vi "Database.vi"() -> ()   [LabVIEW 2016]
panel:
  in  "Tree (Right)":string[](tree)=["PPMS 2\\PPMS 2 Temperature"]
  in  "Tree (Left)":string[](tree)=["MNK_18T\\1820_IPS_Level_He", "MNK_18T\\1820_IPS_Magnet_Field"]
  in  "max points per trace (all)":i32=-1
  in  "Tab Control":enum32{"Time Traces", "X-Y Plot (shitty)"}(tab)
  out "Database Trace":T1(graph) caption="Retrieved from Citadel 5"
  in  "Y Scale.Mapping Mode\n0 = linear; 1 = log":u8
  in  "Filter?":bool
  out "XY Graph":cluster{"data":dbl[], "data":dbl[]}(graph)
  in  "Tab Control 2":T2(tab)
  in  "DST":bool caption="Blank Button"
  in  "IP or PC Name":string="HousesOfTheHoly"
  in  "Span":dbl=3600.0 step=3600.0 format="%<%D d %H hr %M min %S s>t"
  in  "Which Database?":enum16{"HousesOfTheHoly", "Rambleon"}(ring)
  in  "Mode":T3(ring)=enum."Start, End, End - T"
  in  "Display the following network shared variables (left axis)":u16[](array[ring])=[194] items=["Attocube 3DR\\axis 1: Amplitude", "Attocube 3DR\\axis 1: Capacitance", "Attocube 3DR\\axis 1: control mode", "Attocube 3DR\\axis 1: current position", "Attocube 3DR\\axis 1: DCLevel", "Attocube 3DR\\axis 1: Frequency", "Attocube 3DR\\axis 1: moving", "Attocube 3DR\\axis 1: Output", "Attocube 3DR\\axis 1: rot. count", "Attocube 3DR\\axis 1: sensor disconnected", "Attocube 3DR\\axis 1: sensor error", "Attocube 3DR\\axis 1: Single Circle Mode", "Attocube 3DR\\axis 1: sp position", "Attocube 3DR\\axis 1: sp rot count", "Attocube 3DR\\axis 1: speed", "Attocube 3DR\\axis 1: StepWidth", "Attocube 3DR\\axis 1: stop detected", "Attocube 3DR\\axis 1: stop enable", "Attocube 3DR\\axis 1: Target GND", "Attocube 3DR\\axis 2: Amplitude", "Attocube 3DR\\axis 2: Capacitance", "Attocube 3DR\\axis 2: control mode", "Attocube 3DR\\axis 2: current position", "Attocube 3DR\\axis 2: DCLevel", "Attocube 3DR\\axis 2: Frequency", "Attocube 3DR\\axis 2: moving", "Attocube 3DR\\axis 2: Output", "Attocube 3DR\\axis 2: rot. count", "Attocube 3DR\\axis 2: sensor disconnected", "Attocube 3DR\\axis 2: sensor error", "Attocube 3DR\\axis 2: Single Circle Mode", "Attocube 3DR\\axis 2: sp position", "Attocube 3DR\\axis 2: sp rot count", "Attocube 3DR\\axis 2: speed", "Attocube 3DR\\axis 2: StepWidth", "Attocube 3DR\\axis 2: stop detected", "Attocube 3DR\\axis 2: stop enable", "Attocube 3DR\\axis 2: Target GND", "Attocube 3DR\\static amplitude", "Cypher\\Cypher RH1", "Cypher\\Cypher RH2", "Cypher\\Cypher Temperature", "Cypher\\Cypher_Funnel_Property", "Cypher\\Cypher_Path_Property", "Cypher\\Cypher_Rectangle_Property", "DR200\\DR200_Magnet_Field", "DR200\\DR200_Magnet_Field_Target", "DR200\\DR200_Magnet_PS_Current", "DR200\\DR200_Magnet_PS_Field", "DR200\\DR200_Magnet_PS_Voltage", "DR200\\DR200_Magnet_Rate_Target", "DR200\\DR200_Magnet_Status_Activity", "DR200\\DR200_Magnet_Status_Mode", "DR200\\DR200_Magnet_Status_Switch_Heater", "DR200\\DR200_Magnet_Status_System", "JLevy\\Levy 1", "Leiden CF900\\CF Impedance CMN", "Leiden CF900\\CF_FP_STATE", "Leiden CF900\\CF_KH_ch1", "Leiden CF900\\CF_KH_ch2", "Leiden CF900\\CF_KH_ch3", "Leiden CF900\\CF_KH_ch4", "Leiden CF900\\CF_KH_ch5", "Leiden CF900\\CF_KH_ch6", "Leiden CF900\\CF_KH_ch7", "Leiden CF900\\CF_KH_ch8", "Leiden CF900\\CF_TC_calibration", "Leiden CF900\\CF_TC_description", "Leiden CF900\\CF_TC_Z_calibration", "Leiden CF900\\CF_TC_Z_description", "Leiden CF900\\CF_TC_Z_R0", "Leiden CF900\\CF_TC_Z_R1", "Leiden CF900\\CF_TC_Z_R2", "Leiden CF900\\CF_TC_Z_R3", "Leiden CF900\\CF_TC_Z_R4", "Leiden CF900\\CF_TC_Z_R5", "Leiden CF900\\CF_TC_Z_R6", "Leiden CF900\\CF_TC_Z_R7", "Leiden CF900\\CF_TC_Z_R8", "Leiden CF900\\CF_TC_Z_R9", "Leiden CF900\\CF_TC_Z_T0", "Leiden CF900\\CF_TC_Z_T1", "Leiden CF900\\CF_TC_Z_T2", "Leiden CF900\\CF_TC_Z_T3", "Leiden CF900\\CF_TC_Z_T4", "Leiden CF900\\CF_TC_Z_T5", "Leiden CF900\\CF_TC_Z_T6", "Leiden CF900\\CF_TC_Z_T7", "Leiden CF900\\CF_TC_Z_T8", "Leiden CF900\\CF_TC_Z_T9", "Leiden CF900\\CF900_Cstill", "Leiden CF900\\Leiden CF FP\\CF FP Flow", "Leiden CF900\\Leiden CF FP\\CF FP He", "Leiden CF900\\Leiden CF FP\\CF FP MG0", "Leiden CF900\\Leiden CF FP\\CF FP MG1", "Leiden CF900\\Leiden CF FP\\CF FP MG2", "Leiden CF900\\Leiden CF FP\\CF FP MG3", "Leiden CF900\\Leiden CF FP\\CF FP MG4", "Leiden CF900\\Leiden CF FP\\CF FP MG5", "Leiden CF900\\Leiden CF FP\\CF FP oil", "Leiden CF900\\Leiden CF FP\\CF FP P_high", "Leiden CF900\\Leiden CF FP\\CF FP P_low", "Leiden CF900\\Leiden CF FP\\CF FP P1", "Leiden CF900\\Leiden CF FP\\CF FP P2", "Leiden CF900\\Leiden CF FP\\CF FP P3", "Leiden CF900\\Leiden CF FP\\CF FP P4", "Leiden CF900\\Leiden CF FP\\CF FP P5", "Leiden CF900\\Leiden CF FP\\CF FP P6", "Leiden CF900\\Leiden CF FP\\CF FP P7", "Leiden CF900\\Leiden CF FP\\CF FP PT current", "Leiden CF900\\Leiden CF FP\\CF FP PT on", "Leiden CF900\\Leiden CF FP\\CF FP State0", "Leiden CF900\\Leiden CF FP\\CF FP State1", "Leiden CF900\\Leiden CF FP\\CF FP State2", "Leiden CF900\\Leiden CF FP\\CF FP W_in", "Leiden CF900\\Leiden CF FP\\CF FP W_out", "Leiden CF900\\Leiden CF Impedance Bridge\\CF IB TA", "Leiden CF900\\Leiden CF Impedance Bridge\\CF IB TB", "Leiden CF900\\Leiden CF Impedance Bridge\\CF IB TC", "Leiden CF900\\Leiden CF Impedance Bridge\\CF IB TD", "Leiden CF900\\Leiden CF Impedance Bridge\\CF IB TE", "Leiden CF900\\Leiden CF Magnetic Field\\CF Field X", "Leiden CF900\\Leiden CF Magnetic Field\\CF Field Y", "Leiden CF900\\Leiden CF Magnetic Field\\CF Field Z", "Leiden CF900\\Leiden CF TC\\CF TC I0", "Leiden CF900\\Leiden CF TC\\CF TC I1", "Leiden CF900\\Leiden CF TC\\CF TC I2", "Leiden CF900\\Leiden CF TC\\CF TC I3", "Leiden CF900\\Leiden CF TC\\CF TC R0", "Leiden CF900\\Leiden CF TC\\CF TC R1", "Leiden CF900\\Leiden CF TC\\CF TC R2", "Leiden CF900\\Leiden CF TC\\CF TC R3", "Leiden CF900\\Leiden CF TC\\CF TC R4", "Leiden CF900\\Leiden CF TC\\CF TC R5", "Leiden CF900\\Leiden CF TC\\CF TC R6", "Leiden CF900\\Leiden CF TC\\CF TC R7", "Leiden CF900\\Leiden CF TC\\CF TC T0", "Leiden CF900\\Leiden CF TC\\CF TC T1", "Leiden CF900\\Leiden CF TC\\CF TC T2", "Leiden CF900\\Leiden CF TC\\CF TC T3", "Leiden CF900\\Leiden CF TC\\CF TC T4", "Leiden CF900\\Leiden CF TC\\CF TC T5", "Leiden CF900\\Leiden CF TC\\CF TC T6", "Leiden CF900\\Leiden CF TC\\CF TC T7", "Leiden CF900\\RuO2_T", "Leiden CF900\\RuO2_Z", "Leiden CF900\\Vbg", "Leiden CF900\\VRM VrmSweepMode", "Leiden CF900\\VRM VrmSweepRate", "Leiden CF900\\VRM VrmSweepTime", "Leiden CF900\\VRM VrmX setpT", "Leiden CF900\\VRM VrmY setpT", "Leiden CF900\\VRM VrmZ setpT", "Leiden CF900\\VRM X at rest", "Leiden CF900\\VRM X magA", "Leiden CF900\\VRM X magT", "Leiden CF900\\VRM X meas A", "Leiden CF900\\VRM X meas V", "Leiden CF900\\VRM X outA", "Leiden CF900\\VRM X outT", "Leiden CF900\\VRM X setpT", "Leiden CF900\\VRM X Status", "Leiden CF900\\VRM X sweep", "Leiden CF900\\VRM X sweep A", "Leiden CF900\\VRM Y at rest", "Leiden CF900\\VRM Y magA", "Leiden CF900\\VRM Y magT", "Leiden CF900\\VRM Y meas A", "Leiden CF900\\VRM Y meas V", "Leiden CF900\\VRM Y outA", "Leiden CF900\\VRM Y outT", "Leiden CF900\\VRM Y setpT", "Leiden CF900\\VRM Y Status", "Leiden CF900\\VRM Y sweep", "Leiden CF900\\VRM Y sweep A", "Leiden CF900\\VRM Z at rest", "Leiden CF900\\VRM Z magA", "Leiden CF900\\VRM Z magT", "Leiden CF900\\VRM Z meas A", "Leiden CF900\\VRM Z meas V", "Leiden CF900\\VRM Z outA", "Leiden CF900\\VRM Z outT", "Leiden CF900\\VRM Z setpT", "Leiden CF900\\VRM Z Status", "Leiden CF900\\VRM Z sweep", "Leiden CF900\\VRM Z sweep A", "MFP3D\\MFP3D Hum", "MFP3D\\MFP3D Temperature", "MFP3D\\MFP3D TSP01 Hum", "MFP3D\\MFP3D TSP01 Temperature", "MFP3D\\MFP3D User", "MNK_18T\\1820_IPS_Current", "MNK_18T\\1820_IPS_Level_He", "MNK_18T\\1820_IPS_Level_N2", "MNK_18T\\1820_IPS_M1_Current", "MNK_18T\\1820_IPS_M1_Voltage", "MNK_18T\\1820_IPS_M2_Current", "MNK_18T\\1820_IPS_M2_Voltage", "MNK_18T\\1820_IPS_M3_Current", "MNK_18T\\1820_IPS_M3_Voltage", "MNK_18T\\1820_IPS_Magnet_Field", "MNK_18T\\1820_IPS_Magnet_Temperature", "MNK_18T\\1820_IPS_Magnet_Temperature_R", "MNK_18T\\1820_IPS_PS_Field", "MNK_18T\\1820_IPS_Reply", "MNK_18T\\1820_IPS_Status", "MNK_18T\\1820_IPS_Switch", "MNK_18T\\1820_IPS_Target_Field", "MNK_18T\\1820_IPS_Target_Field_Rate", "MNK_18T\\1820_IPS_Voltage", "MNK_18T\\1820_ITC_Lambda_Status", "MNK_18T\\1820_ITC_Lambda_Temperature", "MNK_18T\\1820_ITC_Lambda_Temperature_R", "MNK_18T\\1820_ITC_Needle_Valve", "MNK_18T\\1820_ITC_Pressure", "MNK_18T\\1820_ITC_Reply", "MNK_18T\\KH_ch1", "MNK_18T\\KH_ch2", "MNK_18T\\KH_ch3", "MNK_18T\\KH_ch4", "MNK_18T\\KH_ch5", "MNK_18T\\KH_ch6", "MNK_18T\\KH_ch7", "MNK_18T\\KH_ch8", "MNK_18T\\Lockin_Results", "MNK_18T\\MNK_CMN-187_T", "MNK_18T\\MNK_CMN-187_Z", "MNK_18T\\MNK_Cstill_T", "MNK_18T\\MNK_Cstill_Z", "MNK_18T\\MNK_FP_Flow", "MNK_18T\\MNK_FP_MG0", "MNK_18T\\MNK_FP_MG1", "MNK_18T\\MNK_FP_MG2", "MNK_18T\\MNK_FP_MG3", "MNK_18T\\MNK_FP_MG4", "MNK_18T\\MNK_FP_MG5", "MNK_18T\\MNK_FP_P1", "MNK_18T\\MNK_FP_P2", "MNK_18T\\MNK_FP_P3", "MNK_18T\\MNK_FP_P4", "MNK_18T\\MNK_FP_P5", "MNK_18T\\MNK_FP_P6", "MNK_18T\\MNK_FP_P7", "MNK_18T\\MNK_FP_STATE", "MNK_18T\\MNK_FP_State0", "MNK_18T\\MNK_FP_State1", "MNK_18T\\MNK_FP_State2", "MNK_18T\\MNK_TC_calibration", "MNK_18T\\MNK_TC_description", "MNK_18T\\MNK_TC_I0", "MNK_18T\\MNK_TC_I1", "MNK_18T\\MNK_TC_I2", "MNK_18T\\MNK_TC_I3", "MNK_18T\\MNK_TC_R0", "MNK_18T\\MNK_TC_R1", "MNK_18T\\MNK_TC_R2", "MNK_18T\\MNK_TC_R3", "MNK_18T\\MNK_TC_R4", "MNK_18T\\MNK_TC_R5", "MNK_18T\\MNK_TC_R6", "MNK_18T\\MNK_TC_R7", "MNK_18T\\MNK_TC_T0", "MNK_18T\\MNK_TC_T1", "MNK_18T\\MNK_TC_T2", "MNK_18T\\MNK_TC_T3", "MNK_18T\\MNK_TC_T4", "MNK_18T\\MNK_TC_T5", "MNK_18T\\MNK_TC_T6", "MNK_18T\\MNK_TC_T7", "MNK_18T\\MNK_TC_Z_calibration", "MNK_18T\\MNK_TC_Z_description", "MNK_18T\\OSC_config", "MNK_18T\\Vbg", "Montana THZ 1\\THZ 1 Dew Point", "Montana THZ 1\\THZ 1 Humidity", "Montana THZ 1\\THZ 1 Temperature", "OneNote API HTTP\\Access Token 0000000048124379", "OneNote API HTTP\\Asana Access Token 15669051163913", "PPMS 1\\PPMS 1 Magnetic Field", "PPMS 1\\PPMS 1 Temperature", "PPMS 2\\PPMS 2 Flow Rate", "PPMS 2\\PPMS 2 Helium Level", "PPMS 2\\PPMS 2 Magnetic Field", "PPMS 2\\PPMS 2 Position", "PPMS 2\\PPMS 2 Sys Pressure", "PPMS 2\\PPMS 2 Temperature", "PPMS 2\\PPMS 2 Vbg", "PPMS2\\PPMS2 Annulus Pres (Torr)", "PPMS2\\PPMS2 Annulus Vacuum (V)", "PPMS2\\PPMS2 Block Htr Cur (mA)", "PPMS2\\PPMS2 Block Htr Pwr (W)", "PPMS2\\PPMS2 BlockHeater(Ohm)", "PPMS2\\PPMS2 Bridge 1 Excitation (uA)", "PPMS2\\PPMS2 Bridge 1 Resistance (ohms)", "PPMS2\\PPMS2 Bridge 2 Excitation (uA)", "PPMS2\\PPMS2 Bridge 2 Resistance (ohms)", "PPMS2\\PPMS2 Bridge 3 Excitation (uA)", "PPMS2\\PPMS2 Bridge 3 Resistance (ohms)", "PPMS2\\PPMS2 Bridge 4 Excitation (uA)", "PPMS2\\PPMS2 Bridge 4 Resistance (ohms)", "PPMS2\\PPMS2 CIG Cernox (K)", "PPMS2\\PPMS2 CIG Excit (uA)", "PPMS2\\PPMS2 Comment", "PPMS2\\PPMS2 DAC  I  (cnts)", "PPMS2\\PPMS2 Digital Inputs (code)", "PPMS2\\PPMS2 Drive 1 Iout (mA)", "PPMS2\\PPMS2 Drive 1 Ipower (watts)", "PPMS2\\PPMS2 Drive 2 Iout (mA)", "PPMS2\\PPMS2 Drive 2 Ipower (watts)", "PPMS2\\PPMS2 EXT Flow (L min)", "PPMS2\\PPMS2 Flapper state", "PPMS2\\PPMS2 Flow Rate (l min)", "PPMS2\\PPMS2 He Level ()", "PPMS2\\PPMS2 Hi res (A) read", "PPMS2\\PPMS2 High Vacuum mode", "PPMS2\\PPMS2 Hires enable", "PPMS2\\PPMS2 Impedance (mode)", "PPMS2\\PPMS2 iso flag", "PPMS2\\PPMS2 KRPMs", "PPMS2\\PPMS2 Last 2 eng st", "PPMS2\\PPMS2 Log", "PPMS2\\PPMS2 Mag (V) read", "PPMS2\\PPMS2 Mag (V) set", "PPMS2\\PPMS2 Mag adj sc(I)set", "PPMS2\\PPMS2 Magnet (Oe)", "PPMS2\\PPMS2 Magnetic Field (Oe)", "PPMS2\\PPMS2 Map 20 ()", "PPMS2\\PPMS2 Map 21 ()", "PPMS2\\PPMS2 Map 22 ()", "PPMS2\\PPMS2 Map 23 ()", "PPMS2\\PPMS2 Map 24 ()", "PPMS2\\PPMS2 Map 25 ()", "PPMS2\\PPMS2 Map 26 ()", "PPMS2\\PPMS2 Map 27 ()", "PPMS2\\PPMS2 Map 28 ()", "PPMS2\\PPMS2 Map 29 ()", "PPMS2\\PPMS2 Map 67 ()", "PPMS2\\PPMS2 Map 68 ()", "PPMS2\\PPMS2 Map 69 ()", "PPMS2\\PPMS2 Map 89 ()", "PPMS2\\PPMS2 Map 90 ()", "PPMS2\\PPMS2 Map 91 ()", "PPMS2\\PPMS2 Map 92 ()", "PPMS2\\PPMS2 Map 93 ()", "PPMS2\\PPMS2 Neck Excit (uA)", "PPMS2\\PPMS2 Neck Htr Cur (mA)", "PPMS2\\PPMS2 Neck Htr Pwr (W)", "PPMS2\\PPMS2 Neck Therm (K)", "PPMS2\\PPMS2 NeckHeater(Ohm)", "PPMS2\\PPMS2 Plat Excit (uA)", "PPMS2\\PPMS2 Plat Therm (K)", "PPMS2\\PPMS2 Pressure ()", "PPMS2\\PPMS2 PSU Field (Oe)", "PPMS2\\PPMS2 Pump power (W)", "PPMS2\\PPMS2 Pump temp (C)", "PPMS2\\PPMS2 Redirected 55 ()", "PPMS2\\PPMS2 Redirected 56 ()", "PPMS2\\PPMS2 Redirected 57 ()", "PPMS2\\PPMS2 Redirected 58 ()", "PPMS2\\PPMS2 Redirected 59 ()", "PPMS2\\PPMS2 Redirected 61 ()", "PPMS2\\PPMS2 Regen htr flag", "PPMS2\\PPMS2 Sample Position (deg)", "PPMS2\\PPMS2 Seq Stat ()", "PPMS2\\PPMS2 Setpoint (K)", "PPMS2\\PPMS2 Signal 1 Vin (V)", "PPMS2\\PPMS2 Signal 2 Vin (V)", "PPMS2\\PPMS2 Spare Excit (uA)", "PPMS2\\PPMS2 Spare Therm (K)", "PPMS2\\PPMS2 Status (code)", "PPMS2\\PPMS2 Sw heater state", "PPMS2\\PPMS2 Sys Temp ()", "PPMS2\\PPMS2 System Pres (Torr)", "PPMS2\\PPMS2 System Status (code)", "PPMS2\\PPMS2 Tableless Map53 ()", "PPMS2\\PPMS2 Tableless Map54 ()", "PPMS2\\PPMS2 Temperature (K)", "PPMS2\\PPMS2 Therm v", "PPMS2\\PPMS2 Time Stamp (sec)", "PPMS2\\PPMS2 Valve Position (deg)", "PPMSDR\\PPMSDR Annulus Pres (Torr)", "PPMSDR\\PPMSDR Annulus Vacuum (V)", "PPMSDR\\PPMSDR Block Htr Cur (mA)", "PPMSDR\\PPMSDR Block Htr Pwr (W)", "PPMSDR\\PPMSDR BlockHeater(Ohm)", "PPMSDR\\PPMSDR Bridge 1 Excitation (uA)", "PPMSDR\\PPMSDR Bridge 1 Resistance (ohms)", "PPMSDR\\PPMSDR Bridge 2 Excitation (uA)", "PPMSDR\\PPMSDR Bridge 2 Resistance (ohms)", "PPMSDR\\PPMSDR Bridge 3 Excitation (uA)", "PPMSDR\\PPMSDR Bridge 3 Resistance (ohms)", "PPMSDR\\PPMSDR Bridge 4 Excitation (uA)", "PPMSDR\\PPMSDR Bridge 4 Resistance (ohms)", "PPMSDR\\PPMSDR CIG Cernox (K)", "PPMSDR\\PPMSDR CIG Excit (uA)", "PPMSDR\\PPMSDR Comment", "PPMSDR\\PPMSDR DAC  I  (cnts)", "PPMSDR\\PPMSDR Digital Inputs (code)", "PPMSDR\\PPMSDR Drive 1 Iout (mA)", "PPMSDR\\PPMSDR Drive 1 Ipower (watts)", "PPMSDR\\PPMSDR Drive 2 Iout (mA)", "PPMSDR\\PPMSDR Drive 2 Ipower (watts)", "PPMSDR\\PPMSDR EXT Flow (L min)", "PPMSDR\\PPMSDR Flapper state", "PPMSDR\\PPMSDR Flow Rate (l min)", "PPMSDR\\PPMSDR He Level ()", "PPMSDR\\PPMSDR Hi res (A) read", "PPMSDR\\PPMSDR High Vacuum mode", "PPMSDR\\PPMSDR Hires enable", "PPMSDR\\PPMSDR Impedance (mode)", "PPMSDR\\PPMSDR iso flag", "PPMSDR\\PPMSDR KRPMs", "PPMSDR\\PPMSDR Last 2 eng st", "PPMSDR\\PPMSDR Log", "PPMSDR\\PPMSDR low res (A) read", "PPMSDR\\PPMSDR Mag (V) read", "PPMSDR\\PPMSDR Mag (V) set", "PPMSDR\\PPMSDR Mag adj sc(I)set", "PPMSDR\\PPMSDR Magnet (Oe)", "PPMSDR\\PPMSDR Magnetic Field (Oe)", "PPMSDR\\PPMSDR MAP 1", "PPMSDR\\PPMSDR MAP 10", "PPMSDR\\PPMSDR MAP 11", "PPMSDR\\PPMSDR MAP 12", "PPMSDR\\PPMSDR MAP 13", "PPMSDR\\PPMSDR MAP 14", "PPMSDR\\PPMSDR MAP 15", "PPMSDR\\PPMSDR MAP 16", "PPMSDR\\PPMSDR MAP 17", "PPMSDR\\PPMSDR MAP 18", "PPMSDR\\PPMSDR MAP 19", "PPMSDR\\PPMSDR MAP 2", "PPMSDR\\PPMSDR MAP 20", "PPMSDR\\PPMSDR Map 20 ()", "PPMSDR\\PPMSDR MAP 21", "PPMSDR\\PPMSDR Map 21 ()", "PPMSDR\\PPMSDR MAP 22", "PPMSDR\\PPMSDR Map 22 ()", "PPMSDR\\PPMSDR MAP 23", "PPMSDR\\PPMSDR Map 23 ()", "PPMSDR\\PPMSDR MAP 24", "PPMSDR\\PPMSDR Map 24 ()", "PPMSDR\\PPMSDR MAP 25", "PPMSDR\\PPMSDR Map 25 ()", "PPMSDR\\PPMSDR MAP 26", "PPMSDR\\PPMSDR Map 26 ()", "PPMSDR\\PPMSDR MAP 27", "PPMSDR\\PPMSDR Map 27 ()", "PPMSDR\\PPMSDR MAP 28", "PPMSDR\\PPMSDR Map 28 ()", "PPMSDR\\PPMSDR MAP 29", "PPMSDR\\PPMSDR Map 29 ()", "PPMSDR\\PPMSDR MAP 3", "PPMSDR\\PPMSDR MAP 30", "PPMSDR\\PPMSDR MAP 4", "PPMSDR\\PPMSDR MAP 5", "PPMSDR\\PPMSDR MAP 6", "PPMSDR\\PPMSDR Map 67 ()", "PPMSDR\\PPMSDR Map 68 ()", "PPMSDR\\PPMSDR Map 69 ()", "PPMSDR\\PPMSDR MAP 7", "PPMSDR\\PPMSDR MAP 8", "PPMSDR\\PPMSDR Map 89 ()", "PPMSDR\\PPMSDR MAP 9", "PPMSDR\\PPMSDR Map 90 ()", "PPMSDR\\PPMSDR Map 91 ()", "PPMSDR\\PPMSDR Map 92 ()", "PPMSDR\\PPMSDR Map 93 ()", "PPMSDR\\PPMSDR Neck Excit (uA)", "PPMSDR\\PPMSDR Neck Htr Cur (mA)", "PPMSDR\\PPMSDR Neck Htr Pwr (W)", "PPMSDR\\PPMSDR Neck Therm (K)", "PPMSDR\\PPMSDR NeckHeater(Ohm)", "PPMSDR\\PPMSDR Plat Excit (uA)", "PPMSDR\\PPMSDR Plat Therm (K)", "PPMSDR\\PPMSDR Pressure ()", "PPMSDR\\PPMSDR Pump power (W)", "PPMSDR\\PPMSDR Pump temp (C)", "PPMSDR\\PPMSDR Redirected 55 ()", "PPMSDR\\PPMSDR Redirected 56 ()", "PPMSDR\\PPMSDR Redirected 57 ()", "PPMSDR\\PPMSDR Redirected 58 ()", "PPMSDR\\PPMSDR Redirected 59 ()", "PPMSDR\\PPMSDR Redirected 61 ()", "PPMSDR\\PPMSDR Regen htr flag", "PPMSDR\\PPMSDR Sample Position (deg)", "PPMSDR\\PPMSDR Seq Stat ()", "PPMSDR\\PPMSDR Setpoint (K)", "PPMSDR\\PPMSDR Signal 1 Vin (V)", "PPMSDR\\PPMSDR Signal 2 Vin (V)", "PPMSDR\\PPMSDR Spare Excit (uA)", "PPMSDR\\PPMSDR Spare Therm (K)", "PPMSDR\\PPMSDR Status (code)", "PPMSDR\\PPMSDR Sw heater state", "PPMSDR\\PPMSDR Sys Temp ()", "PPMSDR\\PPMSDR System Pres (Torr)", "PPMSDR\\PPMSDR System Status (code)", "PPMSDR\\PPMSDR Tableless Map53 ()", "PPMSDR\\PPMSDR Tableless Map54 ()", "PPMSDR\\PPMSDR Temperature (K)", "PPMSDR\\PPMSDR Therm v", "PPMSDR\\PPMSDR Time Stamp (sec)", "PPMSDR\\PPMSDR Valve Position (deg)", "Sample Characterization\\2G Conductance", "Sample Characterization\\4G", "Sample Characterization\\4R", "Sample Characterization\\CURRENT", "Sample Characterization\\Experiment ID", "Sample Characterization\\Notes", "Sample Characterization\\OSCILLATION VOLTAGE", "Sample Characterization\\Sample Name", "Sample Characterization\\V1", "Sample Characterization\\V2", "SPM\\Laser Power", "SPM\\SPM scanner X", "SPM\\SPM scanner Y", "TEMPerHUM\\MFP : Humidity", "TEMPerHUM\\MFP : ID", "TEMPerHUM\\MFP : Location", "TEMPerHUM\\MFP : Picture URL", "TEMPerHUM\\MFP : Temperature", "TEMPerHUM\\MFP-3D : Humidity", "TEMPerHUM\\MFP-3D : ID", "TEMPerHUM\\MFP-3D : Location", "TEMPerHUM\\MFP-3D : Picture URL", "TEMPerHUM\\MFP-3D : Temperature", "TEMPerHUM\\TEST3 : Humidity", "TEMPerHUM\\TEST3 : ID", "TEMPerHUM\\TEST3 : Location", "TEMPerHUM\\TEST3 : Picture URL", "TEMPerHUM\\TEST3 : Temperature"]
  in  "Display the following network shared variables (right axis)":u16[](array[ring])=[192] items=["Attocube 3DR\\axis 1: Amplitude", "Attocube 3DR\\axis 1: Capacitance", "Attocube 3DR\\axis 1: control mode", "Attocube 3DR\\axis 1: current position", "Attocube 3DR\\axis 1: DCLevel", "Attocube 3DR\\axis 1: Frequency", "Attocube 3DR\\axis 1: moving", "Attocube 3DR\\axis 1: Output", "Attocube 3DR\\axis 1: rot. count", "Attocube 3DR\\axis 1: sensor disconnected", "Attocube 3DR\\axis 1: sensor error", "Attocube 3DR\\axis 1: Single Circle Mode", "Attocube 3DR\\axis 1: sp position", "Attocube 3DR\\axis 1: sp rot count", "Attocube 3DR\\axis 1: speed", "Attocube 3DR\\axis 1: StepWidth", "Attocube 3DR\\axis 1: stop detected", "Attocube 3DR\\axis 1: stop enable", "Attocube 3DR\\axis 1: Target GND", "Attocube 3DR\\axis 2: Amplitude", "Attocube 3DR\\axis 2: Capacitance", "Attocube 3DR\\axis 2: control mode", "Attocube 3DR\\axis 2: current position", "Attocube 3DR\\axis 2: DCLevel", "Attocube 3DR\\axis 2: Frequency", "Attocube 3DR\\axis 2: moving", "Attocube 3DR\\axis 2: Output", "Attocube 3DR\\axis 2: rot. count", "Attocube 3DR\\axis 2: sensor disconnected", "Attocube 3DR\\axis 2: sensor error", "Attocube 3DR\\axis 2: Single Circle Mode", "Attocube 3DR\\axis 2: sp position", "Attocube 3DR\\axis 2: sp rot count", "Attocube 3DR\\axis 2: speed", "Attocube 3DR\\axis 2: StepWidth", "Attocube 3DR\\axis 2: stop detected", "Attocube 3DR\\axis 2: stop enable", "Attocube 3DR\\axis 2: Target GND", "Attocube 3DR\\static amplitude", "Cypher\\Cypher RH1", "Cypher\\Cypher RH2", "Cypher\\Cypher Temperature", "Cypher\\Cypher_Funnel_Property", "Cypher\\Cypher_Path_Property", "Cypher\\Cypher_Rectangle_Property", "DR200\\DR200_Magnet_Field", "DR200\\DR200_Magnet_Field_Target", "DR200\\DR200_Magnet_PS_Current", "DR200\\DR200_Magnet_PS_Field", "DR200\\DR200_Magnet_PS_Voltage", "DR200\\DR200_Magnet_Rate_Target", "DR200\\DR200_Magnet_Status_Activity", "DR200\\DR200_Magnet_Status_Mode", "DR200\\DR200_Magnet_Status_Switch_Heater", "DR200\\DR200_Magnet_Status_System", "JLevy\\Levy 1", "Leiden CF900\\CF Impedance CMN", "Leiden CF900\\CF_FP_STATE", "Leiden CF900\\CF_KH_ch1", "Leiden CF900\\CF_KH_ch2", "Leiden CF900\\CF_KH_ch3", "Leiden CF900\\CF_KH_ch4", "Leiden CF900\\CF_KH_ch5", "Leiden CF900\\CF_KH_ch6", "Leiden CF900\\CF_KH_ch7", "Leiden CF900\\CF_KH_ch8", "Leiden CF900\\CF_TC_calibration", "Leiden CF900\\CF_TC_description", "Leiden CF900\\CF_TC_Z_calibration", "Leiden CF900\\CF_TC_Z_description", "Leiden CF900\\CF_TC_Z_R0", "Leiden CF900\\CF_TC_Z_R1", "Leiden CF900\\CF_TC_Z_R2", "Leiden CF900\\CF_TC_Z_R3", "Leiden CF900\\CF_TC_Z_R4", "Leiden CF900\\CF_TC_Z_R5", "Leiden CF900\\CF_TC_Z_R6", "Leiden CF900\\CF_TC_Z_R7", "Leiden CF900\\CF_TC_Z_R8", "Leiden CF900\\CF_TC_Z_R9", "Leiden CF900\\CF_TC_Z_T0", "Leiden CF900\\CF_TC_Z_T1", "Leiden CF900\\CF_TC_Z_T2", "Leiden CF900\\CF_TC_Z_T3", "Leiden CF900\\CF_TC_Z_T4", "Leiden CF900\\CF_TC_Z_T5", "Leiden CF900\\CF_TC_Z_T6", "Leiden CF900\\CF_TC_Z_T7", "Leiden CF900\\CF_TC_Z_T8", "Leiden CF900\\CF_TC_Z_T9", "Leiden CF900\\CF900_Cstill", "Leiden CF900\\Leiden CF FP\\CF FP Flow", "Leiden CF900\\Leiden CF FP\\CF FP He", "Leiden CF900\\Leiden CF FP\\CF FP MG0", "Leiden CF900\\Leiden CF FP\\CF FP MG1", "Leiden CF900\\Leiden CF FP\\CF FP MG2", "Leiden CF900\\Leiden CF FP\\CF FP MG3", "Leiden CF900\\Leiden CF FP\\CF FP MG4", "Leiden CF900\\Leiden CF FP\\CF FP MG5", "Leiden CF900\\Leiden CF FP\\CF FP oil", "Leiden CF900\\Leiden CF FP\\CF FP P_high", "Leiden CF900\\Leiden CF FP\\CF FP P_low", "Leiden CF900\\Leiden CF FP\\CF FP P1", "Leiden CF900\\Leiden CF FP\\CF FP P2", "Leiden CF900\\Leiden CF FP\\CF FP P3", "Leiden CF900\\Leiden CF FP\\CF FP P4", "Leiden CF900\\Leiden CF FP\\CF FP P5", "Leiden CF900\\Leiden CF FP\\CF FP P6", "Leiden CF900\\Leiden CF FP\\CF FP P7", "Leiden CF900\\Leiden CF FP\\CF FP PT current", "Leiden CF900\\Leiden CF FP\\CF FP PT on", "Leiden CF900\\Leiden CF FP\\CF FP State0", "Leiden CF900\\Leiden CF FP\\CF FP State1", "Leiden CF900\\Leiden CF FP\\CF FP State2", "Leiden CF900\\Leiden CF FP\\CF FP W_in", "Leiden CF900\\Leiden CF FP\\CF FP W_out", "Leiden CF900\\Leiden CF Impedance Bridge\\CF IB TA", "Leiden CF900\\Leiden CF Impedance Bridge\\CF IB TB", "Leiden CF900\\Leiden CF Impedance Bridge\\CF IB TC", "Leiden CF900\\Leiden CF Impedance Bridge\\CF IB TD", "Leiden CF900\\Leiden CF Impedance Bridge\\CF IB TE", "Leiden CF900\\Leiden CF Magnetic Field\\CF Field X", "Leiden CF900\\Leiden CF Magnetic Field\\CF Field Y", "Leiden CF900\\Leiden CF Magnetic Field\\CF Field Z", "Leiden CF900\\Leiden CF TC\\CF TC I0", "Leiden CF900\\Leiden CF TC\\CF TC I1", "Leiden CF900\\Leiden CF TC\\CF TC I2", "Leiden CF900\\Leiden CF TC\\CF TC I3", "Leiden CF900\\Leiden CF TC\\CF TC R0", "Leiden CF900\\Leiden CF TC\\CF TC R1", "Leiden CF900\\Leiden CF TC\\CF TC R2", "Leiden CF900\\Leiden CF TC\\CF TC R3", "Leiden CF900\\Leiden CF TC\\CF TC R4", "Leiden CF900\\Leiden CF TC\\CF TC R5", "Leiden CF900\\Leiden CF TC\\CF TC R6", "Leiden CF900\\Leiden CF TC\\CF TC R7", "Leiden CF900\\Leiden CF TC\\CF TC T0", "Leiden CF900\\Leiden CF TC\\CF TC T1", "Leiden CF900\\Leiden CF TC\\CF TC T2", "Leiden CF900\\Leiden CF TC\\CF TC T3", "Leiden CF900\\Leiden CF TC\\CF TC T4", "Leiden CF900\\Leiden CF TC\\CF TC T5", "Leiden CF900\\Leiden CF TC\\CF TC T6", "Leiden CF900\\Leiden CF TC\\CF TC T7", "Leiden CF900\\RuO2_T", "Leiden CF900\\RuO2_Z", "Leiden CF900\\Vbg", "Leiden CF900\\VRM VrmSweepMode", "Leiden CF900\\VRM VrmSweepRate", "Leiden CF900\\VRM VrmSweepTime", "Leiden CF900\\VRM VrmX setpT", "Leiden CF900\\VRM VrmY setpT", "Leiden CF900\\VRM VrmZ setpT", "Leiden CF900\\VRM X at rest", "Leiden CF900\\VRM X magA", "Leiden CF900\\VRM X magT", "Leiden CF900\\VRM X meas A", "Leiden CF900\\VRM X meas V", "Leiden CF900\\VRM X outA", "Leiden CF900\\VRM X outT", "Leiden CF900\\VRM X setpT", "Leiden CF900\\VRM X Status", "Leiden CF900\\VRM X sweep", "Leiden CF900\\VRM X sweep A", "Leiden CF900\\VRM Y at rest", "Leiden CF900\\VRM Y magA", "Leiden CF900\\VRM Y magT", "Leiden CF900\\VRM Y meas A", "Leiden CF900\\VRM Y meas V", "Leiden CF900\\VRM Y outA", "Leiden CF900\\VRM Y outT", "Leiden CF900\\VRM Y setpT", "Leiden CF900\\VRM Y Status", "Leiden CF900\\VRM Y sweep", "Leiden CF900\\VRM Y sweep A", "Leiden CF900\\VRM Z at rest", "Leiden CF900\\VRM Z magA", "Leiden CF900\\VRM Z magT", "Leiden CF900\\VRM Z meas A", "Leiden CF900\\VRM Z meas V", "Leiden CF900\\VRM Z outA", "Leiden CF900\\VRM Z outT", "Leiden CF900\\VRM Z setpT", "Leiden CF900\\VRM Z Status", "Leiden CF900\\VRM Z sweep", "Leiden CF900\\VRM Z sweep A", "MFP3D\\MFP3D Hum", "MFP3D\\MFP3D Temperature", "MFP3D\\MFP3D TSP01 Hum", "MFP3D\\MFP3D TSP01 Temperature", "MFP3D\\MFP3D User", "MNK_18T\\1820_IPS_Current", "MNK_18T\\1820_IPS_Level_He", "MNK_18T\\1820_IPS_Level_N2", "MNK_18T\\1820_IPS_M1_Current", "MNK_18T\\1820_IPS_M1_Voltage", "MNK_18T\\1820_IPS_M2_Current", "MNK_18T\\1820_IPS_M2_Voltage", "MNK_18T\\1820_IPS_M3_Current", "MNK_18T\\1820_IPS_M3_Voltage", "MNK_18T\\1820_IPS_Magnet_Field", "MNK_18T\\1820_IPS_Magnet_Temperature", "MNK_18T\\1820_IPS_Magnet_Temperature_R", "MNK_18T\\1820_IPS_PS_Field", "MNK_18T\\1820_IPS_Reply", "MNK_18T\\1820_IPS_Status", "MNK_18T\\1820_IPS_Switch", "MNK_18T\\1820_IPS_Target_Field", "MNK_18T\\1820_IPS_Target_Field_Rate", "MNK_18T\\1820_IPS_Voltage", "MNK_18T\\1820_ITC_Lambda_Status", "MNK_18T\\1820_ITC_Lambda_Temperature", "MNK_18T\\1820_ITC_Lambda_Temperature_R", "MNK_18T\\1820_ITC_Needle_Valve", "MNK_18T\\1820_ITC_Pressure", "MNK_18T\\1820_ITC_Reply", "MNK_18T\\KH_ch1", "MNK_18T\\KH_ch2", "MNK_18T\\KH_ch3", "MNK_18T\\KH_ch4", "MNK_18T\\KH_ch5", "MNK_18T\\KH_ch6", "MNK_18T\\KH_ch7", "MNK_18T\\KH_ch8", "MNK_18T\\Lockin_Results", "MNK_18T\\MNK_CMN-187_T", "MNK_18T\\MNK_CMN-187_Z", "MNK_18T\\MNK_Cstill_T", "MNK_18T\\MNK_Cstill_Z", "MNK_18T\\MNK_FP_Flow", "MNK_18T\\MNK_FP_MG0", "MNK_18T\\MNK_FP_MG1", "MNK_18T\\MNK_FP_MG2", "MNK_18T\\MNK_FP_MG3", "MNK_18T\\MNK_FP_MG4", "MNK_18T\\MNK_FP_MG5", "MNK_18T\\MNK_FP_P1", "MNK_18T\\MNK_FP_P2", "MNK_18T\\MNK_FP_P3", "MNK_18T\\MNK_FP_P4", "MNK_18T\\MNK_FP_P5", "MNK_18T\\MNK_FP_P6", "MNK_18T\\MNK_FP_P7", "MNK_18T\\MNK_FP_STATE", "MNK_18T\\MNK_FP_State0", "MNK_18T\\MNK_FP_State1", "MNK_18T\\MNK_FP_State2", "MNK_18T\\MNK_TC_calibration", "MNK_18T\\MNK_TC_description", "MNK_18T\\MNK_TC_I0", "MNK_18T\\MNK_TC_I1", "MNK_18T\\MNK_TC_I2", "MNK_18T\\MNK_TC_I3", "MNK_18T\\MNK_TC_R0", "MNK_18T\\MNK_TC_R1", "MNK_18T\\MNK_TC_R2", "MNK_18T\\MNK_TC_R3", "MNK_18T\\MNK_TC_R4", "MNK_18T\\MNK_TC_R5", "MNK_18T\\MNK_TC_R6", "MNK_18T\\MNK_TC_R7", "MNK_18T\\MNK_TC_T0", "MNK_18T\\MNK_TC_T1", "MNK_18T\\MNK_TC_T2", "MNK_18T\\MNK_TC_T3", "MNK_18T\\MNK_TC_T4", "MNK_18T\\MNK_TC_T5", "MNK_18T\\MNK_TC_T6", "MNK_18T\\MNK_TC_T7", "MNK_18T\\MNK_TC_Z_calibration", "MNK_18T\\MNK_TC_Z_description", "MNK_18T\\OSC_config", "MNK_18T\\Vbg", "Montana THZ 1\\THZ 1 Dew Point", "Montana THZ 1\\THZ 1 Humidity", "Montana THZ 1\\THZ 1 Temperature", "OneNote API HTTP\\Access Token 0000000048124379", "OneNote API HTTP\\Asana Access Token 15669051163913", "PPMS 1\\PPMS 1 Magnetic Field", "PPMS 1\\PPMS 1 Temperature", "PPMS 2\\PPMS 2 Flow Rate", "PPMS 2\\PPMS 2 Helium Level", "PPMS 2\\PPMS 2 Magnetic Field", "PPMS 2\\PPMS 2 Position", "PPMS 2\\PPMS 2 Sys Pressure", "PPMS 2\\PPMS 2 Temperature", "PPMS 2\\PPMS 2 Vbg", "PPMS2\\PPMS2 Annulus Pres (Torr)", "PPMS2\\PPMS2 Annulus Vacuum (V)", "PPMS2\\PPMS2 Block Htr Cur (mA)", "PPMS2\\PPMS2 Block Htr Pwr (W)", "PPMS2\\PPMS2 BlockHeater(Ohm)", "PPMS2\\PPMS2 Bridge 1 Excitation (uA)", "PPMS2\\PPMS2 Bridge 1 Resistance (ohms)", "PPMS2\\PPMS2 Bridge 2 Excitation (uA)", "PPMS2\\PPMS2 Bridge 2 Resistance (ohms)", "PPMS2\\PPMS2 Bridge 3 Excitation (uA)", "PPMS2\\PPMS2 Bridge 3 Resistance (ohms)", "PPMS2\\PPMS2 Bridge 4 Excitation (uA)", "PPMS2\\PPMS2 Bridge 4 Resistance (ohms)", "PPMS2\\PPMS2 CIG Cernox (K)", "PPMS2\\PPMS2 CIG Excit (uA)", "PPMS2\\PPMS2 Comment", "PPMS2\\PPMS2 DAC  I  (cnts)", "PPMS2\\PPMS2 Digital Inputs (code)", "PPMS2\\PPMS2 Drive 1 Iout (mA)", "PPMS2\\PPMS2 Drive 1 Ipower (watts)", "PPMS2\\PPMS2 Drive 2 Iout (mA)", "PPMS2\\PPMS2 Drive 2 Ipower (watts)", "PPMS2\\PPMS2 EXT Flow (L min)", "PPMS2\\PPMS2 Flapper state", "PPMS2\\PPMS2 Flow Rate (l min)", "PPMS2\\PPMS2 He Level ()", "PPMS2\\PPMS2 Hi res (A) read", "PPMS2\\PPMS2 High Vacuum mode", "PPMS2\\PPMS2 Hires enable", "PPMS2\\PPMS2 Impedance (mode)", "PPMS2\\PPMS2 iso flag", "PPMS2\\PPMS2 KRPMs", "PPMS2\\PPMS2 Last 2 eng st", "PPMS2\\PPMS2 Log", "PPMS2\\PPMS2 Mag (V) read", "PPMS2\\PPMS2 Mag (V) set", "PPMS2\\PPMS2 Mag adj sc(I)set", "PPMS2\\PPMS2 Magnet (Oe)", "PPMS2\\PPMS2 Magnetic Field (Oe)", "PPMS2\\PPMS2 Map 20 ()", "PPMS2\\PPMS2 Map 21 ()", "PPMS2\\PPMS2 Map 22 ()", "PPMS2\\PPMS2 Map 23 ()", "PPMS2\\PPMS2 Map 24 ()", "PPMS2\\PPMS2 Map 25 ()", "PPMS2\\PPMS2 Map 26 ()", "PPMS2\\PPMS2 Map 27 ()", "PPMS2\\PPMS2 Map 28 ()", "PPMS2\\PPMS2 Map 29 ()", "PPMS2\\PPMS2 Map 67 ()", "PPMS2\\PPMS2 Map 68 ()", "PPMS2\\PPMS2 Map 69 ()", "PPMS2\\PPMS2 Map 89 ()", "PPMS2\\PPMS2 Map 90 ()", "PPMS2\\PPMS2 Map 91 ()", "PPMS2\\PPMS2 Map 92 ()", "PPMS2\\PPMS2 Map 93 ()", "PPMS2\\PPMS2 Neck Excit (uA)", "PPMS2\\PPMS2 Neck Htr Cur (mA)", "PPMS2\\PPMS2 Neck Htr Pwr (W)", "PPMS2\\PPMS2 Neck Therm (K)", "PPMS2\\PPMS2 NeckHeater(Ohm)", "PPMS2\\PPMS2 Plat Excit (uA)", "PPMS2\\PPMS2 Plat Therm (K)", "PPMS2\\PPMS2 Pressure ()", "PPMS2\\PPMS2 PSU Field (Oe)", "PPMS2\\PPMS2 Pump power (W)", "PPMS2\\PPMS2 Pump temp (C)", "PPMS2\\PPMS2 Redirected 55 ()", "PPMS2\\PPMS2 Redirected 56 ()", "PPMS2\\PPMS2 Redirected 57 ()", "PPMS2\\PPMS2 Redirected 58 ()", "PPMS2\\PPMS2 Redirected 59 ()", "PPMS2\\PPMS2 Redirected 61 ()", "PPMS2\\PPMS2 Regen htr flag", "PPMS2\\PPMS2 Sample Position (deg)", "PPMS2\\PPMS2 Seq Stat ()", "PPMS2\\PPMS2 Setpoint (K)", "PPMS2\\PPMS2 Signal 1 Vin (V)", "PPMS2\\PPMS2 Signal 2 Vin (V)", "PPMS2\\PPMS2 Spare Excit (uA)", "PPMS2\\PPMS2 Spare Therm (K)", "PPMS2\\PPMS2 Status (code)", "PPMS2\\PPMS2 Sw heater state", "PPMS2\\PPMS2 Sys Temp ()", "PPMS2\\PPMS2 System Pres (Torr)", "PPMS2\\PPMS2 System Status (code)", "PPMS2\\PPMS2 Tableless Map53 ()", "PPMS2\\PPMS2 Tableless Map54 ()", "PPMS2\\PPMS2 Temperature (K)", "PPMS2\\PPMS2 Therm v", "PPMS2\\PPMS2 Time Stamp (sec)", "PPMS2\\PPMS2 Valve Position (deg)", "PPMSDR\\PPMSDR Annulus Pres (Torr)", "PPMSDR\\PPMSDR Annulus Vacuum (V)", "PPMSDR\\PPMSDR Block Htr Cur (mA)", "PPMSDR\\PPMSDR Block Htr Pwr (W)", "PPMSDR\\PPMSDR BlockHeater(Ohm)", "PPMSDR\\PPMSDR Bridge 1 Excitation (uA)", "PPMSDR\\PPMSDR Bridge 1 Resistance (ohms)", "PPMSDR\\PPMSDR Bridge 2 Excitation (uA)", "PPMSDR\\PPMSDR Bridge 2 Resistance (ohms)", "PPMSDR\\PPMSDR Bridge 3 Excitation (uA)", "PPMSDR\\PPMSDR Bridge 3 Resistance (ohms)", "PPMSDR\\PPMSDR Bridge 4 Excitation (uA)", "PPMSDR\\PPMSDR Bridge 4 Resistance (ohms)", "PPMSDR\\PPMSDR CIG Cernox (K)", "PPMSDR\\PPMSDR CIG Excit (uA)", "PPMSDR\\PPMSDR Comment", "PPMSDR\\PPMSDR DAC  I  (cnts)", "PPMSDR\\PPMSDR Digital Inputs (code)", "PPMSDR\\PPMSDR Drive 1 Iout (mA)", "PPMSDR\\PPMSDR Drive 1 Ipower (watts)", "PPMSDR\\PPMSDR Drive 2 Iout (mA)", "PPMSDR\\PPMSDR Drive 2 Ipower (watts)", "PPMSDR\\PPMSDR EXT Flow (L min)", "PPMSDR\\PPMSDR Flapper state", "PPMSDR\\PPMSDR Flow Rate (l min)", "PPMSDR\\PPMSDR He Level ()", "PPMSDR\\PPMSDR Hi res (A) read", "PPMSDR\\PPMSDR High Vacuum mode", "PPMSDR\\PPMSDR Hires enable", "PPMSDR\\PPMSDR Impedance (mode)", "PPMSDR\\PPMSDR iso flag", "PPMSDR\\PPMSDR KRPMs", "PPMSDR\\PPMSDR Last 2 eng st", "PPMSDR\\PPMSDR Log", "PPMSDR\\PPMSDR low res (A) read", "PPMSDR\\PPMSDR Mag (V) read", "PPMSDR\\PPMSDR Mag (V) set", "PPMSDR\\PPMSDR Mag adj sc(I)set", "PPMSDR\\PPMSDR Magnet (Oe)", "PPMSDR\\PPMSDR Magnetic Field (Oe)", "PPMSDR\\PPMSDR MAP 1", "PPMSDR\\PPMSDR MAP 10", "PPMSDR\\PPMSDR MAP 11", "PPMSDR\\PPMSDR MAP 12", "PPMSDR\\PPMSDR MAP 13", "PPMSDR\\PPMSDR MAP 14", "PPMSDR\\PPMSDR MAP 15", "PPMSDR\\PPMSDR MAP 16", "PPMSDR\\PPMSDR MAP 17", "PPMSDR\\PPMSDR MAP 18", "PPMSDR\\PPMSDR MAP 19", "PPMSDR\\PPMSDR MAP 2", "PPMSDR\\PPMSDR MAP 20", "PPMSDR\\PPMSDR Map 20 ()", "PPMSDR\\PPMSDR MAP 21", "PPMSDR\\PPMSDR Map 21 ()", "PPMSDR\\PPMSDR MAP 22", "PPMSDR\\PPMSDR Map 22 ()", "PPMSDR\\PPMSDR MAP 23", "PPMSDR\\PPMSDR Map 23 ()", "PPMSDR\\PPMSDR MAP 24", "PPMSDR\\PPMSDR Map 24 ()", "PPMSDR\\PPMSDR MAP 25", "PPMSDR\\PPMSDR Map 25 ()", "PPMSDR\\PPMSDR MAP 26", "PPMSDR\\PPMSDR Map 26 ()", "PPMSDR\\PPMSDR MAP 27", "PPMSDR\\PPMSDR Map 27 ()", "PPMSDR\\PPMSDR MAP 28", "PPMSDR\\PPMSDR Map 28 ()", "PPMSDR\\PPMSDR MAP 29", "PPMSDR\\PPMSDR Map 29 ()", "PPMSDR\\PPMSDR MAP 3", "PPMSDR\\PPMSDR MAP 30", "PPMSDR\\PPMSDR MAP 4", "PPMSDR\\PPMSDR MAP 5", "PPMSDR\\PPMSDR MAP 6", "PPMSDR\\PPMSDR Map 67 ()", "PPMSDR\\PPMSDR Map 68 ()", "PPMSDR\\PPMSDR Map 69 ()", "PPMSDR\\PPMSDR MAP 7", "PPMSDR\\PPMSDR MAP 8", "PPMSDR\\PPMSDR Map 89 ()", "PPMSDR\\PPMSDR MAP 9", "PPMSDR\\PPMSDR Map 90 ()", "PPMSDR\\PPMSDR Map 91 ()", "PPMSDR\\PPMSDR Map 92 ()", "PPMSDR\\PPMSDR Map 93 ()", "PPMSDR\\PPMSDR Neck Excit (uA)", "PPMSDR\\PPMSDR Neck Htr Cur (mA)", "PPMSDR\\PPMSDR Neck Htr Pwr (W)", "PPMSDR\\PPMSDR Neck Therm (K)", "PPMSDR\\PPMSDR NeckHeater(Ohm)", "PPMSDR\\PPMSDR Plat Excit (uA)", "PPMSDR\\PPMSDR Plat Therm (K)", "PPMSDR\\PPMSDR Pressure ()", "PPMSDR\\PPMSDR Pump power (W)", "PPMSDR\\PPMSDR Pump temp (C)", "PPMSDR\\PPMSDR Redirected 55 ()", "PPMSDR\\PPMSDR Redirected 56 ()", "PPMSDR\\PPMSDR Redirected 57 ()", "PPMSDR\\PPMSDR Redirected 58 ()", "PPMSDR\\PPMSDR Redirected 59 ()", "PPMSDR\\PPMSDR Redirected 61 ()", "PPMSDR\\PPMSDR Regen htr flag", "PPMSDR\\PPMSDR Sample Position (deg)", "PPMSDR\\PPMSDR Seq Stat ()", "PPMSDR\\PPMSDR Setpoint (K)", "PPMSDR\\PPMSDR Signal 1 Vin (V)", "PPMSDR\\PPMSDR Signal 2 Vin (V)", "PPMSDR\\PPMSDR Spare Excit (uA)", "PPMSDR\\PPMSDR Spare Therm (K)", "PPMSDR\\PPMSDR Status (code)", "PPMSDR\\PPMSDR Sw heater state", "PPMSDR\\PPMSDR Sys Temp ()", "PPMSDR\\PPMSDR System Pres (Torr)", "PPMSDR\\PPMSDR System Status (code)", "PPMSDR\\PPMSDR Tableless Map53 ()", "PPMSDR\\PPMSDR Tableless Map54 ()", "PPMSDR\\PPMSDR Temperature (K)", "PPMSDR\\PPMSDR Therm v", "PPMSDR\\PPMSDR Time Stamp (sec)", "PPMSDR\\PPMSDR Valve Position (deg)", "Sample Characterization\\2G Conductance", "Sample Characterization\\4G", "Sample Characterization\\4R", "Sample Characterization\\CURRENT", "Sample Characterization\\Experiment ID", "Sample Characterization\\Notes", "Sample Characterization\\OSCILLATION VOLTAGE", "Sample Characterization\\Sample Name", "Sample Characterization\\V1", "Sample Characterization\\V2", "SPM\\Laser Power", "SPM\\SPM scanner X", "SPM\\SPM scanner Y", "TEMPerHUM\\MFP : Humidity", "TEMPerHUM\\MFP : ID", "TEMPerHUM\\MFP : Location", "TEMPerHUM\\MFP : Picture URL", "TEMPerHUM\\MFP : Temperature", "TEMPerHUM\\MFP-3D : Humidity", "TEMPerHUM\\MFP-3D : ID", "TEMPerHUM\\MFP-3D : Location", "TEMPerHUM\\MFP-3D : Picture URL", "TEMPerHUM\\MFP-3D : Temperature", "TEMPerHUM\\TEST3 : Humidity", "TEMPerHUM\\TEST3 : ID", "TEMPerHUM\\TEST3 : Location", "TEMPerHUM\\TEST3 : Picture URL", "TEMPerHUM\\TEST3 : Temperature"]
  in  "Export Button":bool
  in  "path":path=path "C:/Users/Voodoo/Desktop/export"
  out "Shift Hours":dbl=-5.0 format="%#_13g"
  in  "Igor":bool=TRUE caption="Blank Button"
  in  "Favorite A (Right)":u16[](array[ring])=[136] items=["Attocube 3DR\\axis 1: Amplitude", "Attocube 3DR\\axis 1: Capacitance", "Attocube 3DR\\axis 1: control mode", "Attocube 3DR\\axis 1: current position", "Attocube 3DR\\axis 1: DCLevel", "Attocube 3DR\\axis 1: Frequency", "Attocube 3DR\\axis 1: moving", "Attocube 3DR\\axis 1: Output", "Attocube 3DR\\axis 1: rot. count", "Attocube 3DR\\axis 1: sensor disconnected", "Attocube 3DR\\axis 1: sensor error", "Attocube 3DR\\axis 1: Single Circle Mode", "Attocube 3DR\\axis 1: sp position", "Attocube 3DR\\axis 1: sp rot count", "Attocube 3DR\\axis 1: speed", "Attocube 3DR\\axis 1: StepWidth", "Attocube 3DR\\axis 1: stop detected", "Attocube 3DR\\axis 1: stop enable", "Attocube 3DR\\axis 1: Target GND", "Attocube 3DR\\axis 2: Amplitude", "Attocube 3DR\\axis 2: Capacitance", "Attocube 3DR\\axis 2: control mode", "Attocube 3DR\\axis 2: current position", "Attocube 3DR\\axis 2: DCLevel", "Attocube 3DR\\axis 2: Frequency", "Attocube 3DR\\axis 2: moving", "Attocube 3DR\\axis 2: Output", "Attocube 3DR\\axis 2: rot. count", "Attocube 3DR\\axis 2: sensor disconnected", "Attocube 3DR\\axis 2: sensor error", "Attocube 3DR\\axis 2: Single Circle Mode", "Attocube 3DR\\axis 2: sp position", "Attocube 3DR\\axis 2: sp rot count", "Attocube 3DR\\axis 2: speed", "Attocube 3DR\\axis 2: StepWidth", "Attocube 3DR\\axis 2: stop detected", "Attocube 3DR\\axis 2: stop enable", "Attocube 3DR\\axis 2: Target GND", "Attocube 3DR\\static amplitude", "Cypher\\Cypher RH1", "Cypher\\Cypher RH2", "Cypher\\Cypher Temperature", "Cypher\\Cypher_Funnel_Property", "Cypher\\Cypher_Path_Property", "Cypher\\Cypher_Rectangle_Property", "DR200\\DR200_Magnet_Field", "DR200\\DR200_Magnet_Field_Target", "DR200\\DR200_Magnet_PS_Current", "DR200\\DR200_Magnet_PS_Field", "DR200\\DR200_Magnet_PS_Voltage", "DR200\\DR200_Magnet_Rate_Target", "DR200\\DR200_Magnet_Status_Activity", "DR200\\DR200_Magnet_Status_Mode", "DR200\\DR200_Magnet_Status_Switch_Heater", "DR200\\DR200_Magnet_Status_System", "JLevy\\Levy 1", "Leiden CF900\\CF Impedance CMN", "Leiden CF900\\CF_FP_STATE", "Leiden CF900\\CF_KH_ch1", "Leiden CF900\\CF_KH_ch2", "Leiden CF900\\CF_KH_ch3", "Leiden CF900\\CF_KH_ch4", "Leiden CF900\\CF_KH_ch5", "Leiden CF900\\CF_KH_ch6", "Leiden CF900\\CF_KH_ch7", "Leiden CF900\\CF_KH_ch8", "Leiden CF900\\CF_TC_calibration", "Leiden CF900\\CF_TC_description", "Leiden CF900\\CF_TC_Z_calibration", "Leiden CF900\\CF_TC_Z_description", "Leiden CF900\\CF_TC_Z_R0", "Leiden CF900\\CF_TC_Z_R1", "Leiden CF900\\CF_TC_Z_R2", "Leiden CF900\\CF_TC_Z_R3", "Leiden CF900\\CF_TC_Z_R4", "Leiden CF900\\CF_TC_Z_R5", "Leiden CF900\\CF_TC_Z_R6", "Leiden CF900\\CF_TC_Z_R7", "Leiden CF900\\CF_TC_Z_R8", "Leiden CF900\\CF_TC_Z_R9", "Leiden CF900\\CF_TC_Z_T0", "Leiden CF900\\CF_TC_Z_T1", "Leiden CF900\\CF_TC_Z_T2", "Leiden CF900\\CF_TC_Z_T3", "Leiden CF900\\CF_TC_Z_T4", "Leiden CF900\\CF_TC_Z_T5", "Leiden CF900\\CF_TC_Z_T6", "Leiden CF900\\CF_TC_Z_T7", "Leiden CF900\\CF_TC_Z_T8", "Leiden CF900\\CF_TC_Z_T9", "Leiden CF900\\CF900_Cstill", "Leiden CF900\\Leiden CF FP\\CF FP Flow", "Leiden CF900\\Leiden CF FP\\CF FP He", "Leiden CF900\\Leiden CF FP\\CF FP MG0", "Leiden CF900\\Leiden CF FP\\CF FP MG1", "Leiden CF900\\Leiden CF FP\\CF FP MG2", "Leiden CF900\\Leiden CF FP\\CF FP MG3", "Leiden CF900\\Leiden CF FP\\CF FP MG4", "Leiden CF900\\Leiden CF FP\\CF FP MG5", "Leiden CF900\\Leiden CF FP\\CF FP oil", "Leiden CF900\\Leiden CF FP\\CF FP P_high", "Leiden CF900\\Leiden CF FP\\CF FP P_low", "Leiden CF900\\Leiden CF FP\\CF FP P1", "Leiden CF900\\Leiden CF FP\\CF FP P2", "Leiden CF900\\Leiden CF FP\\CF FP P3", "Leiden CF900\\Leiden CF FP\\CF FP P4", "Leiden CF900\\Leiden CF FP\\CF FP P5", "Leiden CF900\\Leiden CF FP\\CF FP P6", "Leiden CF900\\Leiden CF FP\\CF FP P7", "Leiden CF900\\Leiden CF FP\\CF FP PT current", "Leiden CF900\\Leiden CF FP\\CF FP PT on", "Leiden CF900\\Leiden CF FP\\CF FP State0", "Leiden CF900\\Leiden CF FP\\CF FP State1", "Leiden CF900\\Leiden CF FP\\CF FP State2", "Leiden CF900\\Leiden CF FP\\CF FP W_in", "Leiden CF900\\Leiden CF FP\\CF FP W_out", "Leiden CF900\\Leiden CF Impedance Bridge\\CF IB TA", "Leiden CF900\\Leiden CF Impedance Bridge\\CF IB TB", "Leiden CF900\\Leiden CF Impedance Bridge\\CF IB TC", "Leiden CF900\\Leiden CF Impedance Bridge\\CF IB TD", "Leiden CF900\\Leiden CF Impedance Bridge\\CF IB TE", "Leiden CF900\\Leiden CF Magnetic Field\\CF Field X", "Leiden CF900\\Leiden CF Magnetic Field\\CF Field Y", "Leiden CF900\\Leiden CF Magnetic Field\\CF Field Z", "Leiden CF900\\Leiden CF TC\\CF TC I0", "Leiden CF900\\Leiden CF TC\\CF TC I1", "Leiden CF900\\Leiden CF TC\\CF TC I2", "Leiden CF900\\Leiden CF TC\\CF TC I3", "Leiden CF900\\Leiden CF TC\\CF TC R0", "Leiden CF900\\Leiden CF TC\\CF TC R1", "Leiden CF900\\Leiden CF TC\\CF TC R2", "Leiden CF900\\Leiden CF TC\\CF TC R3", "Leiden CF900\\Leiden CF TC\\CF TC R4", "Leiden CF900\\Leiden CF TC\\CF TC R5", "Leiden CF900\\Leiden CF TC\\CF TC R6", "Leiden CF900\\Leiden CF TC\\CF TC R7", "Leiden CF900\\Leiden CF TC\\CF TC T0", "Leiden CF900\\Leiden CF TC\\CF TC T1", "Leiden CF900\\Leiden CF TC\\CF TC T2", "Leiden CF900\\Leiden CF TC\\CF TC T3", "Leiden CF900\\Leiden CF TC\\CF TC T4", "Leiden CF900\\Leiden CF TC\\CF TC T5", "Leiden CF900\\Leiden CF TC\\CF TC T6", "Leiden CF900\\Leiden CF TC\\CF TC T7", "Leiden CF900\\RuO2_T", "Leiden CF900\\RuO2_Z", "Leiden CF900\\Vbg", "Leiden CF900\\VRM VrmSweepMode", "Leiden CF900\\VRM VrmSweepRate", "Leiden CF900\\VRM VrmSweepTime", "Leiden CF900\\VRM VrmX setpT", "Leiden CF900\\VRM VrmY setpT", "Leiden CF900\\VRM VrmZ setpT", "Leiden CF900\\VRM X at rest", "Leiden CF900\\VRM X magA", "Leiden CF900\\VRM X magT", "Leiden CF900\\VRM X meas A", "Leiden CF900\\VRM X meas V", "Leiden CF900\\VRM X outA", "Leiden CF900\\VRM X outT", "Leiden CF900\\VRM X setpT", "Leiden CF900\\VRM X Status", "Leiden CF900\\VRM X sweep", "Leiden CF900\\VRM X sweep A", "Leiden CF900\\VRM Y at rest", "Leiden CF900\\VRM Y magA", "Leiden CF900\\VRM Y magT", "Leiden CF900\\VRM Y meas A", "Leiden CF900\\VRM Y meas V", "Leiden CF900\\VRM Y outA", "Leiden CF900\\VRM Y outT", "Leiden CF900\\VRM Y setpT", "Leiden CF900\\VRM Y Status", "Leiden CF900\\VRM Y sweep", "Leiden CF900\\VRM Y sweep A", "Leiden CF900\\VRM Z at rest", "Leiden CF900\\VRM Z magA", "Leiden CF900\\VRM Z magT", "Leiden CF900\\VRM Z meas A", "Leiden CF900\\VRM Z meas V", "Leiden CF900\\VRM Z outA", "Leiden CF900\\VRM Z outT", "Leiden CF900\\VRM Z setpT", "Leiden CF900\\VRM Z Status", "Leiden CF900\\VRM Z sweep", "Leiden CF900\\VRM Z sweep A", "MFP3D\\MFP3D Hum", "MFP3D\\MFP3D Temperature", "MFP3D\\MFP3D TSP01 Hum", "MFP3D\\MFP3D TSP01 Temperature", "MFP3D\\MFP3D User", "MNK_18T\\1820_IPS_Current", "MNK_18T\\1820_IPS_Level_He", "MNK_18T\\1820_IPS_Level_N2", "MNK_18T\\1820_IPS_M1_Current", "MNK_18T\\1820_IPS_M1_Voltage", "MNK_18T\\1820_IPS_M2_Current", "MNK_18T\\1820_IPS_M2_Voltage", "MNK_18T\\1820_IPS_M3_Current", "MNK_18T\\1820_IPS_M3_Voltage", "MNK_18T\\1820_IPS_Magnet_Field", "MNK_18T\\1820_IPS_Magnet_Temperature", "MNK_18T\\1820_IPS_Magnet_Temperature_R", "MNK_18T\\1820_IPS_PS_Field", "MNK_18T\\1820_IPS_Reply", "MNK_18T\\1820_IPS_Status", "MNK_18T\\1820_IPS_Switch", "MNK_18T\\1820_IPS_Target_Field", "MNK_18T\\1820_IPS_Target_Field_Rate", "MNK_18T\\1820_IPS_Voltage", "MNK_18T\\1820_ITC_Lambda_Status", "MNK_18T\\1820_ITC_Lambda_Temperature", "MNK_18T\\1820_ITC_Lambda_Temperature_R", "MNK_18T\\1820_ITC_Needle_Valve", "MNK_18T\\1820_ITC_Pressure", "MNK_18T\\1820_ITC_Reply", "MNK_18T\\KH_ch1", "MNK_18T\\KH_ch2", "MNK_18T\\KH_ch3", "MNK_18T\\KH_ch4", "MNK_18T\\KH_ch5", "MNK_18T\\KH_ch6", "MNK_18T\\KH_ch7", "MNK_18T\\KH_ch8", "MNK_18T\\Lockin_Results", "MNK_18T\\MNK_CMN-187_T", "MNK_18T\\MNK_CMN-187_Z", "MNK_18T\\MNK_Cstill_T", "MNK_18T\\MNK_Cstill_Z", "MNK_18T\\MNK_FP_Flow", "MNK_18T\\MNK_FP_MG0", "MNK_18T\\MNK_FP_MG1", "MNK_18T\\MNK_FP_MG2", "MNK_18T\\MNK_FP_MG3", "MNK_18T\\MNK_FP_MG4", "MNK_18T\\MNK_FP_MG5", "MNK_18T\\MNK_FP_P1", "MNK_18T\\MNK_FP_P2", "MNK_18T\\MNK_FP_P3", "MNK_18T\\MNK_FP_P4", "MNK_18T\\MNK_FP_P5", "MNK_18T\\MNK_FP_P6", "MNK_18T\\MNK_FP_P7", "MNK_18T\\MNK_FP_STATE", "MNK_18T\\MNK_FP_State0", "MNK_18T\\MNK_FP_State1", "MNK_18T\\MNK_FP_State2", "MNK_18T\\MNK_TC_calibration", "MNK_18T\\MNK_TC_description", "MNK_18T\\MNK_TC_I0", "MNK_18T\\MNK_TC_I1", "MNK_18T\\MNK_TC_I2", "MNK_18T\\MNK_TC_I3", "MNK_18T\\MNK_TC_R0", "MNK_18T\\MNK_TC_R1", "MNK_18T\\MNK_TC_R2", "MNK_18T\\MNK_TC_R3", "MNK_18T\\MNK_TC_R4", "MNK_18T\\MNK_TC_R5", "MNK_18T\\MNK_TC_R6", "MNK_18T\\MNK_TC_R7", "MNK_18T\\MNK_TC_T0", "MNK_18T\\MNK_TC_T1", "MNK_18T\\MNK_TC_T2", "MNK_18T\\MNK_TC_T3", "MNK_18T\\MNK_TC_T4", "MNK_18T\\MNK_TC_T5", "MNK_18T\\MNK_TC_T6", "MNK_18T\\MNK_TC_T7", "MNK_18T\\MNK_TC_Z_calibration", "MNK_18T\\MNK_TC_Z_description", "MNK_18T\\OSC_config", "MNK_18T\\Vbg", "Montana THZ 1\\THZ 1 Dew Point", "Montana THZ 1\\THZ 1 Humidity", "Montana THZ 1\\THZ 1 Temperature", "OneNote API HTTP\\Access Token 0000000048124379", "OneNote API HTTP\\Asana Access Token 15669051163913", "PPMS 1\\PPMS 1 Magnetic Field", "PPMS 1\\PPMS 1 Temperature", "PPMS 2\\PPMS 2 Flow Rate", "PPMS 2\\PPMS 2 Helium Level", "PPMS 2\\PPMS 2 Magnetic Field", "PPMS 2\\PPMS 2 Position", "PPMS 2\\PPMS 2 Sys Pressure", "PPMS 2\\PPMS 2 Temperature", "PPMS 2\\PPMS 2 Vbg", "PPMS2\\PPMS2 Annulus Pres (Torr)", "PPMS2\\PPMS2 Annulus Vacuum (V)", "PPMS2\\PPMS2 Block Htr Cur (mA)", "PPMS2\\PPMS2 Block Htr Pwr (W)", "PPMS2\\PPMS2 BlockHeater(Ohm)", "PPMS2\\PPMS2 Bridge 1 Excitation (uA)", "PPMS2\\PPMS2 Bridge 1 Resistance (ohms)", "PPMS2\\PPMS2 Bridge 2 Excitation (uA)", "PPMS2\\PPMS2 Bridge 2 Resistance (ohms)", "PPMS2\\PPMS2 Bridge 3 Excitation (uA)", "PPMS2\\PPMS2 Bridge 3 Resistance (ohms)", "PPMS2\\PPMS2 Bridge 4 Excitation (uA)", "PPMS2\\PPMS2 Bridge 4 Resistance (ohms)", "PPMS2\\PPMS2 CIG Cernox (K)", "PPMS2\\PPMS2 CIG Excit (uA)", "PPMS2\\PPMS2 Comment", "PPMS2\\PPMS2 DAC  I  (cnts)", "PPMS2\\PPMS2 Digital Inputs (code)", "PPMS2\\PPMS2 Drive 1 Iout (mA)", "PPMS2\\PPMS2 Drive 1 Ipower (watts)", "PPMS2\\PPMS2 Drive 2 Iout (mA)", "PPMS2\\PPMS2 Drive 2 Ipower (watts)", "PPMS2\\PPMS2 EXT Flow (L min)", "PPMS2\\PPMS2 Flapper state", "PPMS2\\PPMS2 Flow Rate (l min)", "PPMS2\\PPMS2 He Level ()", "PPMS2\\PPMS2 Hi res (A) read", "PPMS2\\PPMS2 High Vacuum mode", "PPMS2\\PPMS2 Hires enable", "PPMS2\\PPMS2 Impedance (mode)", "PPMS2\\PPMS2 iso flag", "PPMS2\\PPMS2 KRPMs", "PPMS2\\PPMS2 Last 2 eng st", "PPMS2\\PPMS2 Log", "PPMS2\\PPMS2 Mag (V) read", "PPMS2\\PPMS2 Mag (V) set", "PPMS2\\PPMS2 Mag adj sc(I)set", "PPMS2\\PPMS2 Magnet (Oe)", "PPMS2\\PPMS2 Magnetic Field (Oe)", "PPMS2\\PPMS2 Map 20 ()", "PPMS2\\PPMS2 Map 21 ()", "PPMS2\\PPMS2 Map 22 ()", "PPMS2\\PPMS2 Map 23 ()", "PPMS2\\PPMS2 Map 24 ()", "PPMS2\\PPMS2 Map 25 ()", "PPMS2\\PPMS2 Map 26 ()", "PPMS2\\PPMS2 Map 27 ()", "PPMS2\\PPMS2 Map 28 ()", "PPMS2\\PPMS2 Map 29 ()", "PPMS2\\PPMS2 Map 67 ()", "PPMS2\\PPMS2 Map 68 ()", "PPMS2\\PPMS2 Map 69 ()", "PPMS2\\PPMS2 Map 89 ()", "PPMS2\\PPMS2 Map 90 ()", "PPMS2\\PPMS2 Map 91 ()", "PPMS2\\PPMS2 Map 92 ()", "PPMS2\\PPMS2 Map 93 ()", "PPMS2\\PPMS2 Neck Excit (uA)", "PPMS2\\PPMS2 Neck Htr Cur (mA)", "PPMS2\\PPMS2 Neck Htr Pwr (W)", "PPMS2\\PPMS2 Neck Therm (K)", "PPMS2\\PPMS2 NeckHeater(Ohm)", "PPMS2\\PPMS2 Plat Excit (uA)", "PPMS2\\PPMS2 Plat Therm (K)", "PPMS2\\PPMS2 Pressure ()", "PPMS2\\PPMS2 PSU Field (Oe)", "PPMS2\\PPMS2 Pump power (W)", "PPMS2\\PPMS2 Pump temp (C)", "PPMS2\\PPMS2 Redirected 55 ()", "PPMS2\\PPMS2 Redirected 56 ()", "PPMS2\\PPMS2 Redirected 57 ()", "PPMS2\\PPMS2 Redirected 58 ()", "PPMS2\\PPMS2 Redirected 59 ()", "PPMS2\\PPMS2 Redirected 61 ()", "PPMS2\\PPMS2 Regen htr flag", "PPMS2\\PPMS2 Sample Position (deg)", "PPMS2\\PPMS2 Seq Stat ()", "PPMS2\\PPMS2 Setpoint (K)", "PPMS2\\PPMS2 Signal 1 Vin (V)", "PPMS2\\PPMS2 Signal 2 Vin (V)", "PPMS2\\PPMS2 Spare Excit (uA)", "PPMS2\\PPMS2 Spare Therm (K)", "PPMS2\\PPMS2 Status (code)", "PPMS2\\PPMS2 Sw heater state", "PPMS2\\PPMS2 Sys Temp ()", "PPMS2\\PPMS2 System Pres (Torr)", "PPMS2\\PPMS2 System Status (code)", "PPMS2\\PPMS2 Tableless Map53 ()", "PPMS2\\PPMS2 Tableless Map54 ()", "PPMS2\\PPMS2 Temperature (K)", "PPMS2\\PPMS2 Therm v", "PPMS2\\PPMS2 Time Stamp (sec)", "PPMS2\\PPMS2 Valve Position (deg)", "PPMSDR\\PPMSDR Annulus Pres (Torr)", "PPMSDR\\PPMSDR Annulus Vacuum (V)", "PPMSDR\\PPMSDR Block Htr Cur (mA)", "PPMSDR\\PPMSDR Block Htr Pwr (W)", "PPMSDR\\PPMSDR BlockHeater(Ohm)", "PPMSDR\\PPMSDR Bridge 1 Excitation (uA)", "PPMSDR\\PPMSDR Bridge 1 Resistance (ohms)", "PPMSDR\\PPMSDR Bridge 2 Excitation (uA)", "PPMSDR\\PPMSDR Bridge 2 Resistance (ohms)", "PPMSDR\\PPMSDR Bridge 3 Excitation (uA)", "PPMSDR\\PPMSDR Bridge 3 Resistance (ohms)", "PPMSDR\\PPMSDR Bridge 4 Excitation (uA)", "PPMSDR\\PPMSDR Bridge 4 Resistance (ohms)", "PPMSDR\\PPMSDR CIG Cernox (K)", "PPMSDR\\PPMSDR CIG Excit (uA)", "PPMSDR\\PPMSDR Comment", "PPMSDR\\PPMSDR DAC  I  (cnts)", "PPMSDR\\PPMSDR Digital Inputs (code)", "PPMSDR\\PPMSDR Drive 1 Iout (mA)", "PPMSDR\\PPMSDR Drive 1 Ipower (watts)", "PPMSDR\\PPMSDR Drive 2 Iout (mA)", "PPMSDR\\PPMSDR Drive 2 Ipower (watts)", "PPMSDR\\PPMSDR EXT Flow (L min)", "PPMSDR\\PPMSDR Flapper state", "PPMSDR\\PPMSDR Flow Rate (l min)", "PPMSDR\\PPMSDR He Level ()", "PPMSDR\\PPMSDR Hi res (A) read", "PPMSDR\\PPMSDR High Vacuum mode", "PPMSDR\\PPMSDR Hires enable", "PPMSDR\\PPMSDR Impedance (mode)", "PPMSDR\\PPMSDR iso flag", "PPMSDR\\PPMSDR KRPMs", "PPMSDR\\PPMSDR Last 2 eng st", "PPMSDR\\PPMSDR Log", "PPMSDR\\PPMSDR low res (A) read", "PPMSDR\\PPMSDR Mag (V) read", "PPMSDR\\PPMSDR Mag (V) set", "PPMSDR\\PPMSDR Mag adj sc(I)set", "PPMSDR\\PPMSDR Magnet (Oe)", "PPMSDR\\PPMSDR Magnetic Field (Oe)", "PPMSDR\\PPMSDR MAP 1", "PPMSDR\\PPMSDR MAP 10", "PPMSDR\\PPMSDR MAP 11", "PPMSDR\\PPMSDR MAP 12", "PPMSDR\\PPMSDR MAP 13", "PPMSDR\\PPMSDR MAP 14", "PPMSDR\\PPMSDR MAP 15", "PPMSDR\\PPMSDR MAP 16", "PPMSDR\\PPMSDR MAP 17", "PPMSDR\\PPMSDR MAP 18", "PPMSDR\\PPMSDR MAP 19", "PPMSDR\\PPMSDR MAP 2", "PPMSDR\\PPMSDR MAP 20", "PPMSDR\\PPMSDR Map 20 ()", "PPMSDR\\PPMSDR MAP 21", "PPMSDR\\PPMSDR Map 21 ()", "PPMSDR\\PPMSDR MAP 22", "PPMSDR\\PPMSDR Map 22 ()", "PPMSDR\\PPMSDR MAP 23", "PPMSDR\\PPMSDR Map 23 ()", "PPMSDR\\PPMSDR MAP 24", "PPMSDR\\PPMSDR Map 24 ()", "PPMSDR\\PPMSDR MAP 25", "PPMSDR\\PPMSDR Map 25 ()", "PPMSDR\\PPMSDR MAP 26", "PPMSDR\\PPMSDR Map 26 ()", "PPMSDR\\PPMSDR MAP 27", "PPMSDR\\PPMSDR Map 27 ()", "PPMSDR\\PPMSDR MAP 28", "PPMSDR\\PPMSDR Map 28 ()", "PPMSDR\\PPMSDR MAP 29", "PPMSDR\\PPMSDR Map 29 ()", "PPMSDR\\PPMSDR MAP 3", "PPMSDR\\PPMSDR MAP 30", "PPMSDR\\PPMSDR MAP 4", "PPMSDR\\PPMSDR MAP 5", "PPMSDR\\PPMSDR MAP 6", "PPMSDR\\PPMSDR Map 67 ()", "PPMSDR\\PPMSDR Map 68 ()", "PPMSDR\\PPMSDR Map 69 ()", "PPMSDR\\PPMSDR MAP 7", "PPMSDR\\PPMSDR MAP 8", "PPMSDR\\PPMSDR Map 89 ()", "PPMSDR\\PPMSDR MAP 9", "PPMSDR\\PPMSDR Map 90 ()", "PPMSDR\\PPMSDR Map 91 ()", "PPMSDR\\PPMSDR Map 92 ()", "PPMSDR\\PPMSDR Map 93 ()", "PPMSDR\\PPMSDR Neck Excit (uA)", "PPMSDR\\PPMSDR Neck Htr Cur (mA)", "PPMSDR\\PPMSDR Neck Htr Pwr (W)", "PPMSDR\\PPMSDR Neck Therm (K)", "PPMSDR\\PPMSDR NeckHeater(Ohm)", "PPMSDR\\PPMSDR Plat Excit (uA)", "PPMSDR\\PPMSDR Plat Therm (K)", "PPMSDR\\PPMSDR Pressure ()", "PPMSDR\\PPMSDR Pump power (W)", "PPMSDR\\PPMSDR Pump temp (C)", "PPMSDR\\PPMSDR Redirected 55 ()", "PPMSDR\\PPMSDR Redirected 56 ()", "PPMSDR\\PPMSDR Redirected 57 ()", "PPMSDR\\PPMSDR Redirected 58 ()", "PPMSDR\\PPMSDR Redirected 59 ()", "PPMSDR\\PPMSDR Redirected 61 ()", "PPMSDR\\PPMSDR Regen htr flag", "PPMSDR\\PPMSDR Sample Position (deg)", "PPMSDR\\PPMSDR Seq Stat ()", "PPMSDR\\PPMSDR Setpoint (K)", "PPMSDR\\PPMSDR Signal 1 Vin (V)", "PPMSDR\\PPMSDR Signal 2 Vin (V)", "PPMSDR\\PPMSDR Spare Excit (uA)", "PPMSDR\\PPMSDR Spare Therm (K)", "PPMSDR\\PPMSDR Status (code)", "PPMSDR\\PPMSDR Sw heater state", "PPMSDR\\PPMSDR Sys Temp ()", "PPMSDR\\PPMSDR System Pres (Torr)", "PPMSDR\\PPMSDR System Status (code)", "PPMSDR\\PPMSDR Tableless Map53 ()", "PPMSDR\\PPMSDR Tableless Map54 ()", "PPMSDR\\PPMSDR Temperature (K)", "PPMSDR\\PPMSDR Therm v", "PPMSDR\\PPMSDR Time Stamp (sec)", "PPMSDR\\PPMSDR Valve Position (deg)", "Sample Characterization\\2G Conductance", "Sample Characterization\\4G", "Sample Characterization\\4R", "Sample Characterization\\CURRENT", "Sample Characterization\\Experiment ID", "Sample Characterization\\Notes", "Sample Characterization\\OSCILLATION VOLTAGE", "Sample Characterization\\Sample Name", "Sample Characterization\\V1", "Sample Characterization\\V2", "SPM\\Laser Power", "SPM\\SPM scanner X", "SPM\\SPM scanner Y", "TEMPerHUM\\MFP : Humidity", "TEMPerHUM\\MFP : ID", "TEMPerHUM\\MFP : Location", "TEMPerHUM\\MFP : Picture URL", "TEMPerHUM\\MFP : Temperature", "TEMPerHUM\\MFP-3D : Humidity", "TEMPerHUM\\MFP-3D : ID", "TEMPerHUM\\MFP-3D : Location", "TEMPerHUM\\MFP-3D : Picture URL", "TEMPerHUM\\MFP-3D : Temperature", "TEMPerHUM\\TEST3 : Humidity", "TEMPerHUM\\TEST3 : ID", "TEMPerHUM\\TEST3 : Location", "TEMPerHUM\\TEST3 : Picture URL", "TEMPerHUM\\TEST3 : Temperature"]
  in  "Favorite A (Left)":u16[](array[ring])=[100] items=["Attocube 3DR\\axis 1: Amplitude", "Attocube 3DR\\axis 1: Capacitance", "Attocube 3DR\\axis 1: control mode", "Attocube 3DR\\axis 1: current position", "Attocube 3DR\\axis 1: DCLevel", "Attocube 3DR\\axis 1: Frequency", "Attocube 3DR\\axis 1: moving", "Attocube 3DR\\axis 1: Output", "Attocube 3DR\\axis 1: rot. count", "Attocube 3DR\\axis 1: sensor disconnected", "Attocube 3DR\\axis 1: sensor error", "Attocube 3DR\\axis 1: Single Circle Mode", "Attocube 3DR\\axis 1: sp position", "Attocube 3DR\\axis 1: sp rot count", "Attocube 3DR\\axis 1: speed", "Attocube 3DR\\axis 1: StepWidth", "Attocube 3DR\\axis 1: stop detected", "Attocube 3DR\\axis 1: stop enable", "Attocube 3DR\\axis 1: Target GND", "Attocube 3DR\\axis 2: Amplitude", "Attocube 3DR\\axis 2: Capacitance", "Attocube 3DR\\axis 2: control mode", "Attocube 3DR\\axis 2: current position", "Attocube 3DR\\axis 2: DCLevel", "Attocube 3DR\\axis 2: Frequency", "Attocube 3DR\\axis 2: moving", "Attocube 3DR\\axis 2: Output", "Attocube 3DR\\axis 2: rot. count", "Attocube 3DR\\axis 2: sensor disconnected", "Attocube 3DR\\axis 2: sensor error", "Attocube 3DR\\axis 2: Single Circle Mode", "Attocube 3DR\\axis 2: sp position", "Attocube 3DR\\axis 2: sp rot count", "Attocube 3DR\\axis 2: speed", "Attocube 3DR\\axis 2: StepWidth", "Attocube 3DR\\axis 2: stop detected", "Attocube 3DR\\axis 2: stop enable", "Attocube 3DR\\axis 2: Target GND", "Attocube 3DR\\static amplitude", "Cypher\\Cypher RH1", "Cypher\\Cypher RH2", "Cypher\\Cypher Temperature", "Cypher\\Cypher_Funnel_Property", "Cypher\\Cypher_Path_Property", "Cypher\\Cypher_Rectangle_Property", "DR200\\DR200_Magnet_Field", "DR200\\DR200_Magnet_Field_Target", "DR200\\DR200_Magnet_PS_Current", "DR200\\DR200_Magnet_PS_Field", "DR200\\DR200_Magnet_PS_Voltage", "DR200\\DR200_Magnet_Rate_Target", "DR200\\DR200_Magnet_Status_Activity", "DR200\\DR200_Magnet_Status_Mode", "DR200\\DR200_Magnet_Status_Switch_Heater", "DR200\\DR200_Magnet_Status_System", "JLevy\\Levy 1", "Leiden CF900\\CF Impedance CMN", "Leiden CF900\\CF_FP_STATE", "Leiden CF900\\CF_KH_ch1", "Leiden CF900\\CF_KH_ch2", "Leiden CF900\\CF_KH_ch3", "Leiden CF900\\CF_KH_ch4", "Leiden CF900\\CF_KH_ch5", "Leiden CF900\\CF_KH_ch6", "Leiden CF900\\CF_KH_ch7", "Leiden CF900\\CF_KH_ch8", "Leiden CF900\\CF_TC_calibration", "Leiden CF900\\CF_TC_description", "Leiden CF900\\CF_TC_Z_calibration", "Leiden CF900\\CF_TC_Z_description", "Leiden CF900\\CF_TC_Z_R0", "Leiden CF900\\CF_TC_Z_R1", "Leiden CF900\\CF_TC_Z_R2", "Leiden CF900\\CF_TC_Z_R3", "Leiden CF900\\CF_TC_Z_R4", "Leiden CF900\\CF_TC_Z_R5", "Leiden CF900\\CF_TC_Z_R6", "Leiden CF900\\CF_TC_Z_R7", "Leiden CF900\\CF_TC_Z_R8", "Leiden CF900\\CF_TC_Z_R9", "Leiden CF900\\CF_TC_Z_T0", "Leiden CF900\\CF_TC_Z_T1", "Leiden CF900\\CF_TC_Z_T2", "Leiden CF900\\CF_TC_Z_T3", "Leiden CF900\\CF_TC_Z_T4", "Leiden CF900\\CF_TC_Z_T5", "Leiden CF900\\CF_TC_Z_T6", "Leiden CF900\\CF_TC_Z_T7", "Leiden CF900\\CF_TC_Z_T8", "Leiden CF900\\CF_TC_Z_T9", "Leiden CF900\\CF900_Cstill", "Leiden CF900\\Leiden CF FP\\CF FP Flow", "Leiden CF900\\Leiden CF FP\\CF FP He", "Leiden CF900\\Leiden CF FP\\CF FP MG0", "Leiden CF900\\Leiden CF FP\\CF FP MG1", "Leiden CF900\\Leiden CF FP\\CF FP MG2", "Leiden CF900\\Leiden CF FP\\CF FP MG3", "Leiden CF900\\Leiden CF FP\\CF FP MG4", "Leiden CF900\\Leiden CF FP\\CF FP MG5", "Leiden CF900\\Leiden CF FP\\CF FP oil", "Leiden CF900\\Leiden CF FP\\CF FP P_high", "Leiden CF900\\Leiden CF FP\\CF FP P_low", "Leiden CF900\\Leiden CF FP\\CF FP P1", "Leiden CF900\\Leiden CF FP\\CF FP P2", "Leiden CF900\\Leiden CF FP\\CF FP P3", "Leiden CF900\\Leiden CF FP\\CF FP P4", "Leiden CF900\\Leiden CF FP\\CF FP P5", "Leiden CF900\\Leiden CF FP\\CF FP P6", "Leiden CF900\\Leiden CF FP\\CF FP P7", "Leiden CF900\\Leiden CF FP\\CF FP PT current", "Leiden CF900\\Leiden CF FP\\CF FP PT on", "Leiden CF900\\Leiden CF FP\\CF FP State0", "Leiden CF900\\Leiden CF FP\\CF FP State1", "Leiden CF900\\Leiden CF FP\\CF FP State2", "Leiden CF900\\Leiden CF FP\\CF FP W_in", "Leiden CF900\\Leiden CF FP\\CF FP W_out", "Leiden CF900\\Leiden CF Impedance Bridge\\CF IB TA", "Leiden CF900\\Leiden CF Impedance Bridge\\CF IB TB", "Leiden CF900\\Leiden CF Impedance Bridge\\CF IB TC", "Leiden CF900\\Leiden CF Impedance Bridge\\CF IB TD", "Leiden CF900\\Leiden CF Impedance Bridge\\CF IB TE", "Leiden CF900\\Leiden CF Magnetic Field\\CF Field X", "Leiden CF900\\Leiden CF Magnetic Field\\CF Field Y", "Leiden CF900\\Leiden CF Magnetic Field\\CF Field Z", "Leiden CF900\\Leiden CF TC\\CF TC I0", "Leiden CF900\\Leiden CF TC\\CF TC I1", "Leiden CF900\\Leiden CF TC\\CF TC I2", "Leiden CF900\\Leiden CF TC\\CF TC I3", "Leiden CF900\\Leiden CF TC\\CF TC R0", "Leiden CF900\\Leiden CF TC\\CF TC R1", "Leiden CF900\\Leiden CF TC\\CF TC R2", "Leiden CF900\\Leiden CF TC\\CF TC R3", "Leiden CF900\\Leiden CF TC\\CF TC R4", "Leiden CF900\\Leiden CF TC\\CF TC R5", "Leiden CF900\\Leiden CF TC\\CF TC R6", "Leiden CF900\\Leiden CF TC\\CF TC R7", "Leiden CF900\\Leiden CF TC\\CF TC T0", "Leiden CF900\\Leiden CF TC\\CF TC T1", "Leiden CF900\\Leiden CF TC\\CF TC T2", "Leiden CF900\\Leiden CF TC\\CF TC T3", "Leiden CF900\\Leiden CF TC\\CF TC T4", "Leiden CF900\\Leiden CF TC\\CF TC T5", "Leiden CF900\\Leiden CF TC\\CF TC T6", "Leiden CF900\\Leiden CF TC\\CF TC T7", "Leiden CF900\\RuO2_T", "Leiden CF900\\RuO2_Z", "Leiden CF900\\Vbg", "Leiden CF900\\VRM VrmSweepMode", "Leiden CF900\\VRM VrmSweepRate", "Leiden CF900\\VRM VrmSweepTime", "Leiden CF900\\VRM VrmX setpT", "Leiden CF900\\VRM VrmY setpT", "Leiden CF900\\VRM VrmZ setpT", "Leiden CF900\\VRM X at rest", "Leiden CF900\\VRM X magA", "Leiden CF900\\VRM X magT", "Leiden CF900\\VRM X meas A", "Leiden CF900\\VRM X meas V", "Leiden CF900\\VRM X outA", "Leiden CF900\\VRM X outT", "Leiden CF900\\VRM X setpT", "Leiden CF900\\VRM X Status", "Leiden CF900\\VRM X sweep", "Leiden CF900\\VRM X sweep A", "Leiden CF900\\VRM Y at rest", "Leiden CF900\\VRM Y magA", "Leiden CF900\\VRM Y magT", "Leiden CF900\\VRM Y meas A", "Leiden CF900\\VRM Y meas V", "Leiden CF900\\VRM Y outA", "Leiden CF900\\VRM Y outT", "Leiden CF900\\VRM Y setpT", "Leiden CF900\\VRM Y Status", "Leiden CF900\\VRM Y sweep", "Leiden CF900\\VRM Y sweep A", "Leiden CF900\\VRM Z at rest", "Leiden CF900\\VRM Z magA", "Leiden CF900\\VRM Z magT", "Leiden CF900\\VRM Z meas A", "Leiden CF900\\VRM Z meas V", "Leiden CF900\\VRM Z outA", "Leiden CF900\\VRM Z outT", "Leiden CF900\\VRM Z setpT", "Leiden CF900\\VRM Z Status", "Leiden CF900\\VRM Z sweep", "Leiden CF900\\VRM Z sweep A", "MFP3D\\MFP3D Hum", "MFP3D\\MFP3D Temperature", "MFP3D\\MFP3D TSP01 Hum", "MFP3D\\MFP3D TSP01 Temperature", "MFP3D\\MFP3D User", "MNK_18T\\1820_IPS_Current", "MNK_18T\\1820_IPS_Level_He", "MNK_18T\\1820_IPS_Level_N2", "MNK_18T\\1820_IPS_M1_Current", "MNK_18T\\1820_IPS_M1_Voltage", "MNK_18T\\1820_IPS_M2_Current", "MNK_18T\\1820_IPS_M2_Voltage", "MNK_18T\\1820_IPS_M3_Current", "MNK_18T\\1820_IPS_M3_Voltage", "MNK_18T\\1820_IPS_Magnet_Field", "MNK_18T\\1820_IPS_Magnet_Temperature", "MNK_18T\\1820_IPS_Magnet_Temperature_R", "MNK_18T\\1820_IPS_PS_Field", "MNK_18T\\1820_IPS_Reply", "MNK_18T\\1820_IPS_Status", "MNK_18T\\1820_IPS_Switch", "MNK_18T\\1820_IPS_Target_Field", "MNK_18T\\1820_IPS_Target_Field_Rate", "MNK_18T\\1820_IPS_Voltage", "MNK_18T\\1820_ITC_Lambda_Status", "MNK_18T\\1820_ITC_Lambda_Temperature", "MNK_18T\\1820_ITC_Lambda_Temperature_R", "MNK_18T\\1820_ITC_Needle_Valve", "MNK_18T\\1820_ITC_Pressure", "MNK_18T\\1820_ITC_Reply", "MNK_18T\\KH_ch1", "MNK_18T\\KH_ch2", "MNK_18T\\KH_ch3", "MNK_18T\\KH_ch4", "MNK_18T\\KH_ch5", "MNK_18T\\KH_ch6", "MNK_18T\\KH_ch7", "MNK_18T\\KH_ch8", "MNK_18T\\Lockin_Results", "MNK_18T\\MNK_CMN-187_T", "MNK_18T\\MNK_CMN-187_Z", "MNK_18T\\MNK_Cstill_T", "MNK_18T\\MNK_Cstill_Z", "MNK_18T\\MNK_FP_Flow", "MNK_18T\\MNK_FP_MG0", "MNK_18T\\MNK_FP_MG1", "MNK_18T\\MNK_FP_MG2", "MNK_18T\\MNK_FP_MG3", "MNK_18T\\MNK_FP_MG4", "MNK_18T\\MNK_FP_MG5", "MNK_18T\\MNK_FP_P1", "MNK_18T\\MNK_FP_P2", "MNK_18T\\MNK_FP_P3", "MNK_18T\\MNK_FP_P4", "MNK_18T\\MNK_FP_P5", "MNK_18T\\MNK_FP_P6", "MNK_18T\\MNK_FP_P7", "MNK_18T\\MNK_FP_STATE", "MNK_18T\\MNK_FP_State0", "MNK_18T\\MNK_FP_State1", "MNK_18T\\MNK_FP_State2", "MNK_18T\\MNK_TC_calibration", "MNK_18T\\MNK_TC_description", "MNK_18T\\MNK_TC_I0", "MNK_18T\\MNK_TC_I1", "MNK_18T\\MNK_TC_I2", "MNK_18T\\MNK_TC_I3", "MNK_18T\\MNK_TC_R0", "MNK_18T\\MNK_TC_R1", "MNK_18T\\MNK_TC_R2", "MNK_18T\\MNK_TC_R3", "MNK_18T\\MNK_TC_R4", "MNK_18T\\MNK_TC_R5", "MNK_18T\\MNK_TC_R6", "MNK_18T\\MNK_TC_R7", "MNK_18T\\MNK_TC_T0", "MNK_18T\\MNK_TC_T1", "MNK_18T\\MNK_TC_T2", "MNK_18T\\MNK_TC_T3", "MNK_18T\\MNK_TC_T4", "MNK_18T\\MNK_TC_T5", "MNK_18T\\MNK_TC_T6", "MNK_18T\\MNK_TC_T7", "MNK_18T\\MNK_TC_Z_calibration", "MNK_18T\\MNK_TC_Z_description", "MNK_18T\\OSC_config", "MNK_18T\\Vbg", "Montana THZ 1\\THZ 1 Dew Point", "Montana THZ 1\\THZ 1 Humidity", "Montana THZ 1\\THZ 1 Temperature", "OneNote API HTTP\\Access Token 0000000048124379", "OneNote API HTTP\\Asana Access Token 15669051163913", "PPMS 1\\PPMS 1 Magnetic Field", "PPMS 1\\PPMS 1 Temperature", "PPMS 2\\PPMS 2 Flow Rate", "PPMS 2\\PPMS 2 Helium Level", "PPMS 2\\PPMS 2 Magnetic Field", "PPMS 2\\PPMS 2 Position", "PPMS 2\\PPMS 2 Sys Pressure", "PPMS 2\\PPMS 2 Temperature", "PPMS 2\\PPMS 2 Vbg", "PPMS2\\PPMS2 Annulus Pres (Torr)", "PPMS2\\PPMS2 Annulus Vacuum (V)", "PPMS2\\PPMS2 Block Htr Cur (mA)", "PPMS2\\PPMS2 Block Htr Pwr (W)", "PPMS2\\PPMS2 BlockHeater(Ohm)", "PPMS2\\PPMS2 Bridge 1 Excitation (uA)", "PPMS2\\PPMS2 Bridge 1 Resistance (ohms)", "PPMS2\\PPMS2 Bridge 2 Excitation (uA)", "PPMS2\\PPMS2 Bridge 2 Resistance (ohms)", "PPMS2\\PPMS2 Bridge 3 Excitation (uA)", "PPMS2\\PPMS2 Bridge 3 Resistance (ohms)", "PPMS2\\PPMS2 Bridge 4 Excitation (uA)", "PPMS2\\PPMS2 Bridge 4 Resistance (ohms)", "PPMS2\\PPMS2 CIG Cernox (K)", "PPMS2\\PPMS2 CIG Excit (uA)", "PPMS2\\PPMS2 Comment", "PPMS2\\PPMS2 DAC  I  (cnts)", "PPMS2\\PPMS2 Digital Inputs (code)", "PPMS2\\PPMS2 Drive 1 Iout (mA)", "PPMS2\\PPMS2 Drive 1 Ipower (watts)", "PPMS2\\PPMS2 Drive 2 Iout (mA)", "PPMS2\\PPMS2 Drive 2 Ipower (watts)", "PPMS2\\PPMS2 EXT Flow (L min)", "PPMS2\\PPMS2 Flapper state", "PPMS2\\PPMS2 Flow Rate (l min)", "PPMS2\\PPMS2 He Level ()", "PPMS2\\PPMS2 Hi res (A) read", "PPMS2\\PPMS2 High Vacuum mode", "PPMS2\\PPMS2 Hires enable", "PPMS2\\PPMS2 Impedance (mode)", "PPMS2\\PPMS2 iso flag", "PPMS2\\PPMS2 KRPMs", "PPMS2\\PPMS2 Last 2 eng st", "PPMS2\\PPMS2 Log", "PPMS2\\PPMS2 Mag (V) read", "PPMS2\\PPMS2 Mag (V) set", "PPMS2\\PPMS2 Mag adj sc(I)set", "PPMS2\\PPMS2 Magnet (Oe)", "PPMS2\\PPMS2 Magnetic Field (Oe)", "PPMS2\\PPMS2 Map 20 ()", "PPMS2\\PPMS2 Map 21 ()", "PPMS2\\PPMS2 Map 22 ()", "PPMS2\\PPMS2 Map 23 ()", "PPMS2\\PPMS2 Map 24 ()", "PPMS2\\PPMS2 Map 25 ()", "PPMS2\\PPMS2 Map 26 ()", "PPMS2\\PPMS2 Map 27 ()", "PPMS2\\PPMS2 Map 28 ()", "PPMS2\\PPMS2 Map 29 ()", "PPMS2\\PPMS2 Map 67 ()", "PPMS2\\PPMS2 Map 68 ()", "PPMS2\\PPMS2 Map 69 ()", "PPMS2\\PPMS2 Map 89 ()", "PPMS2\\PPMS2 Map 90 ()", "PPMS2\\PPMS2 Map 91 ()", "PPMS2\\PPMS2 Map 92 ()", "PPMS2\\PPMS2 Map 93 ()", "PPMS2\\PPMS2 Neck Excit (uA)", "PPMS2\\PPMS2 Neck Htr Cur (mA)", "PPMS2\\PPMS2 Neck Htr Pwr (W)", "PPMS2\\PPMS2 Neck Therm (K)", "PPMS2\\PPMS2 NeckHeater(Ohm)", "PPMS2\\PPMS2 Plat Excit (uA)", "PPMS2\\PPMS2 Plat Therm (K)", "PPMS2\\PPMS2 Pressure ()", "PPMS2\\PPMS2 PSU Field (Oe)", "PPMS2\\PPMS2 Pump power (W)", "PPMS2\\PPMS2 Pump temp (C)", "PPMS2\\PPMS2 Redirected 55 ()", "PPMS2\\PPMS2 Redirected 56 ()", "PPMS2\\PPMS2 Redirected 57 ()", "PPMS2\\PPMS2 Redirected 58 ()", "PPMS2\\PPMS2 Redirected 59 ()", "PPMS2\\PPMS2 Redirected 61 ()", "PPMS2\\PPMS2 Regen htr flag", "PPMS2\\PPMS2 Sample Position (deg)", "PPMS2\\PPMS2 Seq Stat ()", "PPMS2\\PPMS2 Setpoint (K)", "PPMS2\\PPMS2 Signal 1 Vin (V)", "PPMS2\\PPMS2 Signal 2 Vin (V)", "PPMS2\\PPMS2 Spare Excit (uA)", "PPMS2\\PPMS2 Spare Therm (K)", "PPMS2\\PPMS2 Status (code)", "PPMS2\\PPMS2 Sw heater state", "PPMS2\\PPMS2 Sys Temp ()", "PPMS2\\PPMS2 System Pres (Torr)", "PPMS2\\PPMS2 System Status (code)", "PPMS2\\PPMS2 Tableless Map53 ()", "PPMS2\\PPMS2 Tableless Map54 ()", "PPMS2\\PPMS2 Temperature (K)", "PPMS2\\PPMS2 Therm v", "PPMS2\\PPMS2 Time Stamp (sec)", "PPMS2\\PPMS2 Valve Position (deg)", "PPMSDR\\PPMSDR Annulus Pres (Torr)", "PPMSDR\\PPMSDR Annulus Vacuum (V)", "PPMSDR\\PPMSDR Block Htr Cur (mA)", "PPMSDR\\PPMSDR Block Htr Pwr (W)", "PPMSDR\\PPMSDR BlockHeater(Ohm)", "PPMSDR\\PPMSDR Bridge 1 Excitation (uA)", "PPMSDR\\PPMSDR Bridge 1 Resistance (ohms)", "PPMSDR\\PPMSDR Bridge 2 Excitation (uA)", "PPMSDR\\PPMSDR Bridge 2 Resistance (ohms)", "PPMSDR\\PPMSDR Bridge 3 Excitation (uA)", "PPMSDR\\PPMSDR Bridge 3 Resistance (ohms)", "PPMSDR\\PPMSDR Bridge 4 Excitation (uA)", "PPMSDR\\PPMSDR Bridge 4 Resistance (ohms)", "PPMSDR\\PPMSDR CIG Cernox (K)", "PPMSDR\\PPMSDR CIG Excit (uA)", "PPMSDR\\PPMSDR Comment", "PPMSDR\\PPMSDR DAC  I  (cnts)", "PPMSDR\\PPMSDR Digital Inputs (code)", "PPMSDR\\PPMSDR Drive 1 Iout (mA)", "PPMSDR\\PPMSDR Drive 1 Ipower (watts)", "PPMSDR\\PPMSDR Drive 2 Iout (mA)", "PPMSDR\\PPMSDR Drive 2 Ipower (watts)", "PPMSDR\\PPMSDR EXT Flow (L min)", "PPMSDR\\PPMSDR Flapper state", "PPMSDR\\PPMSDR Flow Rate (l min)", "PPMSDR\\PPMSDR He Level ()", "PPMSDR\\PPMSDR Hi res (A) read", "PPMSDR\\PPMSDR High Vacuum mode", "PPMSDR\\PPMSDR Hires enable", "PPMSDR\\PPMSDR Impedance (mode)", "PPMSDR\\PPMSDR iso flag", "PPMSDR\\PPMSDR KRPMs", "PPMSDR\\PPMSDR Last 2 eng st", "PPMSDR\\PPMSDR Log", "PPMSDR\\PPMSDR low res (A) read", "PPMSDR\\PPMSDR Mag (V) read", "PPMSDR\\PPMSDR Mag (V) set", "PPMSDR\\PPMSDR Mag adj sc(I)set", "PPMSDR\\PPMSDR Magnet (Oe)", "PPMSDR\\PPMSDR Magnetic Field (Oe)", "PPMSDR\\PPMSDR MAP 1", "PPMSDR\\PPMSDR MAP 10", "PPMSDR\\PPMSDR MAP 11", "PPMSDR\\PPMSDR MAP 12", "PPMSDR\\PPMSDR MAP 13", "PPMSDR\\PPMSDR MAP 14", "PPMSDR\\PPMSDR MAP 15", "PPMSDR\\PPMSDR MAP 16", "PPMSDR\\PPMSDR MAP 17", "PPMSDR\\PPMSDR MAP 18", "PPMSDR\\PPMSDR MAP 19", "PPMSDR\\PPMSDR MAP 2", "PPMSDR\\PPMSDR MAP 20", "PPMSDR\\PPMSDR Map 20 ()", "PPMSDR\\PPMSDR MAP 21", "PPMSDR\\PPMSDR Map 21 ()", "PPMSDR\\PPMSDR MAP 22", "PPMSDR\\PPMSDR Map 22 ()", "PPMSDR\\PPMSDR MAP 23", "PPMSDR\\PPMSDR Map 23 ()", "PPMSDR\\PPMSDR MAP 24", "PPMSDR\\PPMSDR Map 24 ()", "PPMSDR\\PPMSDR MAP 25", "PPMSDR\\PPMSDR Map 25 ()", "PPMSDR\\PPMSDR MAP 26", "PPMSDR\\PPMSDR Map 26 ()", "PPMSDR\\PPMSDR MAP 27", "PPMSDR\\PPMSDR Map 27 ()", "PPMSDR\\PPMSDR MAP 28", "PPMSDR\\PPMSDR Map 28 ()", "PPMSDR\\PPMSDR MAP 29", "PPMSDR\\PPMSDR Map 29 ()", "PPMSDR\\PPMSDR MAP 3", "PPMSDR\\PPMSDR MAP 30", "PPMSDR\\PPMSDR MAP 4", "PPMSDR\\PPMSDR MAP 5", "PPMSDR\\PPMSDR MAP 6", "PPMSDR\\PPMSDR Map 67 ()", "PPMSDR\\PPMSDR Map 68 ()", "PPMSDR\\PPMSDR Map 69 ()", "PPMSDR\\PPMSDR MAP 7", "PPMSDR\\PPMSDR MAP 8", "PPMSDR\\PPMSDR Map 89 ()", "PPMSDR\\PPMSDR MAP 9", "PPMSDR\\PPMSDR Map 90 ()", "PPMSDR\\PPMSDR Map 91 ()", "PPMSDR\\PPMSDR Map 92 ()", "PPMSDR\\PPMSDR Map 93 ()", "PPMSDR\\PPMSDR Neck Excit (uA)", "PPMSDR\\PPMSDR Neck Htr Cur (mA)", "PPMSDR\\PPMSDR Neck Htr Pwr (W)", "PPMSDR\\PPMSDR Neck Therm (K)", "PPMSDR\\PPMSDR NeckHeater(Ohm)", "PPMSDR\\PPMSDR Plat Excit (uA)", "PPMSDR\\PPMSDR Plat Therm (K)", "PPMSDR\\PPMSDR Pressure ()", "PPMSDR\\PPMSDR Pump power (W)", "PPMSDR\\PPMSDR Pump temp (C)", "PPMSDR\\PPMSDR Redirected 55 ()", "PPMSDR\\PPMSDR Redirected 56 ()", "PPMSDR\\PPMSDR Redirected 57 ()", "PPMSDR\\PPMSDR Redirected 58 ()", "PPMSDR\\PPMSDR Redirected 59 ()", "PPMSDR\\PPMSDR Redirected 61 ()", "PPMSDR\\PPMSDR Regen htr flag", "PPMSDR\\PPMSDR Sample Position (deg)", "PPMSDR\\PPMSDR Seq Stat ()", "PPMSDR\\PPMSDR Setpoint (K)", "PPMSDR\\PPMSDR Signal 1 Vin (V)", "PPMSDR\\PPMSDR Signal 2 Vin (V)", "PPMSDR\\PPMSDR Spare Excit (uA)", "PPMSDR\\PPMSDR Spare Therm (K)", "PPMSDR\\PPMSDR Status (code)", "PPMSDR\\PPMSDR Sw heater state", "PPMSDR\\PPMSDR Sys Temp ()", "PPMSDR\\PPMSDR System Pres (Torr)", "PPMSDR\\PPMSDR System Status (code)", "PPMSDR\\PPMSDR Tableless Map53 ()", "PPMSDR\\PPMSDR Tableless Map54 ()", "PPMSDR\\PPMSDR Temperature (K)", "PPMSDR\\PPMSDR Therm v", "PPMSDR\\PPMSDR Time Stamp (sec)", "PPMSDR\\PPMSDR Valve Position (deg)", "Sample Characterization\\2G Conductance", "Sample Characterization\\4G", "Sample Characterization\\4R", "Sample Characterization\\CURRENT", "Sample Characterization\\Experiment ID", "Sample Characterization\\Notes", "Sample Characterization\\OSCILLATION VOLTAGE", "Sample Characterization\\Sample Name", "Sample Characterization\\V1", "Sample Characterization\\V2", "SPM\\Laser Power", "SPM\\SPM scanner X", "SPM\\SPM scanner Y", "TEMPerHUM\\MFP : Humidity", "TEMPerHUM\\MFP : ID", "TEMPerHUM\\MFP : Location", "TEMPerHUM\\MFP : Picture URL", "TEMPerHUM\\MFP : Temperature", "TEMPerHUM\\MFP-3D : Humidity", "TEMPerHUM\\MFP-3D : ID", "TEMPerHUM\\MFP-3D : Location", "TEMPerHUM\\MFP-3D : Picture URL", "TEMPerHUM\\MFP-3D : Temperature", "TEMPerHUM\\TEST3 : Humidity", "TEMPerHUM\\TEST3 : ID", "TEMPerHUM\\TEST3 : Location", "TEMPerHUM\\TEST3 : Picture URL", "TEMPerHUM\\TEST3 : Temperature"]
  in  "Favorite B (Right)":u16[](array[ring])=[172] items=["Attocube 3DR\\axis 1: Amplitude", "Attocube 3DR\\axis 1: Capacitance", "Attocube 3DR\\axis 1: control mode", "Attocube 3DR\\axis 1: current position", "Attocube 3DR\\axis 1: DCLevel", "Attocube 3DR\\axis 1: Frequency", "Attocube 3DR\\axis 1: moving", "Attocube 3DR\\axis 1: Output", "Attocube 3DR\\axis 1: rot. count", "Attocube 3DR\\axis 1: sensor disconnected", "Attocube 3DR\\axis 1: sensor error", "Attocube 3DR\\axis 1: Single Circle Mode", "Attocube 3DR\\axis 1: sp position", "Attocube 3DR\\axis 1: sp rot count", "Attocube 3DR\\axis 1: speed", "Attocube 3DR\\axis 1: StepWidth", "Attocube 3DR\\axis 1: stop detected", "Attocube 3DR\\axis 1: stop enable", "Attocube 3DR\\axis 1: Target GND", "Attocube 3DR\\axis 2: Amplitude", "Attocube 3DR\\axis 2: Capacitance", "Attocube 3DR\\axis 2: control mode", "Attocube 3DR\\axis 2: current position", "Attocube 3DR\\axis 2: DCLevel", "Attocube 3DR\\axis 2: Frequency", "Attocube 3DR\\axis 2: moving", "Attocube 3DR\\axis 2: Output", "Attocube 3DR\\axis 2: rot. count", "Attocube 3DR\\axis 2: sensor disconnected", "Attocube 3DR\\axis 2: sensor error", "Attocube 3DR\\axis 2: Single Circle Mode", "Attocube 3DR\\axis 2: sp position", "Attocube 3DR\\axis 2: sp rot count", "Attocube 3DR\\axis 2: speed", "Attocube 3DR\\axis 2: StepWidth", "Attocube 3DR\\axis 2: stop detected", "Attocube 3DR\\axis 2: stop enable", "Attocube 3DR\\axis 2: Target GND", "Attocube 3DR\\static amplitude", "Cypher\\Cypher RH1", "Cypher\\Cypher RH2", "Cypher\\Cypher Temperature", "Cypher\\Cypher_Funnel_Property", "Cypher\\Cypher_Path_Property", "Cypher\\Cypher_Rectangle_Property", "DR200\\DR200_Magnet_Field", "DR200\\DR200_Magnet_Field_Target", "DR200\\DR200_Magnet_PS_Current", "DR200\\DR200_Magnet_PS_Field", "DR200\\DR200_Magnet_PS_Voltage", "DR200\\DR200_Magnet_Rate_Target", "DR200\\DR200_Magnet_Status_Activity", "DR200\\DR200_Magnet_Status_Mode", "DR200\\DR200_Magnet_Status_Switch_Heater", "DR200\\DR200_Magnet_Status_System", "JLevy\\Levy 1", "Leiden CF900\\CF Impedance CMN", "Leiden CF900\\CF_FP_STATE", "Leiden CF900\\CF_KH_ch1", "Leiden CF900\\CF_KH_ch2", "Leiden CF900\\CF_KH_ch3", "Leiden CF900\\CF_KH_ch4", "Leiden CF900\\CF_KH_ch5", "Leiden CF900\\CF_KH_ch6", "Leiden CF900\\CF_KH_ch7", "Leiden CF900\\CF_KH_ch8", "Leiden CF900\\CF_TC_calibration", "Leiden CF900\\CF_TC_description", "Leiden CF900\\CF_TC_Z_calibration", "Leiden CF900\\CF_TC_Z_description", "Leiden CF900\\CF_TC_Z_R0", "Leiden CF900\\CF_TC_Z_R1", "Leiden CF900\\CF_TC_Z_R2", "Leiden CF900\\CF_TC_Z_R3", "Leiden CF900\\CF_TC_Z_R4", "Leiden CF900\\CF_TC_Z_R5", "Leiden CF900\\CF_TC_Z_R6", "Leiden CF900\\CF_TC_Z_R7", "Leiden CF900\\CF_TC_Z_R8", "Leiden CF900\\CF_TC_Z_R9", "Leiden CF900\\CF_TC_Z_T0", "Leiden CF900\\CF_TC_Z_T1", "Leiden CF900\\CF_TC_Z_T2", "Leiden CF900\\CF_TC_Z_T3", "Leiden CF900\\CF_TC_Z_T4", "Leiden CF900\\CF_TC_Z_T5", "Leiden CF900\\CF_TC_Z_T6", "Leiden CF900\\CF_TC_Z_T7", "Leiden CF900\\CF_TC_Z_T8", "Leiden CF900\\CF_TC_Z_T9", "Leiden CF900\\CF900_Cstill", "Leiden CF900\\Leiden CF FP\\CF FP Flow", "Leiden CF900\\Leiden CF FP\\CF FP He", "Leiden CF900\\Leiden CF FP\\CF FP MG0", "Leiden CF900\\Leiden CF FP\\CF FP MG1", "Leiden CF900\\Leiden CF FP\\CF FP MG2", "Leiden CF900\\Leiden CF FP\\CF FP MG3", "Leiden CF900\\Leiden CF FP\\CF FP MG4", "Leiden CF900\\Leiden CF FP\\CF FP MG5", "Leiden CF900\\Leiden CF FP\\CF FP oil", "Leiden CF900\\Leiden CF FP\\CF FP P_high", "Leiden CF900\\Leiden CF FP\\CF FP P_low", "Leiden CF900\\Leiden CF FP\\CF FP P1", "Leiden CF900\\Leiden CF FP\\CF FP P2", "Leiden CF900\\Leiden CF FP\\CF FP P3", "Leiden CF900\\Leiden CF FP\\CF FP P4", "Leiden CF900\\Leiden CF FP\\CF FP P5", "Leiden CF900\\Leiden CF FP\\CF FP P6", "Leiden CF900\\Leiden CF FP\\CF FP P7", "Leiden CF900\\Leiden CF FP\\CF FP PT current", "Leiden CF900\\Leiden CF FP\\CF FP PT on", "Leiden CF900\\Leiden CF FP\\CF FP State0", "Leiden CF900\\Leiden CF FP\\CF FP State1", "Leiden CF900\\Leiden CF FP\\CF FP State2", "Leiden CF900\\Leiden CF FP\\CF FP W_in", "Leiden CF900\\Leiden CF FP\\CF FP W_out", "Leiden CF900\\Leiden CF Impedance Bridge\\CF IB TA", "Leiden CF900\\Leiden CF Impedance Bridge\\CF IB TB", "Leiden CF900\\Leiden CF Impedance Bridge\\CF IB TC", "Leiden CF900\\Leiden CF Impedance Bridge\\CF IB TD", "Leiden CF900\\Leiden CF Impedance Bridge\\CF IB TE", "Leiden CF900\\Leiden CF Magnetic Field\\CF Field X", "Leiden CF900\\Leiden CF Magnetic Field\\CF Field Y", "Leiden CF900\\Leiden CF Magnetic Field\\CF Field Z", "Leiden CF900\\Leiden CF TC\\CF TC I0", "Leiden CF900\\Leiden CF TC\\CF TC I1", "Leiden CF900\\Leiden CF TC\\CF TC I2", "Leiden CF900\\Leiden CF TC\\CF TC I3", "Leiden CF900\\Leiden CF TC\\CF TC R0", "Leiden CF900\\Leiden CF TC\\CF TC R1", "Leiden CF900\\Leiden CF TC\\CF TC R2", "Leiden CF900\\Leiden CF TC\\CF TC R3", "Leiden CF900\\Leiden CF TC\\CF TC R4", "Leiden CF900\\Leiden CF TC\\CF TC R5", "Leiden CF900\\Leiden CF TC\\CF TC R6", "Leiden CF900\\Leiden CF TC\\CF TC R7", "Leiden CF900\\Leiden CF TC\\CF TC T0", "Leiden CF900\\Leiden CF TC\\CF TC T1", "Leiden CF900\\Leiden CF TC\\CF TC T2", "Leiden CF900\\Leiden CF TC\\CF TC T3", "Leiden CF900\\Leiden CF TC\\CF TC T4", "Leiden CF900\\Leiden CF TC\\CF TC T5", "Leiden CF900\\Leiden CF TC\\CF TC T6", "Leiden CF900\\Leiden CF TC\\CF TC T7", "Leiden CF900\\RuO2_T", "Leiden CF900\\RuO2_Z", "Leiden CF900\\Vbg", "Leiden CF900\\VRM VrmSweepMode", "Leiden CF900\\VRM VrmSweepRate", "Leiden CF900\\VRM VrmSweepTime", "Leiden CF900\\VRM VrmX setpT", "Leiden CF900\\VRM VrmY setpT", "Leiden CF900\\VRM VrmZ setpT", "Leiden CF900\\VRM X at rest", "Leiden CF900\\VRM X magA", "Leiden CF900\\VRM X magT", "Leiden CF900\\VRM X meas A", "Leiden CF900\\VRM X meas V", "Leiden CF900\\VRM X outA", "Leiden CF900\\VRM X outT", "Leiden CF900\\VRM X setpT", "Leiden CF900\\VRM X Status", "Leiden CF900\\VRM X sweep", "Leiden CF900\\VRM X sweep A", "Leiden CF900\\VRM Y at rest", "Leiden CF900\\VRM Y magA", "Leiden CF900\\VRM Y magT", "Leiden CF900\\VRM Y meas A", "Leiden CF900\\VRM Y meas V", "Leiden CF900\\VRM Y outA", "Leiden CF900\\VRM Y outT", "Leiden CF900\\VRM Y setpT", "Leiden CF900\\VRM Y Status", "Leiden CF900\\VRM Y sweep", "Leiden CF900\\VRM Y sweep A", "Leiden CF900\\VRM Z at rest", "Leiden CF900\\VRM Z magA", "Leiden CF900\\VRM Z magT", "Leiden CF900\\VRM Z meas A", "Leiden CF900\\VRM Z meas V", "Leiden CF900\\VRM Z outA", "Leiden CF900\\VRM Z outT", "Leiden CF900\\VRM Z setpT", "Leiden CF900\\VRM Z Status", "Leiden CF900\\VRM Z sweep", "Leiden CF900\\VRM Z sweep A", "MFP3D\\MFP3D Hum", "MFP3D\\MFP3D Temperature", "MFP3D\\MFP3D TSP01 Hum", "MFP3D\\MFP3D TSP01 Temperature", "MFP3D\\MFP3D User", "MNK_18T\\1820_IPS_Current", "MNK_18T\\1820_IPS_Level_He", "MNK_18T\\1820_IPS_Level_N2", "MNK_18T\\1820_IPS_M1_Current", "MNK_18T\\1820_IPS_M1_Voltage", "MNK_18T\\1820_IPS_M2_Current", "MNK_18T\\1820_IPS_M2_Voltage", "MNK_18T\\1820_IPS_M3_Current", "MNK_18T\\1820_IPS_M3_Voltage", "MNK_18T\\1820_IPS_Magnet_Field", "MNK_18T\\1820_IPS_Magnet_Temperature", "MNK_18T\\1820_IPS_Magnet_Temperature_R", "MNK_18T\\1820_IPS_PS_Field", "MNK_18T\\1820_IPS_Reply", "MNK_18T\\1820_IPS_Status", "MNK_18T\\1820_IPS_Switch", "MNK_18T\\1820_IPS_Target_Field", "MNK_18T\\1820_IPS_Target_Field_Rate", "MNK_18T\\1820_IPS_Voltage", "MNK_18T\\1820_ITC_Lambda_Status", "MNK_18T\\1820_ITC_Lambda_Temperature", "MNK_18T\\1820_ITC_Lambda_Temperature_R", "MNK_18T\\1820_ITC_Needle_Valve", "MNK_18T\\1820_ITC_Pressure", "MNK_18T\\1820_ITC_Reply", "MNK_18T\\KH_ch1", "MNK_18T\\KH_ch2", "MNK_18T\\KH_ch3", "MNK_18T\\KH_ch4", "MNK_18T\\KH_ch5", "MNK_18T\\KH_ch6", "MNK_18T\\KH_ch7", "MNK_18T\\KH_ch8", "MNK_18T\\Lockin_Results", "MNK_18T\\MNK_CMN-187_T", "MNK_18T\\MNK_CMN-187_Z", "MNK_18T\\MNK_Cstill_T", "MNK_18T\\MNK_Cstill_Z", "MNK_18T\\MNK_FP_Flow", "MNK_18T\\MNK_FP_MG0", "MNK_18T\\MNK_FP_MG1", "MNK_18T\\MNK_FP_MG2", "MNK_18T\\MNK_FP_MG3", "MNK_18T\\MNK_FP_MG4", "MNK_18T\\MNK_FP_MG5", "MNK_18T\\MNK_FP_P1", "MNK_18T\\MNK_FP_P2", "MNK_18T\\MNK_FP_P3", "MNK_18T\\MNK_FP_P4", "MNK_18T\\MNK_FP_P5", "MNK_18T\\MNK_FP_P6", "MNK_18T\\MNK_FP_P7", "MNK_18T\\MNK_FP_STATE", "MNK_18T\\MNK_FP_State0", "MNK_18T\\MNK_FP_State1", "MNK_18T\\MNK_FP_State2", "MNK_18T\\MNK_TC_calibration", "MNK_18T\\MNK_TC_description", "MNK_18T\\MNK_TC_I0", "MNK_18T\\MNK_TC_I1", "MNK_18T\\MNK_TC_I2", "MNK_18T\\MNK_TC_I3", "MNK_18T\\MNK_TC_R0", "MNK_18T\\MNK_TC_R1", "MNK_18T\\MNK_TC_R2", "MNK_18T\\MNK_TC_R3", "MNK_18T\\MNK_TC_R4", "MNK_18T\\MNK_TC_R5", "MNK_18T\\MNK_TC_R6", "MNK_18T\\MNK_TC_R7", "MNK_18T\\MNK_TC_T0", "MNK_18T\\MNK_TC_T1", "MNK_18T\\MNK_TC_T2", "MNK_18T\\MNK_TC_T3", "MNK_18T\\MNK_TC_T4", "MNK_18T\\MNK_TC_T5", "MNK_18T\\MNK_TC_T6", "MNK_18T\\MNK_TC_T7", "MNK_18T\\MNK_TC_Z_calibration", "MNK_18T\\MNK_TC_Z_description", "MNK_18T\\OSC_config", "MNK_18T\\Vbg", "Montana THZ 1\\THZ 1 Dew Point", "Montana THZ 1\\THZ 1 Humidity", "Montana THZ 1\\THZ 1 Temperature", "OneNote API HTTP\\Access Token 0000000048124379", "OneNote API HTTP\\Asana Access Token 15669051163913", "PPMS 1\\PPMS 1 Magnetic Field", "PPMS 1\\PPMS 1 Temperature", "PPMS 2\\PPMS 2 Flow Rate", "PPMS 2\\PPMS 2 Helium Level", "PPMS 2\\PPMS 2 Magnetic Field", "PPMS 2\\PPMS 2 Position", "PPMS 2\\PPMS 2 Sys Pressure", "PPMS 2\\PPMS 2 Temperature", "PPMS 2\\PPMS 2 Vbg", "PPMS2\\PPMS2 Annulus Pres (Torr)", "PPMS2\\PPMS2 Annulus Vacuum (V)", "PPMS2\\PPMS2 Block Htr Cur (mA)", "PPMS2\\PPMS2 Block Htr Pwr (W)", "PPMS2\\PPMS2 BlockHeater(Ohm)", "PPMS2\\PPMS2 Bridge 1 Excitation (uA)", "PPMS2\\PPMS2 Bridge 1 Resistance (ohms)", "PPMS2\\PPMS2 Bridge 2 Excitation (uA)", "PPMS2\\PPMS2 Bridge 2 Resistance (ohms)", "PPMS2\\PPMS2 Bridge 3 Excitation (uA)", "PPMS2\\PPMS2 Bridge 3 Resistance (ohms)", "PPMS2\\PPMS2 Bridge 4 Excitation (uA)", "PPMS2\\PPMS2 Bridge 4 Resistance (ohms)", "PPMS2\\PPMS2 CIG Cernox (K)", "PPMS2\\PPMS2 CIG Excit (uA)", "PPMS2\\PPMS2 Comment", "PPMS2\\PPMS2 DAC  I  (cnts)", "PPMS2\\PPMS2 Digital Inputs (code)", "PPMS2\\PPMS2 Drive 1 Iout (mA)", "PPMS2\\PPMS2 Drive 1 Ipower (watts)", "PPMS2\\PPMS2 Drive 2 Iout (mA)", "PPMS2\\PPMS2 Drive 2 Ipower (watts)", "PPMS2\\PPMS2 EXT Flow (L min)", "PPMS2\\PPMS2 Flapper state", "PPMS2\\PPMS2 Flow Rate (l min)", "PPMS2\\PPMS2 He Level ()", "PPMS2\\PPMS2 Hi res (A) read", "PPMS2\\PPMS2 High Vacuum mode", "PPMS2\\PPMS2 Hires enable", "PPMS2\\PPMS2 Impedance (mode)", "PPMS2\\PPMS2 iso flag", "PPMS2\\PPMS2 KRPMs", "PPMS2\\PPMS2 Last 2 eng st", "PPMS2\\PPMS2 Log", "PPMS2\\PPMS2 Mag (V) read", "PPMS2\\PPMS2 Mag (V) set", "PPMS2\\PPMS2 Mag adj sc(I)set", "PPMS2\\PPMS2 Magnet (Oe)", "PPMS2\\PPMS2 Magnetic Field (Oe)", "PPMS2\\PPMS2 Map 20 ()", "PPMS2\\PPMS2 Map 21 ()", "PPMS2\\PPMS2 Map 22 ()", "PPMS2\\PPMS2 Map 23 ()", "PPMS2\\PPMS2 Map 24 ()", "PPMS2\\PPMS2 Map 25 ()", "PPMS2\\PPMS2 Map 26 ()", "PPMS2\\PPMS2 Map 27 ()", "PPMS2\\PPMS2 Map 28 ()", "PPMS2\\PPMS2 Map 29 ()", "PPMS2\\PPMS2 Map 67 ()", "PPMS2\\PPMS2 Map 68 ()", "PPMS2\\PPMS2 Map 69 ()", "PPMS2\\PPMS2 Map 89 ()", "PPMS2\\PPMS2 Map 90 ()", "PPMS2\\PPMS2 Map 91 ()", "PPMS2\\PPMS2 Map 92 ()", "PPMS2\\PPMS2 Map 93 ()", "PPMS2\\PPMS2 Neck Excit (uA)", "PPMS2\\PPMS2 Neck Htr Cur (mA)", "PPMS2\\PPMS2 Neck Htr Pwr (W)", "PPMS2\\PPMS2 Neck Therm (K)", "PPMS2\\PPMS2 NeckHeater(Ohm)", "PPMS2\\PPMS2 Plat Excit (uA)", "PPMS2\\PPMS2 Plat Therm (K)", "PPMS2\\PPMS2 Pressure ()", "PPMS2\\PPMS2 PSU Field (Oe)", "PPMS2\\PPMS2 Pump power (W)", "PPMS2\\PPMS2 Pump temp (C)", "PPMS2\\PPMS2 Redirected 55 ()", "PPMS2\\PPMS2 Redirected 56 ()", "PPMS2\\PPMS2 Redirected 57 ()", "PPMS2\\PPMS2 Redirected 58 ()", "PPMS2\\PPMS2 Redirected 59 ()", "PPMS2\\PPMS2 Redirected 61 ()", "PPMS2\\PPMS2 Regen htr flag", "PPMS2\\PPMS2 Sample Position (deg)", "PPMS2\\PPMS2 Seq Stat ()", "PPMS2\\PPMS2 Setpoint (K)", "PPMS2\\PPMS2 Signal 1 Vin (V)", "PPMS2\\PPMS2 Signal 2 Vin (V)", "PPMS2\\PPMS2 Spare Excit (uA)", "PPMS2\\PPMS2 Spare Therm (K)", "PPMS2\\PPMS2 Status (code)", "PPMS2\\PPMS2 Sw heater state", "PPMS2\\PPMS2 Sys Temp ()", "PPMS2\\PPMS2 System Pres (Torr)", "PPMS2\\PPMS2 System Status (code)", "PPMS2\\PPMS2 Tableless Map53 ()", "PPMS2\\PPMS2 Tableless Map54 ()", "PPMS2\\PPMS2 Temperature (K)", "PPMS2\\PPMS2 Therm v", "PPMS2\\PPMS2 Time Stamp (sec)", "PPMS2\\PPMS2 Valve Position (deg)", "PPMSDR\\PPMSDR Annulus Pres (Torr)", "PPMSDR\\PPMSDR Annulus Vacuum (V)", "PPMSDR\\PPMSDR Block Htr Cur (mA)", "PPMSDR\\PPMSDR Block Htr Pwr (W)", "PPMSDR\\PPMSDR BlockHeater(Ohm)", "PPMSDR\\PPMSDR Bridge 1 Excitation (uA)", "PPMSDR\\PPMSDR Bridge 1 Resistance (ohms)", "PPMSDR\\PPMSDR Bridge 2 Excitation (uA)", "PPMSDR\\PPMSDR Bridge 2 Resistance (ohms)", "PPMSDR\\PPMSDR Bridge 3 Excitation (uA)", "PPMSDR\\PPMSDR Bridge 3 Resistance (ohms)", "PPMSDR\\PPMSDR Bridge 4 Excitation (uA)", "PPMSDR\\PPMSDR Bridge 4 Resistance (ohms)", "PPMSDR\\PPMSDR CIG Cernox (K)", "PPMSDR\\PPMSDR CIG Excit (uA)", "PPMSDR\\PPMSDR Comment", "PPMSDR\\PPMSDR DAC  I  (cnts)", "PPMSDR\\PPMSDR Digital Inputs (code)", "PPMSDR\\PPMSDR Drive 1 Iout (mA)", "PPMSDR\\PPMSDR Drive 1 Ipower (watts)", "PPMSDR\\PPMSDR Drive 2 Iout (mA)", "PPMSDR\\PPMSDR Drive 2 Ipower (watts)", "PPMSDR\\PPMSDR EXT Flow (L min)", "PPMSDR\\PPMSDR Flapper state", "PPMSDR\\PPMSDR Flow Rate (l min)", "PPMSDR\\PPMSDR He Level ()", "PPMSDR\\PPMSDR Hi res (A) read", "PPMSDR\\PPMSDR High Vacuum mode", "PPMSDR\\PPMSDR Hires enable", "PPMSDR\\PPMSDR Impedance (mode)", "PPMSDR\\PPMSDR iso flag", "PPMSDR\\PPMSDR KRPMs", "PPMSDR\\PPMSDR Last 2 eng st", "PPMSDR\\PPMSDR Log", "PPMSDR\\PPMSDR low res (A) read", "PPMSDR\\PPMSDR Mag (V) read", "PPMSDR\\PPMSDR Mag (V) set", "PPMSDR\\PPMSDR Mag adj sc(I)set", "PPMSDR\\PPMSDR Magnet (Oe)", "PPMSDR\\PPMSDR Magnetic Field (Oe)", "PPMSDR\\PPMSDR MAP 1", "PPMSDR\\PPMSDR MAP 10", "PPMSDR\\PPMSDR MAP 11", "PPMSDR\\PPMSDR MAP 12", "PPMSDR\\PPMSDR MAP 13", "PPMSDR\\PPMSDR MAP 14", "PPMSDR\\PPMSDR MAP 15", "PPMSDR\\PPMSDR MAP 16", "PPMSDR\\PPMSDR MAP 17", "PPMSDR\\PPMSDR MAP 18", "PPMSDR\\PPMSDR MAP 19", "PPMSDR\\PPMSDR MAP 2", "PPMSDR\\PPMSDR MAP 20", "PPMSDR\\PPMSDR Map 20 ()", "PPMSDR\\PPMSDR MAP 21", "PPMSDR\\PPMSDR Map 21 ()", "PPMSDR\\PPMSDR MAP 22", "PPMSDR\\PPMSDR Map 22 ()", "PPMSDR\\PPMSDR MAP 23", "PPMSDR\\PPMSDR Map 23 ()", "PPMSDR\\PPMSDR MAP 24", "PPMSDR\\PPMSDR Map 24 ()", "PPMSDR\\PPMSDR MAP 25", "PPMSDR\\PPMSDR Map 25 ()", "PPMSDR\\PPMSDR MAP 26", "PPMSDR\\PPMSDR Map 26 ()", "PPMSDR\\PPMSDR MAP 27", "PPMSDR\\PPMSDR Map 27 ()", "PPMSDR\\PPMSDR MAP 28", "PPMSDR\\PPMSDR Map 28 ()", "PPMSDR\\PPMSDR MAP 29", "PPMSDR\\PPMSDR Map 29 ()", "PPMSDR\\PPMSDR MAP 3", "PPMSDR\\PPMSDR MAP 30", "PPMSDR\\PPMSDR MAP 4", "PPMSDR\\PPMSDR MAP 5", "PPMSDR\\PPMSDR MAP 6", "PPMSDR\\PPMSDR Map 67 ()", "PPMSDR\\PPMSDR Map 68 ()", "PPMSDR\\PPMSDR Map 69 ()", "PPMSDR\\PPMSDR MAP 7", "PPMSDR\\PPMSDR MAP 8", "PPMSDR\\PPMSDR Map 89 ()", "PPMSDR\\PPMSDR MAP 9", "PPMSDR\\PPMSDR Map 90 ()", "PPMSDR\\PPMSDR Map 91 ()", "PPMSDR\\PPMSDR Map 92 ()", "PPMSDR\\PPMSDR Map 93 ()", "PPMSDR\\PPMSDR Neck Excit (uA)", "PPMSDR\\PPMSDR Neck Htr Cur (mA)", "PPMSDR\\PPMSDR Neck Htr Pwr (W)", "PPMSDR\\PPMSDR Neck Therm (K)", "PPMSDR\\PPMSDR NeckHeater(Ohm)", "PPMSDR\\PPMSDR Plat Excit (uA)", "PPMSDR\\PPMSDR Plat Therm (K)", "PPMSDR\\PPMSDR Pressure ()", "PPMSDR\\PPMSDR Pump power (W)", "PPMSDR\\PPMSDR Pump temp (C)", "PPMSDR\\PPMSDR Redirected 55 ()", "PPMSDR\\PPMSDR Redirected 56 ()", "PPMSDR\\PPMSDR Redirected 57 ()", "PPMSDR\\PPMSDR Redirected 58 ()", "PPMSDR\\PPMSDR Redirected 59 ()", "PPMSDR\\PPMSDR Redirected 61 ()", "PPMSDR\\PPMSDR Regen htr flag", "PPMSDR\\PPMSDR Sample Position (deg)", "PPMSDR\\PPMSDR Seq Stat ()", "PPMSDR\\PPMSDR Setpoint (K)", "PPMSDR\\PPMSDR Signal 1 Vin (V)", "PPMSDR\\PPMSDR Signal 2 Vin (V)", "PPMSDR\\PPMSDR Spare Excit (uA)", "PPMSDR\\PPMSDR Spare Therm (K)", "PPMSDR\\PPMSDR Status (code)", "PPMSDR\\PPMSDR Sw heater state", "PPMSDR\\PPMSDR Sys Temp ()", "PPMSDR\\PPMSDR System Pres (Torr)", "PPMSDR\\PPMSDR System Status (code)", "PPMSDR\\PPMSDR Tableless Map53 ()", "PPMSDR\\PPMSDR Tableless Map54 ()", "PPMSDR\\PPMSDR Temperature (K)", "PPMSDR\\PPMSDR Therm v", "PPMSDR\\PPMSDR Time Stamp (sec)", "PPMSDR\\PPMSDR Valve Position (deg)", "Sample Characterization\\2G Conductance", "Sample Characterization\\4G", "Sample Characterization\\4R", "Sample Characterization\\CURRENT", "Sample Characterization\\Experiment ID", "Sample Characterization\\Notes", "Sample Characterization\\OSCILLATION VOLTAGE", "Sample Characterization\\Sample Name", "Sample Characterization\\V1", "Sample Characterization\\V2", "SPM\\Laser Power", "SPM\\SPM scanner X", "SPM\\SPM scanner Y", "TEMPerHUM\\MFP : Humidity", "TEMPerHUM\\MFP : ID", "TEMPerHUM\\MFP : Location", "TEMPerHUM\\MFP : Picture URL", "TEMPerHUM\\MFP : Temperature", "TEMPerHUM\\MFP-3D : Humidity", "TEMPerHUM\\MFP-3D : ID", "TEMPerHUM\\MFP-3D : Location", "TEMPerHUM\\MFP-3D : Picture URL", "TEMPerHUM\\MFP-3D : Temperature", "TEMPerHUM\\TEST3 : Humidity", "TEMPerHUM\\TEST3 : ID", "TEMPerHUM\\TEST3 : Location", "TEMPerHUM\\TEST3 : Picture URL", "TEMPerHUM\\TEST3 : Temperature"]
  in  "Favorite B (Left)":u16[](array[ring])=[172] items=["Attocube 3DR\\axis 1: Amplitude", "Attocube 3DR\\axis 1: Capacitance", "Attocube 3DR\\axis 1: control mode", "Attocube 3DR\\axis 1: current position", "Attocube 3DR\\axis 1: DCLevel", "Attocube 3DR\\axis 1: Frequency", "Attocube 3DR\\axis 1: moving", "Attocube 3DR\\axis 1: Output", "Attocube 3DR\\axis 1: rot. count", "Attocube 3DR\\axis 1: sensor disconnected", "Attocube 3DR\\axis 1: sensor error", "Attocube 3DR\\axis 1: Single Circle Mode", "Attocube 3DR\\axis 1: sp position", "Attocube 3DR\\axis 1: sp rot count", "Attocube 3DR\\axis 1: speed", "Attocube 3DR\\axis 1: StepWidth", "Attocube 3DR\\axis 1: stop detected", "Attocube 3DR\\axis 1: stop enable", "Attocube 3DR\\axis 1: Target GND", "Attocube 3DR\\axis 2: Amplitude", "Attocube 3DR\\axis 2: Capacitance", "Attocube 3DR\\axis 2: control mode", "Attocube 3DR\\axis 2: current position", "Attocube 3DR\\axis 2: DCLevel", "Attocube 3DR\\axis 2: Frequency", "Attocube 3DR\\axis 2: moving", "Attocube 3DR\\axis 2: Output", "Attocube 3DR\\axis 2: rot. count", "Attocube 3DR\\axis 2: sensor disconnected", "Attocube 3DR\\axis 2: sensor error", "Attocube 3DR\\axis 2: Single Circle Mode", "Attocube 3DR\\axis 2: sp position", "Attocube 3DR\\axis 2: sp rot count", "Attocube 3DR\\axis 2: speed", "Attocube 3DR\\axis 2: StepWidth", "Attocube 3DR\\axis 2: stop detected", "Attocube 3DR\\axis 2: stop enable", "Attocube 3DR\\axis 2: Target GND", "Attocube 3DR\\static amplitude", "Cypher\\Cypher RH1", "Cypher\\Cypher RH2", "Cypher\\Cypher Temperature", "Cypher\\Cypher_Funnel_Property", "Cypher\\Cypher_Path_Property", "Cypher\\Cypher_Rectangle_Property", "DR200\\DR200_Magnet_Field", "DR200\\DR200_Magnet_Field_Target", "DR200\\DR200_Magnet_PS_Current", "DR200\\DR200_Magnet_PS_Field", "DR200\\DR200_Magnet_PS_Voltage", "DR200\\DR200_Magnet_Rate_Target", "DR200\\DR200_Magnet_Status_Activity", "DR200\\DR200_Magnet_Status_Mode", "DR200\\DR200_Magnet_Status_Switch_Heater", "DR200\\DR200_Magnet_Status_System", "JLevy\\Levy 1", "Leiden CF900\\CF Impedance CMN", "Leiden CF900\\CF_FP_STATE", "Leiden CF900\\CF_KH_ch1", "Leiden CF900\\CF_KH_ch2", "Leiden CF900\\CF_KH_ch3", "Leiden CF900\\CF_KH_ch4", "Leiden CF900\\CF_KH_ch5", "Leiden CF900\\CF_KH_ch6", "Leiden CF900\\CF_KH_ch7", "Leiden CF900\\CF_KH_ch8", "Leiden CF900\\CF_TC_calibration", "Leiden CF900\\CF_TC_description", "Leiden CF900\\CF_TC_Z_calibration", "Leiden CF900\\CF_TC_Z_description", "Leiden CF900\\CF_TC_Z_R0", "Leiden CF900\\CF_TC_Z_R1", "Leiden CF900\\CF_TC_Z_R2", "Leiden CF900\\CF_TC_Z_R3", "Leiden CF900\\CF_TC_Z_R4", "Leiden CF900\\CF_TC_Z_R5", "Leiden CF900\\CF_TC_Z_R6", "Leiden CF900\\CF_TC_Z_R7", "Leiden CF900\\CF_TC_Z_R8", "Leiden CF900\\CF_TC_Z_R9", "Leiden CF900\\CF_TC_Z_T0", "Leiden CF900\\CF_TC_Z_T1", "Leiden CF900\\CF_TC_Z_T2", "Leiden CF900\\CF_TC_Z_T3", "Leiden CF900\\CF_TC_Z_T4", "Leiden CF900\\CF_TC_Z_T5", "Leiden CF900\\CF_TC_Z_T6", "Leiden CF900\\CF_TC_Z_T7", "Leiden CF900\\CF_TC_Z_T8", "Leiden CF900\\CF_TC_Z_T9", "Leiden CF900\\CF900_Cstill", "Leiden CF900\\Leiden CF FP\\CF FP Flow", "Leiden CF900\\Leiden CF FP\\CF FP He", "Leiden CF900\\Leiden CF FP\\CF FP MG0", "Leiden CF900\\Leiden CF FP\\CF FP MG1", "Leiden CF900\\Leiden CF FP\\CF FP MG2", "Leiden CF900\\Leiden CF FP\\CF FP MG3", "Leiden CF900\\Leiden CF FP\\CF FP MG4", "Leiden CF900\\Leiden CF FP\\CF FP MG5", "Leiden CF900\\Leiden CF FP\\CF FP oil", "Leiden CF900\\Leiden CF FP\\CF FP P_high", "Leiden CF900\\Leiden CF FP\\CF FP P_low", "Leiden CF900\\Leiden CF FP\\CF FP P1", "Leiden CF900\\Leiden CF FP\\CF FP P2", "Leiden CF900\\Leiden CF FP\\CF FP P3", "Leiden CF900\\Leiden CF FP\\CF FP P4", "Leiden CF900\\Leiden CF FP\\CF FP P5", "Leiden CF900\\Leiden CF FP\\CF FP P6", "Leiden CF900\\Leiden CF FP\\CF FP P7", "Leiden CF900\\Leiden CF FP\\CF FP PT current", "Leiden CF900\\Leiden CF FP\\CF FP PT on", "Leiden CF900\\Leiden CF FP\\CF FP State0", "Leiden CF900\\Leiden CF FP\\CF FP State1", "Leiden CF900\\Leiden CF FP\\CF FP State2", "Leiden CF900\\Leiden CF FP\\CF FP W_in", "Leiden CF900\\Leiden CF FP\\CF FP W_out", "Leiden CF900\\Leiden CF Impedance Bridge\\CF IB TA", "Leiden CF900\\Leiden CF Impedance Bridge\\CF IB TB", "Leiden CF900\\Leiden CF Impedance Bridge\\CF IB TC", "Leiden CF900\\Leiden CF Impedance Bridge\\CF IB TD", "Leiden CF900\\Leiden CF Impedance Bridge\\CF IB TE", "Leiden CF900\\Leiden CF Magnetic Field\\CF Field X", "Leiden CF900\\Leiden CF Magnetic Field\\CF Field Y", "Leiden CF900\\Leiden CF Magnetic Field\\CF Field Z", "Leiden CF900\\Leiden CF TC\\CF TC I0", "Leiden CF900\\Leiden CF TC\\CF TC I1", "Leiden CF900\\Leiden CF TC\\CF TC I2", "Leiden CF900\\Leiden CF TC\\CF TC I3", "Leiden CF900\\Leiden CF TC\\CF TC R0", "Leiden CF900\\Leiden CF TC\\CF TC R1", "Leiden CF900\\Leiden CF TC\\CF TC R2", "Leiden CF900\\Leiden CF TC\\CF TC R3", "Leiden CF900\\Leiden CF TC\\CF TC R4", "Leiden CF900\\Leiden CF TC\\CF TC R5", "Leiden CF900\\Leiden CF TC\\CF TC R6", "Leiden CF900\\Leiden CF TC\\CF TC R7", "Leiden CF900\\Leiden CF TC\\CF TC T0", "Leiden CF900\\Leiden CF TC\\CF TC T1", "Leiden CF900\\Leiden CF TC\\CF TC T2", "Leiden CF900\\Leiden CF TC\\CF TC T3", "Leiden CF900\\Leiden CF TC\\CF TC T4", "Leiden CF900\\Leiden CF TC\\CF TC T5", "Leiden CF900\\Leiden CF TC\\CF TC T6", "Leiden CF900\\Leiden CF TC\\CF TC T7", "Leiden CF900\\RuO2_T", "Leiden CF900\\RuO2_Z", "Leiden CF900\\Vbg", "Leiden CF900\\VRM VrmSweepMode", "Leiden CF900\\VRM VrmSweepRate", "Leiden CF900\\VRM VrmSweepTime", "Leiden CF900\\VRM VrmX setpT", "Leiden CF900\\VRM VrmY setpT", "Leiden CF900\\VRM VrmZ setpT", "Leiden CF900\\VRM X at rest", "Leiden CF900\\VRM X magA", "Leiden CF900\\VRM X magT", "Leiden CF900\\VRM X meas A", "Leiden CF900\\VRM X meas V", "Leiden CF900\\VRM X outA", "Leiden CF900\\VRM X outT", "Leiden CF900\\VRM X setpT", "Leiden CF900\\VRM X Status", "Leiden CF900\\VRM X sweep", "Leiden CF900\\VRM X sweep A", "Leiden CF900\\VRM Y at rest", "Leiden CF900\\VRM Y magA", "Leiden CF900\\VRM Y magT", "Leiden CF900\\VRM Y meas A", "Leiden CF900\\VRM Y meas V", "Leiden CF900\\VRM Y outA", "Leiden CF900\\VRM Y outT", "Leiden CF900\\VRM Y setpT", "Leiden CF900\\VRM Y Status", "Leiden CF900\\VRM Y sweep", "Leiden CF900\\VRM Y sweep A", "Leiden CF900\\VRM Z at rest", "Leiden CF900\\VRM Z magA", "Leiden CF900\\VRM Z magT", "Leiden CF900\\VRM Z meas A", "Leiden CF900\\VRM Z meas V", "Leiden CF900\\VRM Z outA", "Leiden CF900\\VRM Z outT", "Leiden CF900\\VRM Z setpT", "Leiden CF900\\VRM Z Status", "Leiden CF900\\VRM Z sweep", "Leiden CF900\\VRM Z sweep A", "MFP3D\\MFP3D Hum", "MFP3D\\MFP3D Temperature", "MFP3D\\MFP3D TSP01 Hum", "MFP3D\\MFP3D TSP01 Temperature", "MFP3D\\MFP3D User", "MNK_18T\\1820_IPS_Current", "MNK_18T\\1820_IPS_Level_He", "MNK_18T\\1820_IPS_Level_N2", "MNK_18T\\1820_IPS_M1_Current", "MNK_18T\\1820_IPS_M1_Voltage", "MNK_18T\\1820_IPS_M2_Current", "MNK_18T\\1820_IPS_M2_Voltage", "MNK_18T\\1820_IPS_M3_Current", "MNK_18T\\1820_IPS_M3_Voltage", "MNK_18T\\1820_IPS_Magnet_Field", "MNK_18T\\1820_IPS_Magnet_Temperature", "MNK_18T\\1820_IPS_Magnet_Temperature_R", "MNK_18T\\1820_IPS_PS_Field", "MNK_18T\\1820_IPS_Reply", "MNK_18T\\1820_IPS_Status", "MNK_18T\\1820_IPS_Switch", "MNK_18T\\1820_IPS_Target_Field", "MNK_18T\\1820_IPS_Target_Field_Rate", "MNK_18T\\1820_IPS_Voltage", "MNK_18T\\1820_ITC_Lambda_Status", "MNK_18T\\1820_ITC_Lambda_Temperature", "MNK_18T\\1820_ITC_Lambda_Temperature_R", "MNK_18T\\1820_ITC_Needle_Valve", "MNK_18T\\1820_ITC_Pressure", "MNK_18T\\1820_ITC_Reply", "MNK_18T\\KH_ch1", "MNK_18T\\KH_ch2", "MNK_18T\\KH_ch3", "MNK_18T\\KH_ch4", "MNK_18T\\KH_ch5", "MNK_18T\\KH_ch6", "MNK_18T\\KH_ch7", "MNK_18T\\KH_ch8", "MNK_18T\\Lockin_Results", "MNK_18T\\MNK_CMN-187_T", "MNK_18T\\MNK_CMN-187_Z", "MNK_18T\\MNK_Cstill_T", "MNK_18T\\MNK_Cstill_Z", "MNK_18T\\MNK_FP_Flow", "MNK_18T\\MNK_FP_MG0", "MNK_18T\\MNK_FP_MG1", "MNK_18T\\MNK_FP_MG2", "MNK_18T\\MNK_FP_MG3", "MNK_18T\\MNK_FP_MG4", "MNK_18T\\MNK_FP_MG5", "MNK_18T\\MNK_FP_P1", "MNK_18T\\MNK_FP_P2", "MNK_18T\\MNK_FP_P3", "MNK_18T\\MNK_FP_P4", "MNK_18T\\MNK_FP_P5", "MNK_18T\\MNK_FP_P6", "MNK_18T\\MNK_FP_P7", "MNK_18T\\MNK_FP_STATE", "MNK_18T\\MNK_FP_State0", "MNK_18T\\MNK_FP_State1", "MNK_18T\\MNK_FP_State2", "MNK_18T\\MNK_TC_calibration", "MNK_18T\\MNK_TC_description", "MNK_18T\\MNK_TC_I0", "MNK_18T\\MNK_TC_I1", "MNK_18T\\MNK_TC_I2", "MNK_18T\\MNK_TC_I3", "MNK_18T\\MNK_TC_R0", "MNK_18T\\MNK_TC_R1", "MNK_18T\\MNK_TC_R2", "MNK_18T\\MNK_TC_R3", "MNK_18T\\MNK_TC_R4", "MNK_18T\\MNK_TC_R5", "MNK_18T\\MNK_TC_R6", "MNK_18T\\MNK_TC_R7", "MNK_18T\\MNK_TC_T0", "MNK_18T\\MNK_TC_T1", "MNK_18T\\MNK_TC_T2", "MNK_18T\\MNK_TC_T3", "MNK_18T\\MNK_TC_T4", "MNK_18T\\MNK_TC_T5", "MNK_18T\\MNK_TC_T6", "MNK_18T\\MNK_TC_T7", "MNK_18T\\MNK_TC_Z_calibration", "MNK_18T\\MNK_TC_Z_description", "MNK_18T\\OSC_config", "MNK_18T\\Vbg", "Montana THZ 1\\THZ 1 Dew Point", "Montana THZ 1\\THZ 1 Humidity", "Montana THZ 1\\THZ 1 Temperature", "OneNote API HTTP\\Access Token 0000000048124379", "OneNote API HTTP\\Asana Access Token 15669051163913", "PPMS 1\\PPMS 1 Magnetic Field", "PPMS 1\\PPMS 1 Temperature", "PPMS 2\\PPMS 2 Flow Rate", "PPMS 2\\PPMS 2 Helium Level", "PPMS 2\\PPMS 2 Magnetic Field", "PPMS 2\\PPMS 2 Position", "PPMS 2\\PPMS 2 Sys Pressure", "PPMS 2\\PPMS 2 Temperature", "PPMS 2\\PPMS 2 Vbg", "PPMS2\\PPMS2 Annulus Pres (Torr)", "PPMS2\\PPMS2 Annulus Vacuum (V)", "PPMS2\\PPMS2 Block Htr Cur (mA)", "PPMS2\\PPMS2 Block Htr Pwr (W)", "PPMS2\\PPMS2 BlockHeater(Ohm)", "PPMS2\\PPMS2 Bridge 1 Excitation (uA)", "PPMS2\\PPMS2 Bridge 1 Resistance (ohms)", "PPMS2\\PPMS2 Bridge 2 Excitation (uA)", "PPMS2\\PPMS2 Bridge 2 Resistance (ohms)", "PPMS2\\PPMS2 Bridge 3 Excitation (uA)", "PPMS2\\PPMS2 Bridge 3 Resistance (ohms)", "PPMS2\\PPMS2 Bridge 4 Excitation (uA)", "PPMS2\\PPMS2 Bridge 4 Resistance (ohms)", "PPMS2\\PPMS2 CIG Cernox (K)", "PPMS2\\PPMS2 CIG Excit (uA)", "PPMS2\\PPMS2 Comment", "PPMS2\\PPMS2 DAC  I  (cnts)", "PPMS2\\PPMS2 Digital Inputs (code)", "PPMS2\\PPMS2 Drive 1 Iout (mA)", "PPMS2\\PPMS2 Drive 1 Ipower (watts)", "PPMS2\\PPMS2 Drive 2 Iout (mA)", "PPMS2\\PPMS2 Drive 2 Ipower (watts)", "PPMS2\\PPMS2 EXT Flow (L min)", "PPMS2\\PPMS2 Flapper state", "PPMS2\\PPMS2 Flow Rate (l min)", "PPMS2\\PPMS2 He Level ()", "PPMS2\\PPMS2 Hi res (A) read", "PPMS2\\PPMS2 High Vacuum mode", "PPMS2\\PPMS2 Hires enable", "PPMS2\\PPMS2 Impedance (mode)", "PPMS2\\PPMS2 iso flag", "PPMS2\\PPMS2 KRPMs", "PPMS2\\PPMS2 Last 2 eng st", "PPMS2\\PPMS2 Log", "PPMS2\\PPMS2 Mag (V) read", "PPMS2\\PPMS2 Mag (V) set", "PPMS2\\PPMS2 Mag adj sc(I)set", "PPMS2\\PPMS2 Magnet (Oe)", "PPMS2\\PPMS2 Magnetic Field (Oe)", "PPMS2\\PPMS2 Map 20 ()", "PPMS2\\PPMS2 Map 21 ()", "PPMS2\\PPMS2 Map 22 ()", "PPMS2\\PPMS2 Map 23 ()", "PPMS2\\PPMS2 Map 24 ()", "PPMS2\\PPMS2 Map 25 ()", "PPMS2\\PPMS2 Map 26 ()", "PPMS2\\PPMS2 Map 27 ()", "PPMS2\\PPMS2 Map 28 ()", "PPMS2\\PPMS2 Map 29 ()", "PPMS2\\PPMS2 Map 67 ()", "PPMS2\\PPMS2 Map 68 ()", "PPMS2\\PPMS2 Map 69 ()", "PPMS2\\PPMS2 Map 89 ()", "PPMS2\\PPMS2 Map 90 ()", "PPMS2\\PPMS2 Map 91 ()", "PPMS2\\PPMS2 Map 92 ()", "PPMS2\\PPMS2 Map 93 ()", "PPMS2\\PPMS2 Neck Excit (uA)", "PPMS2\\PPMS2 Neck Htr Cur (mA)", "PPMS2\\PPMS2 Neck Htr Pwr (W)", "PPMS2\\PPMS2 Neck Therm (K)", "PPMS2\\PPMS2 NeckHeater(Ohm)", "PPMS2\\PPMS2 Plat Excit (uA)", "PPMS2\\PPMS2 Plat Therm (K)", "PPMS2\\PPMS2 Pressure ()", "PPMS2\\PPMS2 PSU Field (Oe)", "PPMS2\\PPMS2 Pump power (W)", "PPMS2\\PPMS2 Pump temp (C)", "PPMS2\\PPMS2 Redirected 55 ()", "PPMS2\\PPMS2 Redirected 56 ()", "PPMS2\\PPMS2 Redirected 57 ()", "PPMS2\\PPMS2 Redirected 58 ()", "PPMS2\\PPMS2 Redirected 59 ()", "PPMS2\\PPMS2 Redirected 61 ()", "PPMS2\\PPMS2 Regen htr flag", "PPMS2\\PPMS2 Sample Position (deg)", "PPMS2\\PPMS2 Seq Stat ()", "PPMS2\\PPMS2 Setpoint (K)", "PPMS2\\PPMS2 Signal 1 Vin (V)", "PPMS2\\PPMS2 Signal 2 Vin (V)", "PPMS2\\PPMS2 Spare Excit (uA)", "PPMS2\\PPMS2 Spare Therm (K)", "PPMS2\\PPMS2 Status (code)", "PPMS2\\PPMS2 Sw heater state", "PPMS2\\PPMS2 Sys Temp ()", "PPMS2\\PPMS2 System Pres (Torr)", "PPMS2\\PPMS2 System Status (code)", "PPMS2\\PPMS2 Tableless Map53 ()", "PPMS2\\PPMS2 Tableless Map54 ()", "PPMS2\\PPMS2 Temperature (K)", "PPMS2\\PPMS2 Therm v", "PPMS2\\PPMS2 Time Stamp (sec)", "PPMS2\\PPMS2 Valve Position (deg)", "PPMSDR\\PPMSDR Annulus Pres (Torr)", "PPMSDR\\PPMSDR Annulus Vacuum (V)", "PPMSDR\\PPMSDR Block Htr Cur (mA)", "PPMSDR\\PPMSDR Block Htr Pwr (W)", "PPMSDR\\PPMSDR BlockHeater(Ohm)", "PPMSDR\\PPMSDR Bridge 1 Excitation (uA)", "PPMSDR\\PPMSDR Bridge 1 Resistance (ohms)", "PPMSDR\\PPMSDR Bridge 2 Excitation (uA)", "PPMSDR\\PPMSDR Bridge 2 Resistance (ohms)", "PPMSDR\\PPMSDR Bridge 3 Excitation (uA)", "PPMSDR\\PPMSDR Bridge 3 Resistance (ohms)", "PPMSDR\\PPMSDR Bridge 4 Excitation (uA)", "PPMSDR\\PPMSDR Bridge 4 Resistance (ohms)", "PPMSDR\\PPMSDR CIG Cernox (K)", "PPMSDR\\PPMSDR CIG Excit (uA)", "PPMSDR\\PPMSDR Comment", "PPMSDR\\PPMSDR DAC  I  (cnts)", "PPMSDR\\PPMSDR Digital Inputs (code)", "PPMSDR\\PPMSDR Drive 1 Iout (mA)", "PPMSDR\\PPMSDR Drive 1 Ipower (watts)", "PPMSDR\\PPMSDR Drive 2 Iout (mA)", "PPMSDR\\PPMSDR Drive 2 Ipower (watts)", "PPMSDR\\PPMSDR EXT Flow (L min)", "PPMSDR\\PPMSDR Flapper state", "PPMSDR\\PPMSDR Flow Rate (l min)", "PPMSDR\\PPMSDR He Level ()", "PPMSDR\\PPMSDR Hi res (A) read", "PPMSDR\\PPMSDR High Vacuum mode", "PPMSDR\\PPMSDR Hires enable", "PPMSDR\\PPMSDR Impedance (mode)", "PPMSDR\\PPMSDR iso flag", "PPMSDR\\PPMSDR KRPMs", "PPMSDR\\PPMSDR Last 2 eng st", "PPMSDR\\PPMSDR Log", "PPMSDR\\PPMSDR low res (A) read", "PPMSDR\\PPMSDR Mag (V) read", "PPMSDR\\PPMSDR Mag (V) set", "PPMSDR\\PPMSDR Mag adj sc(I)set", "PPMSDR\\PPMSDR Magnet (Oe)", "PPMSDR\\PPMSDR Magnetic Field (Oe)", "PPMSDR\\PPMSDR MAP 1", "PPMSDR\\PPMSDR MAP 10", "PPMSDR\\PPMSDR MAP 11", "PPMSDR\\PPMSDR MAP 12", "PPMSDR\\PPMSDR MAP 13", "PPMSDR\\PPMSDR MAP 14", "PPMSDR\\PPMSDR MAP 15", "PPMSDR\\PPMSDR MAP 16", "PPMSDR\\PPMSDR MAP 17", "PPMSDR\\PPMSDR MAP 18", "PPMSDR\\PPMSDR MAP 19", "PPMSDR\\PPMSDR MAP 2", "PPMSDR\\PPMSDR MAP 20", "PPMSDR\\PPMSDR Map 20 ()", "PPMSDR\\PPMSDR MAP 21", "PPMSDR\\PPMSDR Map 21 ()", "PPMSDR\\PPMSDR MAP 22", "PPMSDR\\PPMSDR Map 22 ()", "PPMSDR\\PPMSDR MAP 23", "PPMSDR\\PPMSDR Map 23 ()", "PPMSDR\\PPMSDR MAP 24", "PPMSDR\\PPMSDR Map 24 ()", "PPMSDR\\PPMSDR MAP 25", "PPMSDR\\PPMSDR Map 25 ()", "PPMSDR\\PPMSDR MAP 26", "PPMSDR\\PPMSDR Map 26 ()", "PPMSDR\\PPMSDR MAP 27", "PPMSDR\\PPMSDR Map 27 ()", "PPMSDR\\PPMSDR MAP 28", "PPMSDR\\PPMSDR Map 28 ()", "PPMSDR\\PPMSDR MAP 29", "PPMSDR\\PPMSDR Map 29 ()", "PPMSDR\\PPMSDR MAP 3", "PPMSDR\\PPMSDR MAP 30", "PPMSDR\\PPMSDR MAP 4", "PPMSDR\\PPMSDR MAP 5", "PPMSDR\\PPMSDR MAP 6", "PPMSDR\\PPMSDR Map 67 ()", "PPMSDR\\PPMSDR Map 68 ()", "PPMSDR\\PPMSDR Map 69 ()", "PPMSDR\\PPMSDR MAP 7", "PPMSDR\\PPMSDR MAP 8", "PPMSDR\\PPMSDR Map 89 ()", "PPMSDR\\PPMSDR MAP 9", "PPMSDR\\PPMSDR Map 90 ()", "PPMSDR\\PPMSDR Map 91 ()", "PPMSDR\\PPMSDR Map 92 ()", "PPMSDR\\PPMSDR Map 93 ()", "PPMSDR\\PPMSDR Neck Excit (uA)", "PPMSDR\\PPMSDR Neck Htr Cur (mA)", "PPMSDR\\PPMSDR Neck Htr Pwr (W)", "PPMSDR\\PPMSDR Neck Therm (K)", "PPMSDR\\PPMSDR NeckHeater(Ohm)", "PPMSDR\\PPMSDR Plat Excit (uA)", "PPMSDR\\PPMSDR Plat Therm (K)", "PPMSDR\\PPMSDR Pressure ()", "PPMSDR\\PPMSDR Pump power (W)", "PPMSDR\\PPMSDR Pump temp (C)", "PPMSDR\\PPMSDR Redirected 55 ()", "PPMSDR\\PPMSDR Redirected 56 ()", "PPMSDR\\PPMSDR Redirected 57 ()", "PPMSDR\\PPMSDR Redirected 58 ()", "PPMSDR\\PPMSDR Redirected 59 ()", "PPMSDR\\PPMSDR Redirected 61 ()", "PPMSDR\\PPMSDR Regen htr flag", "PPMSDR\\PPMSDR Sample Position (deg)", "PPMSDR\\PPMSDR Seq Stat ()", "PPMSDR\\PPMSDR Setpoint (K)", "PPMSDR\\PPMSDR Signal 1 Vin (V)", "PPMSDR\\PPMSDR Signal 2 Vin (V)", "PPMSDR\\PPMSDR Spare Excit (uA)", "PPMSDR\\PPMSDR Spare Therm (K)", "PPMSDR\\PPMSDR Status (code)", "PPMSDR\\PPMSDR Sw heater state", "PPMSDR\\PPMSDR Sys Temp ()", "PPMSDR\\PPMSDR System Pres (Torr)", "PPMSDR\\PPMSDR System Status (code)", "PPMSDR\\PPMSDR Tableless Map53 ()", "PPMSDR\\PPMSDR Tableless Map54 ()", "PPMSDR\\PPMSDR Temperature (K)", "PPMSDR\\PPMSDR Therm v", "PPMSDR\\PPMSDR Time Stamp (sec)", "PPMSDR\\PPMSDR Valve Position (deg)", "Sample Characterization\\2G Conductance", "Sample Characterization\\4G", "Sample Characterization\\4R", "Sample Characterization\\CURRENT", "Sample Characterization\\Experiment ID", "Sample Characterization\\Notes", "Sample Characterization\\OSCILLATION VOLTAGE", "Sample Characterization\\Sample Name", "Sample Characterization\\V1", "Sample Characterization\\V2", "SPM\\Laser Power", "SPM\\SPM scanner X", "SPM\\SPM scanner Y", "TEMPerHUM\\MFP : Humidity", "TEMPerHUM\\MFP : ID", "TEMPerHUM\\MFP : Location", "TEMPerHUM\\MFP : Picture URL", "TEMPerHUM\\MFP : Temperature", "TEMPerHUM\\MFP-3D : Humidity", "TEMPerHUM\\MFP-3D : ID", "TEMPerHUM\\MFP-3D : Location", "TEMPerHUM\\MFP-3D : Picture URL", "TEMPerHUM\\MFP-3D : Temperature", "TEMPerHUM\\TEST3 : Humidity", "TEMPerHUM\\TEST3 : ID", "TEMPerHUM\\TEST3 : Location", "TEMPerHUM\\TEST3 : Picture URL", "TEMPerHUM\\TEST3 : Temperature"]
  in  "Favorite C (Right)":u16[](array[ring]) items=["Attocube 3DR\\axis 1: Amplitude", "Attocube 3DR\\axis 1: Capacitance", "Attocube 3DR\\axis 1: control mode", "Attocube 3DR\\axis 1: current position", "Attocube 3DR\\axis 1: DCLevel", "Attocube 3DR\\axis 1: Frequency", "Attocube 3DR\\axis 1: moving", "Attocube 3DR\\axis 1: Output", "Attocube 3DR\\axis 1: rot. count", "Attocube 3DR\\axis 1: sensor disconnected", "Attocube 3DR\\axis 1: sensor error", "Attocube 3DR\\axis 1: Single Circle Mode", "Attocube 3DR\\axis 1: sp position", "Attocube 3DR\\axis 1: sp rot count", "Attocube 3DR\\axis 1: speed", "Attocube 3DR\\axis 1: StepWidth", "Attocube 3DR\\axis 1: stop detected", "Attocube 3DR\\axis 1: stop enable", "Attocube 3DR\\axis 1: Target GND", "Attocube 3DR\\axis 2: Amplitude", "Attocube 3DR\\axis 2: Capacitance", "Attocube 3DR\\axis 2: control mode", "Attocube 3DR\\axis 2: current position", "Attocube 3DR\\axis 2: DCLevel", "Attocube 3DR\\axis 2: Frequency", "Attocube 3DR\\axis 2: moving", "Attocube 3DR\\axis 2: Output", "Attocube 3DR\\axis 2: rot. count", "Attocube 3DR\\axis 2: sensor disconnected", "Attocube 3DR\\axis 2: sensor error", "Attocube 3DR\\axis 2: Single Circle Mode", "Attocube 3DR\\axis 2: sp position", "Attocube 3DR\\axis 2: sp rot count", "Attocube 3DR\\axis 2: speed", "Attocube 3DR\\axis 2: StepWidth", "Attocube 3DR\\axis 2: stop detected", "Attocube 3DR\\axis 2: stop enable", "Attocube 3DR\\axis 2: Target GND", "Attocube 3DR\\static amplitude", "Cypher\\Cypher RH1", "Cypher\\Cypher RH2", "Cypher\\Cypher Temperature", "Cypher\\Cypher_Funnel_Property", "Cypher\\Cypher_Path_Property", "Cypher\\Cypher_Rectangle_Property", "DR200\\DR200_Magnet_Field", "DR200\\DR200_Magnet_Field_Target", "DR200\\DR200_Magnet_PS_Current", "DR200\\DR200_Magnet_PS_Field", "DR200\\DR200_Magnet_PS_Voltage", "DR200\\DR200_Magnet_Rate_Target", "DR200\\DR200_Magnet_Status_Activity", "DR200\\DR200_Magnet_Status_Mode", "DR200\\DR200_Magnet_Status_Switch_Heater", "DR200\\DR200_Magnet_Status_System", "JLevy\\Levy 1", "Leiden CF900\\CF Impedance CMN", "Leiden CF900\\CF_FP_STATE", "Leiden CF900\\CF_KH_ch1", "Leiden CF900\\CF_KH_ch2", "Leiden CF900\\CF_KH_ch3", "Leiden CF900\\CF_KH_ch4", "Leiden CF900\\CF_KH_ch5", "Leiden CF900\\CF_KH_ch6", "Leiden CF900\\CF_KH_ch7", "Leiden CF900\\CF_KH_ch8", "Leiden CF900\\CF_TC_calibration", "Leiden CF900\\CF_TC_description", "Leiden CF900\\CF_TC_Z_calibration", "Leiden CF900\\CF_TC_Z_description", "Leiden CF900\\CF_TC_Z_R0", "Leiden CF900\\CF_TC_Z_R1", "Leiden CF900\\CF_TC_Z_R2", "Leiden CF900\\CF_TC_Z_R3", "Leiden CF900\\CF_TC_Z_R4", "Leiden CF900\\CF_TC_Z_R5", "Leiden CF900\\CF_TC_Z_R6", "Leiden CF900\\CF_TC_Z_R7", "Leiden CF900\\CF_TC_Z_R8", "Leiden CF900\\CF_TC_Z_R9", "Leiden CF900\\CF_TC_Z_T0", "Leiden CF900\\CF_TC_Z_T1", "Leiden CF900\\CF_TC_Z_T2", "Leiden CF900\\CF_TC_Z_T3", "Leiden CF900\\CF_TC_Z_T4", "Leiden CF900\\CF_TC_Z_T5", "Leiden CF900\\CF_TC_Z_T6", "Leiden CF900\\CF_TC_Z_T7", "Leiden CF900\\CF_TC_Z_T8", "Leiden CF900\\CF_TC_Z_T9", "Leiden CF900\\CF900_Cstill", "Leiden CF900\\Leiden CF FP\\CF FP Flow", "Leiden CF900\\Leiden CF FP\\CF FP He", "Leiden CF900\\Leiden CF FP\\CF FP MG0", "Leiden CF900\\Leiden CF FP\\CF FP MG1", "Leiden CF900\\Leiden CF FP\\CF FP MG2", "Leiden CF900\\Leiden CF FP\\CF FP MG3", "Leiden CF900\\Leiden CF FP\\CF FP MG4", "Leiden CF900\\Leiden CF FP\\CF FP MG5", "Leiden CF900\\Leiden CF FP\\CF FP oil", "Leiden CF900\\Leiden CF FP\\CF FP P_high", "Leiden CF900\\Leiden CF FP\\CF FP P_low", "Leiden CF900\\Leiden CF FP\\CF FP P1", "Leiden CF900\\Leiden CF FP\\CF FP P2", "Leiden CF900\\Leiden CF FP\\CF FP P3", "Leiden CF900\\Leiden CF FP\\CF FP P4", "Leiden CF900\\Leiden CF FP\\CF FP P5", "Leiden CF900\\Leiden CF FP\\CF FP P6", "Leiden CF900\\Leiden CF FP\\CF FP P7", "Leiden CF900\\Leiden CF FP\\CF FP PT current", "Leiden CF900\\Leiden CF FP\\CF FP PT on", "Leiden CF900\\Leiden CF FP\\CF FP State0", "Leiden CF900\\Leiden CF FP\\CF FP State1", "Leiden CF900\\Leiden CF FP\\CF FP State2", "Leiden CF900\\Leiden CF FP\\CF FP W_in", "Leiden CF900\\Leiden CF FP\\CF FP W_out", "Leiden CF900\\Leiden CF Impedance Bridge\\CF IB TA", "Leiden CF900\\Leiden CF Impedance Bridge\\CF IB TB", "Leiden CF900\\Leiden CF Impedance Bridge\\CF IB TC", "Leiden CF900\\Leiden CF Impedance Bridge\\CF IB TD", "Leiden CF900\\Leiden CF Impedance Bridge\\CF IB TE", "Leiden CF900\\Leiden CF Magnetic Field\\CF Field X", "Leiden CF900\\Leiden CF Magnetic Field\\CF Field Y", "Leiden CF900\\Leiden CF Magnetic Field\\CF Field Z", "Leiden CF900\\Leiden CF TC\\CF TC I0", "Leiden CF900\\Leiden CF TC\\CF TC I1", "Leiden CF900\\Leiden CF TC\\CF TC I2", "Leiden CF900\\Leiden CF TC\\CF TC I3", "Leiden CF900\\Leiden CF TC\\CF TC R0", "Leiden CF900\\Leiden CF TC\\CF TC R1", "Leiden CF900\\Leiden CF TC\\CF TC R2", "Leiden CF900\\Leiden CF TC\\CF TC R3", "Leiden CF900\\Leiden CF TC\\CF TC R4", "Leiden CF900\\Leiden CF TC\\CF TC R5", "Leiden CF900\\Leiden CF TC\\CF TC R6", "Leiden CF900\\Leiden CF TC\\CF TC R7", "Leiden CF900\\Leiden CF TC\\CF TC T0", "Leiden CF900\\Leiden CF TC\\CF TC T1", "Leiden CF900\\Leiden CF TC\\CF TC T2", "Leiden CF900\\Leiden CF TC\\CF TC T3", "Leiden CF900\\Leiden CF TC\\CF TC T4", "Leiden CF900\\Leiden CF TC\\CF TC T5", "Leiden CF900\\Leiden CF TC\\CF TC T6", "Leiden CF900\\Leiden CF TC\\CF TC T7", "Leiden CF900\\RuO2_T", "Leiden CF900\\RuO2_Z", "Leiden CF900\\Vbg", "Leiden CF900\\VRM VrmSweepMode", "Leiden CF900\\VRM VrmSweepRate", "Leiden CF900\\VRM VrmSweepTime", "Leiden CF900\\VRM VrmX setpT", "Leiden CF900\\VRM VrmY setpT", "Leiden CF900\\VRM VrmZ setpT", "Leiden CF900\\VRM X at rest", "Leiden CF900\\VRM X magA", "Leiden CF900\\VRM X magT", "Leiden CF900\\VRM X meas A", "Leiden CF900\\VRM X meas V", "Leiden CF900\\VRM X outA", "Leiden CF900\\VRM X outT", "Leiden CF900\\VRM X setpT", "Leiden CF900\\VRM X Status", "Leiden CF900\\VRM X sweep", "Leiden CF900\\VRM X sweep A", "Leiden CF900\\VRM Y at rest", "Leiden CF900\\VRM Y magA", "Leiden CF900\\VRM Y magT", "Leiden CF900\\VRM Y meas A", "Leiden CF900\\VRM Y meas V", "Leiden CF900\\VRM Y outA", "Leiden CF900\\VRM Y outT", "Leiden CF900\\VRM Y setpT", "Leiden CF900\\VRM Y Status", "Leiden CF900\\VRM Y sweep", "Leiden CF900\\VRM Y sweep A", "Leiden CF900\\VRM Z at rest", "Leiden CF900\\VRM Z magA", "Leiden CF900\\VRM Z magT", "Leiden CF900\\VRM Z meas A", "Leiden CF900\\VRM Z meas V", "Leiden CF900\\VRM Z outA", "Leiden CF900\\VRM Z outT", "Leiden CF900\\VRM Z setpT", "Leiden CF900\\VRM Z Status", "Leiden CF900\\VRM Z sweep", "Leiden CF900\\VRM Z sweep A", "MFP3D\\MFP3D Hum", "MFP3D\\MFP3D Temperature", "MFP3D\\MFP3D TSP01 Hum", "MFP3D\\MFP3D TSP01 Temperature", "MFP3D\\MFP3D User", "MNK_18T\\1820_IPS_Current", "MNK_18T\\1820_IPS_Level_He", "MNK_18T\\1820_IPS_Level_N2", "MNK_18T\\1820_IPS_M1_Current", "MNK_18T\\1820_IPS_M1_Voltage", "MNK_18T\\1820_IPS_M2_Current", "MNK_18T\\1820_IPS_M2_Voltage", "MNK_18T\\1820_IPS_M3_Current", "MNK_18T\\1820_IPS_M3_Voltage", "MNK_18T\\1820_IPS_Magnet_Field", "MNK_18T\\1820_IPS_Magnet_Temperature", "MNK_18T\\1820_IPS_Magnet_Temperature_R", "MNK_18T\\1820_IPS_PS_Field", "MNK_18T\\1820_IPS_Reply", "MNK_18T\\1820_IPS_Status", "MNK_18T\\1820_IPS_Switch", "MNK_18T\\1820_IPS_Target_Field", "MNK_18T\\1820_IPS_Target_Field_Rate", "MNK_18T\\1820_IPS_Voltage", "MNK_18T\\1820_ITC_Lambda_Status", "MNK_18T\\1820_ITC_Lambda_Temperature", "MNK_18T\\1820_ITC_Lambda_Temperature_R", "MNK_18T\\1820_ITC_Needle_Valve", "MNK_18T\\1820_ITC_Pressure", "MNK_18T\\1820_ITC_Reply", "MNK_18T\\KH_ch1", "MNK_18T\\KH_ch2", "MNK_18T\\KH_ch3", "MNK_18T\\KH_ch4", "MNK_18T\\KH_ch5", "MNK_18T\\KH_ch6", "MNK_18T\\KH_ch7", "MNK_18T\\KH_ch8", "MNK_18T\\Lockin_Results", "MNK_18T\\MNK_CMN-187_T", "MNK_18T\\MNK_CMN-187_Z", "MNK_18T\\MNK_Cstill_T", "MNK_18T\\MNK_Cstill_Z", "MNK_18T\\MNK_FP_Flow", "MNK_18T\\MNK_FP_MG0", "MNK_18T\\MNK_FP_MG1", "MNK_18T\\MNK_FP_MG2", "MNK_18T\\MNK_FP_MG3", "MNK_18T\\MNK_FP_MG4", "MNK_18T\\MNK_FP_MG5", "MNK_18T\\MNK_FP_P1", "MNK_18T\\MNK_FP_P2", "MNK_18T\\MNK_FP_P3", "MNK_18T\\MNK_FP_P4", "MNK_18T\\MNK_FP_P5", "MNK_18T\\MNK_FP_P6", "MNK_18T\\MNK_FP_P7", "MNK_18T\\MNK_FP_STATE", "MNK_18T\\MNK_FP_State0", "MNK_18T\\MNK_FP_State1", "MNK_18T\\MNK_FP_State2", "MNK_18T\\MNK_TC_calibration", "MNK_18T\\MNK_TC_description", "MNK_18T\\MNK_TC_I0", "MNK_18T\\MNK_TC_I1", "MNK_18T\\MNK_TC_I2", "MNK_18T\\MNK_TC_I3", "MNK_18T\\MNK_TC_R0", "MNK_18T\\MNK_TC_R1", "MNK_18T\\MNK_TC_R2", "MNK_18T\\MNK_TC_R3", "MNK_18T\\MNK_TC_R4", "MNK_18T\\MNK_TC_R5", "MNK_18T\\MNK_TC_R6", "MNK_18T\\MNK_TC_R7", "MNK_18T\\MNK_TC_T0", "MNK_18T\\MNK_TC_T1", "MNK_18T\\MNK_TC_T2", "MNK_18T\\MNK_TC_T3", "MNK_18T\\MNK_TC_T4", "MNK_18T\\MNK_TC_T5", "MNK_18T\\MNK_TC_T6", "MNK_18T\\MNK_TC_T7", "MNK_18T\\MNK_TC_Z_calibration", "MNK_18T\\MNK_TC_Z_description", "MNK_18T\\OSC_config", "MNK_18T\\Vbg", "Montana THZ 1\\THZ 1 Dew Point", "Montana THZ 1\\THZ 1 Humidity", "Montana THZ 1\\THZ 1 Temperature", "OneNote API HTTP\\Access Token 0000000048124379", "OneNote API HTTP\\Asana Access Token 15669051163913", "PPMS 1\\PPMS 1 Magnetic Field", "PPMS 1\\PPMS 1 Temperature", "PPMS 2\\PPMS 2 Flow Rate", "PPMS 2\\PPMS 2 Helium Level", "PPMS 2\\PPMS 2 Magnetic Field", "PPMS 2\\PPMS 2 Position", "PPMS 2\\PPMS 2 Sys Pressure", "PPMS 2\\PPMS 2 Temperature", "PPMS 2\\PPMS 2 Vbg", "PPMS2\\PPMS2 Annulus Pres (Torr)", "PPMS2\\PPMS2 Annulus Vacuum (V)", "PPMS2\\PPMS2 Block Htr Cur (mA)", "PPMS2\\PPMS2 Block Htr Pwr (W)", "PPMS2\\PPMS2 BlockHeater(Ohm)", "PPMS2\\PPMS2 Bridge 1 Excitation (uA)", "PPMS2\\PPMS2 Bridge 1 Resistance (ohms)", "PPMS2\\PPMS2 Bridge 2 Excitation (uA)", "PPMS2\\PPMS2 Bridge 2 Resistance (ohms)", "PPMS2\\PPMS2 Bridge 3 Excitation (uA)", "PPMS2\\PPMS2 Bridge 3 Resistance (ohms)", "PPMS2\\PPMS2 Bridge 4 Excitation (uA)", "PPMS2\\PPMS2 Bridge 4 Resistance (ohms)", "PPMS2\\PPMS2 CIG Cernox (K)", "PPMS2\\PPMS2 CIG Excit (uA)", "PPMS2\\PPMS2 Comment", "PPMS2\\PPMS2 DAC  I  (cnts)", "PPMS2\\PPMS2 Digital Inputs (code)", "PPMS2\\PPMS2 Drive 1 Iout (mA)", "PPMS2\\PPMS2 Drive 1 Ipower (watts)", "PPMS2\\PPMS2 Drive 2 Iout (mA)", "PPMS2\\PPMS2 Drive 2 Ipower (watts)", "PPMS2\\PPMS2 EXT Flow (L min)", "PPMS2\\PPMS2 Flapper state", "PPMS2\\PPMS2 Flow Rate (l min)", "PPMS2\\PPMS2 He Level ()", "PPMS2\\PPMS2 Hi res (A) read", "PPMS2\\PPMS2 High Vacuum mode", "PPMS2\\PPMS2 Hires enable", "PPMS2\\PPMS2 Impedance (mode)", "PPMS2\\PPMS2 iso flag", "PPMS2\\PPMS2 KRPMs", "PPMS2\\PPMS2 Last 2 eng st", "PPMS2\\PPMS2 Log", "PPMS2\\PPMS2 Mag (V) read", "PPMS2\\PPMS2 Mag (V) set", "PPMS2\\PPMS2 Mag adj sc(I)set", "PPMS2\\PPMS2 Magnet (Oe)", "PPMS2\\PPMS2 Magnetic Field (Oe)", "PPMS2\\PPMS2 Map 20 ()", "PPMS2\\PPMS2 Map 21 ()", "PPMS2\\PPMS2 Map 22 ()", "PPMS2\\PPMS2 Map 23 ()", "PPMS2\\PPMS2 Map 24 ()", "PPMS2\\PPMS2 Map 25 ()", "PPMS2\\PPMS2 Map 26 ()", "PPMS2\\PPMS2 Map 27 ()", "PPMS2\\PPMS2 Map 28 ()", "PPMS2\\PPMS2 Map 29 ()", "PPMS2\\PPMS2 Map 67 ()", "PPMS2\\PPMS2 Map 68 ()", "PPMS2\\PPMS2 Map 69 ()", "PPMS2\\PPMS2 Map 89 ()", "PPMS2\\PPMS2 Map 90 ()", "PPMS2\\PPMS2 Map 91 ()", "PPMS2\\PPMS2 Map 92 ()", "PPMS2\\PPMS2 Map 93 ()", "PPMS2\\PPMS2 Neck Excit (uA)", "PPMS2\\PPMS2 Neck Htr Cur (mA)", "PPMS2\\PPMS2 Neck Htr Pwr (W)", "PPMS2\\PPMS2 Neck Therm (K)", "PPMS2\\PPMS2 NeckHeater(Ohm)", "PPMS2\\PPMS2 Plat Excit (uA)", "PPMS2\\PPMS2 Plat Therm (K)", "PPMS2\\PPMS2 Pressure ()", "PPMS2\\PPMS2 PSU Field (Oe)", "PPMS2\\PPMS2 Pump power (W)", "PPMS2\\PPMS2 Pump temp (C)", "PPMS2\\PPMS2 Redirected 55 ()", "PPMS2\\PPMS2 Redirected 56 ()", "PPMS2\\PPMS2 Redirected 57 ()", "PPMS2\\PPMS2 Redirected 58 ()", "PPMS2\\PPMS2 Redirected 59 ()", "PPMS2\\PPMS2 Redirected 61 ()", "PPMS2\\PPMS2 Regen htr flag", "PPMS2\\PPMS2 Sample Position (deg)", "PPMS2\\PPMS2 Seq Stat ()", "PPMS2\\PPMS2 Setpoint (K)", "PPMS2\\PPMS2 Signal 1 Vin (V)", "PPMS2\\PPMS2 Signal 2 Vin (V)", "PPMS2\\PPMS2 Spare Excit (uA)", "PPMS2\\PPMS2 Spare Therm (K)", "PPMS2\\PPMS2 Status (code)", "PPMS2\\PPMS2 Sw heater state", "PPMS2\\PPMS2 Sys Temp ()", "PPMS2\\PPMS2 System Pres (Torr)", "PPMS2\\PPMS2 System Status (code)", "PPMS2\\PPMS2 Tableless Map53 ()", "PPMS2\\PPMS2 Tableless Map54 ()", "PPMS2\\PPMS2 Temperature (K)", "PPMS2\\PPMS2 Therm v", "PPMS2\\PPMS2 Time Stamp (sec)", "PPMS2\\PPMS2 Valve Position (deg)", "PPMSDR\\PPMSDR Annulus Pres (Torr)", "PPMSDR\\PPMSDR Annulus Vacuum (V)", "PPMSDR\\PPMSDR Block Htr Cur (mA)", "PPMSDR\\PPMSDR Block Htr Pwr (W)", "PPMSDR\\PPMSDR BlockHeater(Ohm)", "PPMSDR\\PPMSDR Bridge 1 Excitation (uA)", "PPMSDR\\PPMSDR Bridge 1 Resistance (ohms)", "PPMSDR\\PPMSDR Bridge 2 Excitation (uA)", "PPMSDR\\PPMSDR Bridge 2 Resistance (ohms)", "PPMSDR\\PPMSDR Bridge 3 Excitation (uA)", "PPMSDR\\PPMSDR Bridge 3 Resistance (ohms)", "PPMSDR\\PPMSDR Bridge 4 Excitation (uA)", "PPMSDR\\PPMSDR Bridge 4 Resistance (ohms)", "PPMSDR\\PPMSDR CIG Cernox (K)", "PPMSDR\\PPMSDR CIG Excit (uA)", "PPMSDR\\PPMSDR Comment", "PPMSDR\\PPMSDR DAC  I  (cnts)", "PPMSDR\\PPMSDR Digital Inputs (code)", "PPMSDR\\PPMSDR Drive 1 Iout (mA)", "PPMSDR\\PPMSDR Drive 1 Ipower (watts)", "PPMSDR\\PPMSDR Drive 2 Iout (mA)", "PPMSDR\\PPMSDR Drive 2 Ipower (watts)", "PPMSDR\\PPMSDR EXT Flow (L min)", "PPMSDR\\PPMSDR Flapper state", "PPMSDR\\PPMSDR Flow Rate (l min)", "PPMSDR\\PPMSDR He Level ()", "PPMSDR\\PPMSDR Hi res (A) read", "PPMSDR\\PPMSDR High Vacuum mode", "PPMSDR\\PPMSDR Hires enable", "PPMSDR\\PPMSDR Impedance (mode)", "PPMSDR\\PPMSDR iso flag", "PPMSDR\\PPMSDR KRPMs", "PPMSDR\\PPMSDR Last 2 eng st", "PPMSDR\\PPMSDR Log", "PPMSDR\\PPMSDR low res (A) read", "PPMSDR\\PPMSDR Mag (V) read", "PPMSDR\\PPMSDR Mag (V) set", "PPMSDR\\PPMSDR Mag adj sc(I)set", "PPMSDR\\PPMSDR Magnet (Oe)", "PPMSDR\\PPMSDR Magnetic Field (Oe)", "PPMSDR\\PPMSDR MAP 1", "PPMSDR\\PPMSDR MAP 10", "PPMSDR\\PPMSDR MAP 11", "PPMSDR\\PPMSDR MAP 12", "PPMSDR\\PPMSDR MAP 13", "PPMSDR\\PPMSDR MAP 14", "PPMSDR\\PPMSDR MAP 15", "PPMSDR\\PPMSDR MAP 16", "PPMSDR\\PPMSDR MAP 17", "PPMSDR\\PPMSDR MAP 18", "PPMSDR\\PPMSDR MAP 19", "PPMSDR\\PPMSDR MAP 2", "PPMSDR\\PPMSDR MAP 20", "PPMSDR\\PPMSDR Map 20 ()", "PPMSDR\\PPMSDR MAP 21", "PPMSDR\\PPMSDR Map 21 ()", "PPMSDR\\PPMSDR MAP 22", "PPMSDR\\PPMSDR Map 22 ()", "PPMSDR\\PPMSDR MAP 23", "PPMSDR\\PPMSDR Map 23 ()", "PPMSDR\\PPMSDR MAP 24", "PPMSDR\\PPMSDR Map 24 ()", "PPMSDR\\PPMSDR MAP 25", "PPMSDR\\PPMSDR Map 25 ()", "PPMSDR\\PPMSDR MAP 26", "PPMSDR\\PPMSDR Map 26 ()", "PPMSDR\\PPMSDR MAP 27", "PPMSDR\\PPMSDR Map 27 ()", "PPMSDR\\PPMSDR MAP 28", "PPMSDR\\PPMSDR Map 28 ()", "PPMSDR\\PPMSDR MAP 29", "PPMSDR\\PPMSDR Map 29 ()", "PPMSDR\\PPMSDR MAP 3", "PPMSDR\\PPMSDR MAP 30", "PPMSDR\\PPMSDR MAP 4", "PPMSDR\\PPMSDR MAP 5", "PPMSDR\\PPMSDR MAP 6", "PPMSDR\\PPMSDR Map 67 ()", "PPMSDR\\PPMSDR Map 68 ()", "PPMSDR\\PPMSDR Map 69 ()", "PPMSDR\\PPMSDR MAP 7", "PPMSDR\\PPMSDR MAP 8", "PPMSDR\\PPMSDR Map 89 ()", "PPMSDR\\PPMSDR MAP 9", "PPMSDR\\PPMSDR Map 90 ()", "PPMSDR\\PPMSDR Map 91 ()", "PPMSDR\\PPMSDR Map 92 ()", "PPMSDR\\PPMSDR Map 93 ()", "PPMSDR\\PPMSDR Neck Excit (uA)", "PPMSDR\\PPMSDR Neck Htr Cur (mA)", "PPMSDR\\PPMSDR Neck Htr Pwr (W)", "PPMSDR\\PPMSDR Neck Therm (K)", "PPMSDR\\PPMSDR NeckHeater(Ohm)", "PPMSDR\\PPMSDR Plat Excit (uA)", "PPMSDR\\PPMSDR Plat Therm (K)", "PPMSDR\\PPMSDR Pressure ()", "PPMSDR\\PPMSDR Pump power (W)", "PPMSDR\\PPMSDR Pump temp (C)", "PPMSDR\\PPMSDR Redirected 55 ()", "PPMSDR\\PPMSDR Redirected 56 ()", "PPMSDR\\PPMSDR Redirected 57 ()", "PPMSDR\\PPMSDR Redirected 58 ()", "PPMSDR\\PPMSDR Redirected 59 ()", "PPMSDR\\PPMSDR Redirected 61 ()", "PPMSDR\\PPMSDR Regen htr flag", "PPMSDR\\PPMSDR Sample Position (deg)", "PPMSDR\\PPMSDR Seq Stat ()", "PPMSDR\\PPMSDR Setpoint (K)", "PPMSDR\\PPMSDR Signal 1 Vin (V)", "PPMSDR\\PPMSDR Signal 2 Vin (V)", "PPMSDR\\PPMSDR Spare Excit (uA)", "PPMSDR\\PPMSDR Spare Therm (K)", "PPMSDR\\PPMSDR Status (code)", "PPMSDR\\PPMSDR Sw heater state", "PPMSDR\\PPMSDR Sys Temp ()", "PPMSDR\\PPMSDR System Pres (Torr)", "PPMSDR\\PPMSDR System Status (code)", "PPMSDR\\PPMSDR Tableless Map53 ()", "PPMSDR\\PPMSDR Tableless Map54 ()", "PPMSDR\\PPMSDR Temperature (K)", "PPMSDR\\PPMSDR Therm v", "PPMSDR\\PPMSDR Time Stamp (sec)", "PPMSDR\\PPMSDR Valve Position (deg)", "Sample Characterization\\2G Conductance", "Sample Characterization\\4G", "Sample Characterization\\4R", "Sample Characterization\\CURRENT", "Sample Characterization\\Experiment ID", "Sample Characterization\\Notes", "Sample Characterization\\OSCILLATION VOLTAGE", "Sample Characterization\\Sample Name", "Sample Characterization\\V1", "Sample Characterization\\V2", "SPM\\Laser Power", "SPM\\SPM scanner X", "SPM\\SPM scanner Y", "TEMPerHUM\\MFP : Humidity", "TEMPerHUM\\MFP : ID", "TEMPerHUM\\MFP : Location", "TEMPerHUM\\MFP : Picture URL", "TEMPerHUM\\MFP : Temperature", "TEMPerHUM\\MFP-3D : Humidity", "TEMPerHUM\\MFP-3D : ID", "TEMPerHUM\\MFP-3D : Location", "TEMPerHUM\\MFP-3D : Picture URL", "TEMPerHUM\\MFP-3D : Temperature", "TEMPerHUM\\TEST3 : Humidity", "TEMPerHUM\\TEST3 : ID", "TEMPerHUM\\TEST3 : Location", "TEMPerHUM\\TEST3 : Picture URL", "TEMPerHUM\\TEST3 : Temperature"]
  in  "Favorite C (Left)":u16[](array[ring])=[84, 85, 86] items=["Attocube 3DR\\axis 1: Amplitude", "Attocube 3DR\\axis 1: Capacitance", "Attocube 3DR\\axis 1: control mode", "Attocube 3DR\\axis 1: current position", "Attocube 3DR\\axis 1: DCLevel", "Attocube 3DR\\axis 1: Frequency", "Attocube 3DR\\axis 1: moving", "Attocube 3DR\\axis 1: Output", "Attocube 3DR\\axis 1: rot. count", "Attocube 3DR\\axis 1: sensor disconnected", "Attocube 3DR\\axis 1: sensor error", "Attocube 3DR\\axis 1: Single Circle Mode", "Attocube 3DR\\axis 1: sp position", "Attocube 3DR\\axis 1: sp rot count", "Attocube 3DR\\axis 1: speed", "Attocube 3DR\\axis 1: StepWidth", "Attocube 3DR\\axis 1: stop detected", "Attocube 3DR\\axis 1: stop enable", "Attocube 3DR\\axis 1: Target GND", "Attocube 3DR\\axis 2: Amplitude", "Attocube 3DR\\axis 2: Capacitance", "Attocube 3DR\\axis 2: control mode", "Attocube 3DR\\axis 2: current position", "Attocube 3DR\\axis 2: DCLevel", "Attocube 3DR\\axis 2: Frequency", "Attocube 3DR\\axis 2: moving", "Attocube 3DR\\axis 2: Output", "Attocube 3DR\\axis 2: rot. count", "Attocube 3DR\\axis 2: sensor disconnected", "Attocube 3DR\\axis 2: sensor error", "Attocube 3DR\\axis 2: Single Circle Mode", "Attocube 3DR\\axis 2: sp position", "Attocube 3DR\\axis 2: sp rot count", "Attocube 3DR\\axis 2: speed", "Attocube 3DR\\axis 2: StepWidth", "Attocube 3DR\\axis 2: stop detected", "Attocube 3DR\\axis 2: stop enable", "Attocube 3DR\\axis 2: Target GND", "Attocube 3DR\\static amplitude", "Cypher\\Cypher RH1", "Cypher\\Cypher RH2", "Cypher\\Cypher Temperature", "Cypher\\Cypher_Funnel_Property", "Cypher\\Cypher_Path_Property", "Cypher\\Cypher_Rectangle_Property", "DR200\\DR200_Magnet_Field", "DR200\\DR200_Magnet_Field_Target", "DR200\\DR200_Magnet_PS_Current", "DR200\\DR200_Magnet_PS_Field", "DR200\\DR200_Magnet_PS_Voltage", "DR200\\DR200_Magnet_Rate_Target", "DR200\\DR200_Magnet_Status_Activity", "DR200\\DR200_Magnet_Status_Mode", "DR200\\DR200_Magnet_Status_Switch_Heater", "DR200\\DR200_Magnet_Status_System", "JLevy\\Levy 1", "Leiden CF900\\CF Impedance CMN", "Leiden CF900\\CF_FP_STATE", "Leiden CF900\\CF_KH_ch1", "Leiden CF900\\CF_KH_ch2", "Leiden CF900\\CF_KH_ch3", "Leiden CF900\\CF_KH_ch4", "Leiden CF900\\CF_KH_ch5", "Leiden CF900\\CF_KH_ch6", "Leiden CF900\\CF_KH_ch7", "Leiden CF900\\CF_KH_ch8", "Leiden CF900\\CF_TC_calibration", "Leiden CF900\\CF_TC_description", "Leiden CF900\\CF_TC_Z_calibration", "Leiden CF900\\CF_TC_Z_description", "Leiden CF900\\CF_TC_Z_R0", "Leiden CF900\\CF_TC_Z_R1", "Leiden CF900\\CF_TC_Z_R2", "Leiden CF900\\CF_TC_Z_R3", "Leiden CF900\\CF_TC_Z_R4", "Leiden CF900\\CF_TC_Z_R5", "Leiden CF900\\CF_TC_Z_R6", "Leiden CF900\\CF_TC_Z_R7", "Leiden CF900\\CF_TC_Z_R8", "Leiden CF900\\CF_TC_Z_R9", "Leiden CF900\\CF_TC_Z_T0", "Leiden CF900\\CF_TC_Z_T1", "Leiden CF900\\CF_TC_Z_T2", "Leiden CF900\\CF_TC_Z_T3", "Leiden CF900\\CF_TC_Z_T4", "Leiden CF900\\CF_TC_Z_T5", "Leiden CF900\\CF_TC_Z_T6", "Leiden CF900\\CF_TC_Z_T7", "Leiden CF900\\CF_TC_Z_T8", "Leiden CF900\\CF_TC_Z_T9", "Leiden CF900\\CF900_Cstill", "Leiden CF900\\Leiden CF FP\\CF FP Flow", "Leiden CF900\\Leiden CF FP\\CF FP He", "Leiden CF900\\Leiden CF FP\\CF FP MG0", "Leiden CF900\\Leiden CF FP\\CF FP MG1", "Leiden CF900\\Leiden CF FP\\CF FP MG2", "Leiden CF900\\Leiden CF FP\\CF FP MG3", "Leiden CF900\\Leiden CF FP\\CF FP MG4", "Leiden CF900\\Leiden CF FP\\CF FP MG5", "Leiden CF900\\Leiden CF FP\\CF FP oil", "Leiden CF900\\Leiden CF FP\\CF FP P_high", "Leiden CF900\\Leiden CF FP\\CF FP P_low", "Leiden CF900\\Leiden CF FP\\CF FP P1", "Leiden CF900\\Leiden CF FP\\CF FP P2", "Leiden CF900\\Leiden CF FP\\CF FP P3", "Leiden CF900\\Leiden CF FP\\CF FP P4", "Leiden CF900\\Leiden CF FP\\CF FP P5", "Leiden CF900\\Leiden CF FP\\CF FP P6", "Leiden CF900\\Leiden CF FP\\CF FP P7", "Leiden CF900\\Leiden CF FP\\CF FP PT current", "Leiden CF900\\Leiden CF FP\\CF FP PT on", "Leiden CF900\\Leiden CF FP\\CF FP State0", "Leiden CF900\\Leiden CF FP\\CF FP State1", "Leiden CF900\\Leiden CF FP\\CF FP State2", "Leiden CF900\\Leiden CF FP\\CF FP W_in", "Leiden CF900\\Leiden CF FP\\CF FP W_out", "Leiden CF900\\Leiden CF Impedance Bridge\\CF IB TA", "Leiden CF900\\Leiden CF Impedance Bridge\\CF IB TB", "Leiden CF900\\Leiden CF Impedance Bridge\\CF IB TC", "Leiden CF900\\Leiden CF Impedance Bridge\\CF IB TD", "Leiden CF900\\Leiden CF Impedance Bridge\\CF IB TE", "Leiden CF900\\Leiden CF Magnetic Field\\CF Field X", "Leiden CF900\\Leiden CF Magnetic Field\\CF Field Y", "Leiden CF900\\Leiden CF Magnetic Field\\CF Field Z", "Leiden CF900\\Leiden CF TC\\CF TC I0", "Leiden CF900\\Leiden CF TC\\CF TC I1", "Leiden CF900\\Leiden CF TC\\CF TC I2", "Leiden CF900\\Leiden CF TC\\CF TC I3", "Leiden CF900\\Leiden CF TC\\CF TC R0", "Leiden CF900\\Leiden CF TC\\CF TC R1", "Leiden CF900\\Leiden CF TC\\CF TC R2", "Leiden CF900\\Leiden CF TC\\CF TC R3", "Leiden CF900\\Leiden CF TC\\CF TC R4", "Leiden CF900\\Leiden CF TC\\CF TC R5", "Leiden CF900\\Leiden CF TC\\CF TC R6", "Leiden CF900\\Leiden CF TC\\CF TC R7", "Leiden CF900\\Leiden CF TC\\CF TC T0", "Leiden CF900\\Leiden CF TC\\CF TC T1", "Leiden CF900\\Leiden CF TC\\CF TC T2", "Leiden CF900\\Leiden CF TC\\CF TC T3", "Leiden CF900\\Leiden CF TC\\CF TC T4", "Leiden CF900\\Leiden CF TC\\CF TC T5", "Leiden CF900\\Leiden CF TC\\CF TC T6", "Leiden CF900\\Leiden CF TC\\CF TC T7", "Leiden CF900\\RuO2_T", "Leiden CF900\\RuO2_Z", "Leiden CF900\\Vbg", "Leiden CF900\\VRM VrmSweepMode", "Leiden CF900\\VRM VrmSweepRate", "Leiden CF900\\VRM VrmSweepTime", "Leiden CF900\\VRM VrmX setpT", "Leiden CF900\\VRM VrmY setpT", "Leiden CF900\\VRM VrmZ setpT", "Leiden CF900\\VRM X at rest", "Leiden CF900\\VRM X magA", "Leiden CF900\\VRM X magT", "Leiden CF900\\VRM X meas A", "Leiden CF900\\VRM X meas V", "Leiden CF900\\VRM X outA", "Leiden CF900\\VRM X outT", "Leiden CF900\\VRM X setpT", "Leiden CF900\\VRM X Status", "Leiden CF900\\VRM X sweep", "Leiden CF900\\VRM X sweep A", "Leiden CF900\\VRM Y at rest", "Leiden CF900\\VRM Y magA", "Leiden CF900\\VRM Y magT", "Leiden CF900\\VRM Y meas A", "Leiden CF900\\VRM Y meas V", "Leiden CF900\\VRM Y outA", "Leiden CF900\\VRM Y outT", "Leiden CF900\\VRM Y setpT", "Leiden CF900\\VRM Y Status", "Leiden CF900\\VRM Y sweep", "Leiden CF900\\VRM Y sweep A", "Leiden CF900\\VRM Z at rest", "Leiden CF900\\VRM Z magA", "Leiden CF900\\VRM Z magT", "Leiden CF900\\VRM Z meas A", "Leiden CF900\\VRM Z meas V", "Leiden CF900\\VRM Z outA", "Leiden CF900\\VRM Z outT", "Leiden CF900\\VRM Z setpT", "Leiden CF900\\VRM Z Status", "Leiden CF900\\VRM Z sweep", "Leiden CF900\\VRM Z sweep A", "MFP3D\\MFP3D Hum", "MFP3D\\MFP3D Temperature", "MFP3D\\MFP3D TSP01 Hum", "MFP3D\\MFP3D TSP01 Temperature", "MFP3D\\MFP3D User", "MNK_18T\\1820_IPS_Current", "MNK_18T\\1820_IPS_Level_He", "MNK_18T\\1820_IPS_Level_N2", "MNK_18T\\1820_IPS_M1_Current", "MNK_18T\\1820_IPS_M1_Voltage", "MNK_18T\\1820_IPS_M2_Current", "MNK_18T\\1820_IPS_M2_Voltage", "MNK_18T\\1820_IPS_M3_Current", "MNK_18T\\1820_IPS_M3_Voltage", "MNK_18T\\1820_IPS_Magnet_Field", "MNK_18T\\1820_IPS_Magnet_Temperature", "MNK_18T\\1820_IPS_Magnet_Temperature_R", "MNK_18T\\1820_IPS_PS_Field", "MNK_18T\\1820_IPS_Reply", "MNK_18T\\1820_IPS_Status", "MNK_18T\\1820_IPS_Switch", "MNK_18T\\1820_IPS_Target_Field", "MNK_18T\\1820_IPS_Target_Field_Rate", "MNK_18T\\1820_IPS_Voltage", "MNK_18T\\1820_ITC_Lambda_Status", "MNK_18T\\1820_ITC_Lambda_Temperature", "MNK_18T\\1820_ITC_Lambda_Temperature_R", "MNK_18T\\1820_ITC_Needle_Valve", "MNK_18T\\1820_ITC_Pressure", "MNK_18T\\1820_ITC_Reply", "MNK_18T\\KH_ch1", "MNK_18T\\KH_ch2", "MNK_18T\\KH_ch3", "MNK_18T\\KH_ch4", "MNK_18T\\KH_ch5", "MNK_18T\\KH_ch6", "MNK_18T\\KH_ch7", "MNK_18T\\KH_ch8", "MNK_18T\\Lockin_Results", "MNK_18T\\MNK_CMN-187_T", "MNK_18T\\MNK_CMN-187_Z", "MNK_18T\\MNK_Cstill_T", "MNK_18T\\MNK_Cstill_Z", "MNK_18T\\MNK_FP_Flow", "MNK_18T\\MNK_FP_MG0", "MNK_18T\\MNK_FP_MG1", "MNK_18T\\MNK_FP_MG2", "MNK_18T\\MNK_FP_MG3", "MNK_18T\\MNK_FP_MG4", "MNK_18T\\MNK_FP_MG5", "MNK_18T\\MNK_FP_P1", "MNK_18T\\MNK_FP_P2", "MNK_18T\\MNK_FP_P3", "MNK_18T\\MNK_FP_P4", "MNK_18T\\MNK_FP_P5", "MNK_18T\\MNK_FP_P6", "MNK_18T\\MNK_FP_P7", "MNK_18T\\MNK_FP_STATE", "MNK_18T\\MNK_FP_State0", "MNK_18T\\MNK_FP_State1", "MNK_18T\\MNK_FP_State2", "MNK_18T\\MNK_TC_calibration", "MNK_18T\\MNK_TC_description", "MNK_18T\\MNK_TC_I0", "MNK_18T\\MNK_TC_I1", "MNK_18T\\MNK_TC_I2", "MNK_18T\\MNK_TC_I3", "MNK_18T\\MNK_TC_R0", "MNK_18T\\MNK_TC_R1", "MNK_18T\\MNK_TC_R2", "MNK_18T\\MNK_TC_R3", "MNK_18T\\MNK_TC_R4", "MNK_18T\\MNK_TC_R5", "MNK_18T\\MNK_TC_R6", "MNK_18T\\MNK_TC_R7", "MNK_18T\\MNK_TC_T0", "MNK_18T\\MNK_TC_T1", "MNK_18T\\MNK_TC_T2", "MNK_18T\\MNK_TC_T3", "MNK_18T\\MNK_TC_T4", "MNK_18T\\MNK_TC_T5", "MNK_18T\\MNK_TC_T6", "MNK_18T\\MNK_TC_T7", "MNK_18T\\MNK_TC_Z_calibration", "MNK_18T\\MNK_TC_Z_description", "MNK_18T\\OSC_config", "MNK_18T\\Vbg", "Montana THZ 1\\THZ 1 Dew Point", "Montana THZ 1\\THZ 1 Humidity", "Montana THZ 1\\THZ 1 Temperature", "OneNote API HTTP\\Access Token 0000000048124379", "OneNote API HTTP\\Asana Access Token 15669051163913", "PPMS 1\\PPMS 1 Magnetic Field", "PPMS 1\\PPMS 1 Temperature", "PPMS 2\\PPMS 2 Flow Rate", "PPMS 2\\PPMS 2 Helium Level", "PPMS 2\\PPMS 2 Magnetic Field", "PPMS 2\\PPMS 2 Position", "PPMS 2\\PPMS 2 Sys Pressure", "PPMS 2\\PPMS 2 Temperature", "PPMS 2\\PPMS 2 Vbg", "PPMS2\\PPMS2 Annulus Pres (Torr)", "PPMS2\\PPMS2 Annulus Vacuum (V)", "PPMS2\\PPMS2 Block Htr Cur (mA)", "PPMS2\\PPMS2 Block Htr Pwr (W)", "PPMS2\\PPMS2 BlockHeater(Ohm)", "PPMS2\\PPMS2 Bridge 1 Excitation (uA)", "PPMS2\\PPMS2 Bridge 1 Resistance (ohms)", "PPMS2\\PPMS2 Bridge 2 Excitation (uA)", "PPMS2\\PPMS2 Bridge 2 Resistance (ohms)", "PPMS2\\PPMS2 Bridge 3 Excitation (uA)", "PPMS2\\PPMS2 Bridge 3 Resistance (ohms)", "PPMS2\\PPMS2 Bridge 4 Excitation (uA)", "PPMS2\\PPMS2 Bridge 4 Resistance (ohms)", "PPMS2\\PPMS2 CIG Cernox (K)", "PPMS2\\PPMS2 CIG Excit (uA)", "PPMS2\\PPMS2 Comment", "PPMS2\\PPMS2 DAC  I  (cnts)", "PPMS2\\PPMS2 Digital Inputs (code)", "PPMS2\\PPMS2 Drive 1 Iout (mA)", "PPMS2\\PPMS2 Drive 1 Ipower (watts)", "PPMS2\\PPMS2 Drive 2 Iout (mA)", "PPMS2\\PPMS2 Drive 2 Ipower (watts)", "PPMS2\\PPMS2 EXT Flow (L min)", "PPMS2\\PPMS2 Flapper state", "PPMS2\\PPMS2 Flow Rate (l min)", "PPMS2\\PPMS2 He Level ()", "PPMS2\\PPMS2 Hi res (A) read", "PPMS2\\PPMS2 High Vacuum mode", "PPMS2\\PPMS2 Hires enable", "PPMS2\\PPMS2 Impedance (mode)", "PPMS2\\PPMS2 iso flag", "PPMS2\\PPMS2 KRPMs", "PPMS2\\PPMS2 Last 2 eng st", "PPMS2\\PPMS2 Log", "PPMS2\\PPMS2 Mag (V) read", "PPMS2\\PPMS2 Mag (V) set", "PPMS2\\PPMS2 Mag adj sc(I)set", "PPMS2\\PPMS2 Magnet (Oe)", "PPMS2\\PPMS2 Magnetic Field (Oe)", "PPMS2\\PPMS2 Map 20 ()", "PPMS2\\PPMS2 Map 21 ()", "PPMS2\\PPMS2 Map 22 ()", "PPMS2\\PPMS2 Map 23 ()", "PPMS2\\PPMS2 Map 24 ()", "PPMS2\\PPMS2 Map 25 ()", "PPMS2\\PPMS2 Map 26 ()", "PPMS2\\PPMS2 Map 27 ()", "PPMS2\\PPMS2 Map 28 ()", "PPMS2\\PPMS2 Map 29 ()", "PPMS2\\PPMS2 Map 67 ()", "PPMS2\\PPMS2 Map 68 ()", "PPMS2\\PPMS2 Map 69 ()", "PPMS2\\PPMS2 Map 89 ()", "PPMS2\\PPMS2 Map 90 ()", "PPMS2\\PPMS2 Map 91 ()", "PPMS2\\PPMS2 Map 92 ()", "PPMS2\\PPMS2 Map 93 ()", "PPMS2\\PPMS2 Neck Excit (uA)", "PPMS2\\PPMS2 Neck Htr Cur (mA)", "PPMS2\\PPMS2 Neck Htr Pwr (W)", "PPMS2\\PPMS2 Neck Therm (K)", "PPMS2\\PPMS2 NeckHeater(Ohm)", "PPMS2\\PPMS2 Plat Excit (uA)", "PPMS2\\PPMS2 Plat Therm (K)", "PPMS2\\PPMS2 Pressure ()", "PPMS2\\PPMS2 PSU Field (Oe)", "PPMS2\\PPMS2 Pump power (W)", "PPMS2\\PPMS2 Pump temp (C)", "PPMS2\\PPMS2 Redirected 55 ()", "PPMS2\\PPMS2 Redirected 56 ()", "PPMS2\\PPMS2 Redirected 57 ()", "PPMS2\\PPMS2 Redirected 58 ()", "PPMS2\\PPMS2 Redirected 59 ()", "PPMS2\\PPMS2 Redirected 61 ()", "PPMS2\\PPMS2 Regen htr flag", "PPMS2\\PPMS2 Sample Position (deg)", "PPMS2\\PPMS2 Seq Stat ()", "PPMS2\\PPMS2 Setpoint (K)", "PPMS2\\PPMS2 Signal 1 Vin (V)", "PPMS2\\PPMS2 Signal 2 Vin (V)", "PPMS2\\PPMS2 Spare Excit (uA)", "PPMS2\\PPMS2 Spare Therm (K)", "PPMS2\\PPMS2 Status (code)", "PPMS2\\PPMS2 Sw heater state", "PPMS2\\PPMS2 Sys Temp ()", "PPMS2\\PPMS2 System Pres (Torr)", "PPMS2\\PPMS2 System Status (code)", "PPMS2\\PPMS2 Tableless Map53 ()", "PPMS2\\PPMS2 Tableless Map54 ()", "PPMS2\\PPMS2 Temperature (K)", "PPMS2\\PPMS2 Therm v", "PPMS2\\PPMS2 Time Stamp (sec)", "PPMS2\\PPMS2 Valve Position (deg)", "PPMSDR\\PPMSDR Annulus Pres (Torr)", "PPMSDR\\PPMSDR Annulus Vacuum (V)", "PPMSDR\\PPMSDR Block Htr Cur (mA)", "PPMSDR\\PPMSDR Block Htr Pwr (W)", "PPMSDR\\PPMSDR BlockHeater(Ohm)", "PPMSDR\\PPMSDR Bridge 1 Excitation (uA)", "PPMSDR\\PPMSDR Bridge 1 Resistance (ohms)", "PPMSDR\\PPMSDR Bridge 2 Excitation (uA)", "PPMSDR\\PPMSDR Bridge 2 Resistance (ohms)", "PPMSDR\\PPMSDR Bridge 3 Excitation (uA)", "PPMSDR\\PPMSDR Bridge 3 Resistance (ohms)", "PPMSDR\\PPMSDR Bridge 4 Excitation (uA)", "PPMSDR\\PPMSDR Bridge 4 Resistance (ohms)", "PPMSDR\\PPMSDR CIG Cernox (K)", "PPMSDR\\PPMSDR CIG Excit (uA)", "PPMSDR\\PPMSDR Comment", "PPMSDR\\PPMSDR DAC  I  (cnts)", "PPMSDR\\PPMSDR Digital Inputs (code)", "PPMSDR\\PPMSDR Drive 1 Iout (mA)", "PPMSDR\\PPMSDR Drive 1 Ipower (watts)", "PPMSDR\\PPMSDR Drive 2 Iout (mA)", "PPMSDR\\PPMSDR Drive 2 Ipower (watts)", "PPMSDR\\PPMSDR EXT Flow (L min)", "PPMSDR\\PPMSDR Flapper state", "PPMSDR\\PPMSDR Flow Rate (l min)", "PPMSDR\\PPMSDR He Level ()", "PPMSDR\\PPMSDR Hi res (A) read", "PPMSDR\\PPMSDR High Vacuum mode", "PPMSDR\\PPMSDR Hires enable", "PPMSDR\\PPMSDR Impedance (mode)", "PPMSDR\\PPMSDR iso flag", "PPMSDR\\PPMSDR KRPMs", "PPMSDR\\PPMSDR Last 2 eng st", "PPMSDR\\PPMSDR Log", "PPMSDR\\PPMSDR low res (A) read", "PPMSDR\\PPMSDR Mag (V) read", "PPMSDR\\PPMSDR Mag (V) set", "PPMSDR\\PPMSDR Mag adj sc(I)set", "PPMSDR\\PPMSDR Magnet (Oe)", "PPMSDR\\PPMSDR Magnetic Field (Oe)", "PPMSDR\\PPMSDR MAP 1", "PPMSDR\\PPMSDR MAP 10", "PPMSDR\\PPMSDR MAP 11", "PPMSDR\\PPMSDR MAP 12", "PPMSDR\\PPMSDR MAP 13", "PPMSDR\\PPMSDR MAP 14", "PPMSDR\\PPMSDR MAP 15", "PPMSDR\\PPMSDR MAP 16", "PPMSDR\\PPMSDR MAP 17", "PPMSDR\\PPMSDR MAP 18", "PPMSDR\\PPMSDR MAP 19", "PPMSDR\\PPMSDR MAP 2", "PPMSDR\\PPMSDR MAP 20", "PPMSDR\\PPMSDR Map 20 ()", "PPMSDR\\PPMSDR MAP 21", "PPMSDR\\PPMSDR Map 21 ()", "PPMSDR\\PPMSDR MAP 22", "PPMSDR\\PPMSDR Map 22 ()", "PPMSDR\\PPMSDR MAP 23", "PPMSDR\\PPMSDR Map 23 ()", "PPMSDR\\PPMSDR MAP 24", "PPMSDR\\PPMSDR Map 24 ()", "PPMSDR\\PPMSDR MAP 25", "PPMSDR\\PPMSDR Map 25 ()", "PPMSDR\\PPMSDR MAP 26", "PPMSDR\\PPMSDR Map 26 ()", "PPMSDR\\PPMSDR MAP 27", "PPMSDR\\PPMSDR Map 27 ()", "PPMSDR\\PPMSDR MAP 28", "PPMSDR\\PPMSDR Map 28 ()", "PPMSDR\\PPMSDR MAP 29", "PPMSDR\\PPMSDR Map 29 ()", "PPMSDR\\PPMSDR MAP 3", "PPMSDR\\PPMSDR MAP 30", "PPMSDR\\PPMSDR MAP 4", "PPMSDR\\PPMSDR MAP 5", "PPMSDR\\PPMSDR MAP 6", "PPMSDR\\PPMSDR Map 67 ()", "PPMSDR\\PPMSDR Map 68 ()", "PPMSDR\\PPMSDR Map 69 ()", "PPMSDR\\PPMSDR MAP 7", "PPMSDR\\PPMSDR MAP 8", "PPMSDR\\PPMSDR Map 89 ()", "PPMSDR\\PPMSDR MAP 9", "PPMSDR\\PPMSDR Map 90 ()", "PPMSDR\\PPMSDR Map 91 ()", "PPMSDR\\PPMSDR Map 92 ()", "PPMSDR\\PPMSDR Map 93 ()", "PPMSDR\\PPMSDR Neck Excit (uA)", "PPMSDR\\PPMSDR Neck Htr Cur (mA)", "PPMSDR\\PPMSDR Neck Htr Pwr (W)", "PPMSDR\\PPMSDR Neck Therm (K)", "PPMSDR\\PPMSDR NeckHeater(Ohm)", "PPMSDR\\PPMSDR Plat Excit (uA)", "PPMSDR\\PPMSDR Plat Therm (K)", "PPMSDR\\PPMSDR Pressure ()", "PPMSDR\\PPMSDR Pump power (W)", "PPMSDR\\PPMSDR Pump temp (C)", "PPMSDR\\PPMSDR Redirected 55 ()", "PPMSDR\\PPMSDR Redirected 56 ()", "PPMSDR\\PPMSDR Redirected 57 ()", "PPMSDR\\PPMSDR Redirected 58 ()", "PPMSDR\\PPMSDR Redirected 59 ()", "PPMSDR\\PPMSDR Redirected 61 ()", "PPMSDR\\PPMSDR Regen htr flag", "PPMSDR\\PPMSDR Sample Position (deg)", "PPMSDR\\PPMSDR Seq Stat ()", "PPMSDR\\PPMSDR Setpoint (K)", "PPMSDR\\PPMSDR Signal 1 Vin (V)", "PPMSDR\\PPMSDR Signal 2 Vin (V)", "PPMSDR\\PPMSDR Spare Excit (uA)", "PPMSDR\\PPMSDR Spare Therm (K)", "PPMSDR\\PPMSDR Status (code)", "PPMSDR\\PPMSDR Sw heater state", "PPMSDR\\PPMSDR Sys Temp ()", "PPMSDR\\PPMSDR System Pres (Torr)", "PPMSDR\\PPMSDR System Status (code)", "PPMSDR\\PPMSDR Tableless Map53 ()", "PPMSDR\\PPMSDR Tableless Map54 ()", "PPMSDR\\PPMSDR Temperature (K)", "PPMSDR\\PPMSDR Therm v", "PPMSDR\\PPMSDR Time Stamp (sec)", "PPMSDR\\PPMSDR Valve Position (deg)", "Sample Characterization\\2G Conductance", "Sample Characterization\\4G", "Sample Characterization\\4R", "Sample Characterization\\CURRENT", "Sample Characterization\\Experiment ID", "Sample Characterization\\Notes", "Sample Characterization\\OSCILLATION VOLTAGE", "Sample Characterization\\Sample Name", "Sample Characterization\\V1", "Sample Characterization\\V2", "SPM\\Laser Power", "SPM\\SPM scanner X", "SPM\\SPM scanner Y", "TEMPerHUM\\MFP : Humidity", "TEMPerHUM\\MFP : ID", "TEMPerHUM\\MFP : Location", "TEMPerHUM\\MFP : Picture URL", "TEMPerHUM\\MFP : Temperature", "TEMPerHUM\\MFP-3D : Humidity", "TEMPerHUM\\MFP-3D : ID", "TEMPerHUM\\MFP-3D : Location", "TEMPerHUM\\MFP-3D : Picture URL", "TEMPerHUM\\MFP-3D : Temperature", "TEMPerHUM\\TEST3 : Humidity", "TEMPerHUM\\TEST3 : ID", "TEMPerHUM\\TEST3 : Location", "TEMPerHUM\\TEST3 : Picture URL", "TEMPerHUM\\TEST3 : Temperature"]
  in  "Stop Button":bool
  in  "Start":timestamp=timestamp(3589808455.703924 s since 1904-01-01) format="%<%X\n%x>T"
  in  "End":timestamp=timestamp(3589812055.703924 s since 1904-01-01) format="%<%X\n%x>T"
  in  "Seek Back Button":bool=TRUE
  in  "Seek Forward Button":bool
  in  "Step Size":dbl=86400.0 caption="Step Size for \"<\" and \">\"" step=3600.0 format="%<%H:%M:%S>t"
  out "Trace Names":string[](array[string])=["1820_IPS_M1_Current", "1820_IPS_Level_He"]
  in  "List of Alarms":i32(listbox)
  # "Export"
  # "Levy Lab Database Viewer ver 2017.10.03\n\n- key stroke \"Left\" = \"Ctrl\" + \"Left\", \"Right\" = \"Ctrl\" + \"Right\" \nsince left and right arror key are often used and using them for \nevent will intertere with cursor movement. \n\n- drag cursor will update the start and end"
  # "Plot the 1st vs the 2nd variable of the entire array."
  # "- load favorite A by Ctrl + A"
  # "- load favorite B by Ctrl + B"
  # "- load favorite C by Ctrl + C"
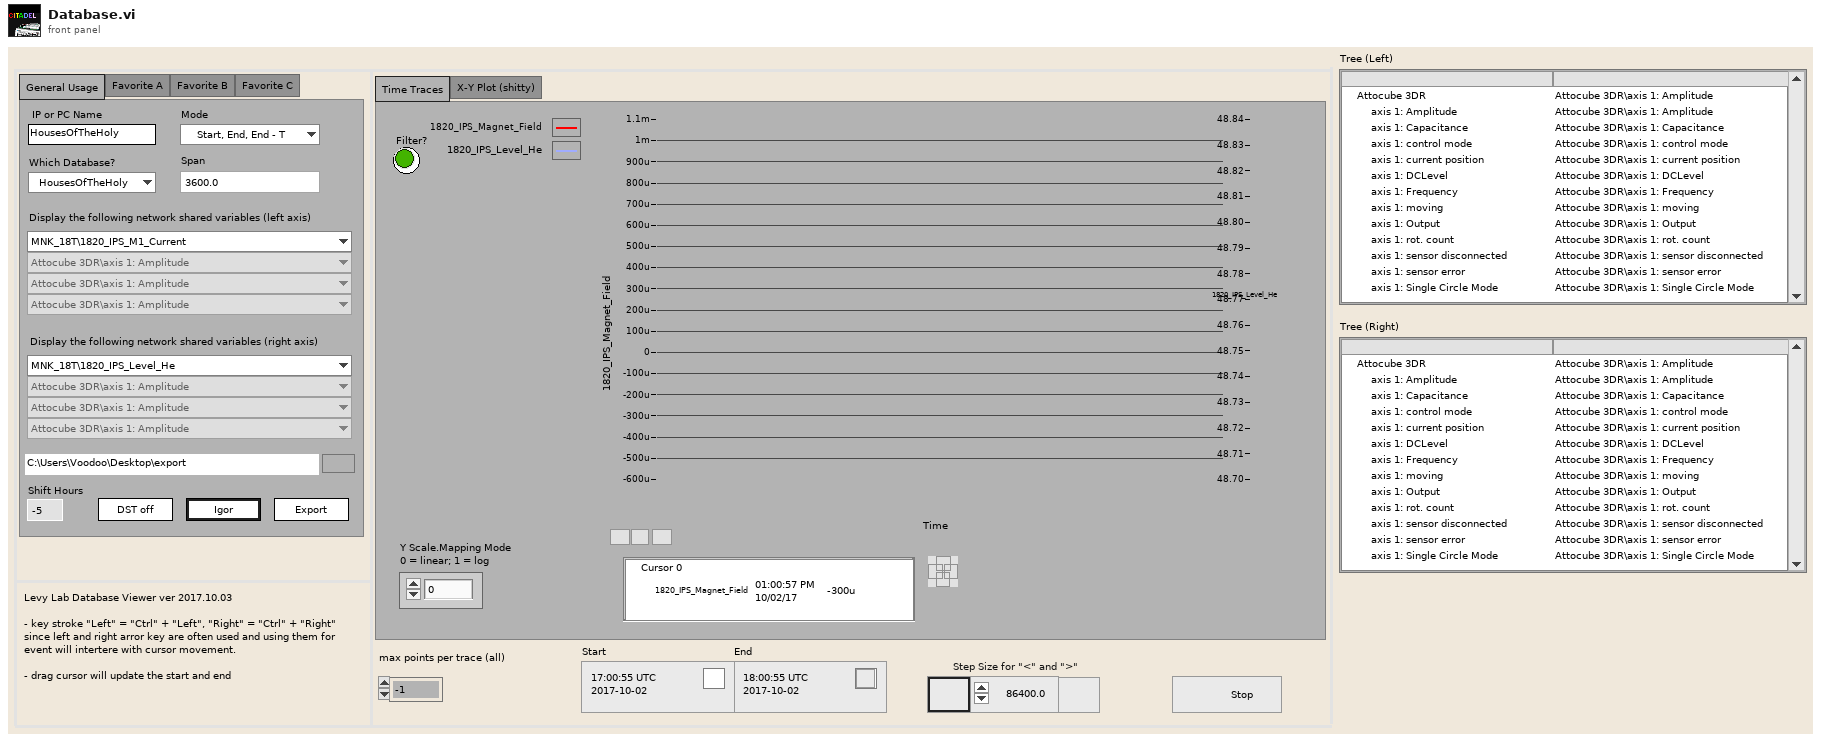
[diagram p1: front panel]
types:
  T1 = cluster{"timestamps":timestamp[], "data":dbl[]}[]
  T2 = enum32{"General Usage", "Favorite A", "Favorite B", "Favorite C"}
  T3 = enum16{"Start, End, Start + T", "Start, End, End - T", "Start, Now (Live)"}
  T4 = cluster{"start timestamp":timestamp, "stop timestamp (now)":timestamp}
  T5 = typedef "LVRangeTypeDef.ctl" = cluster{"Minimum":dbl, "Maximum":dbl, "Increment":dbl, "Minor Increment":dbl, "Start":dbl}
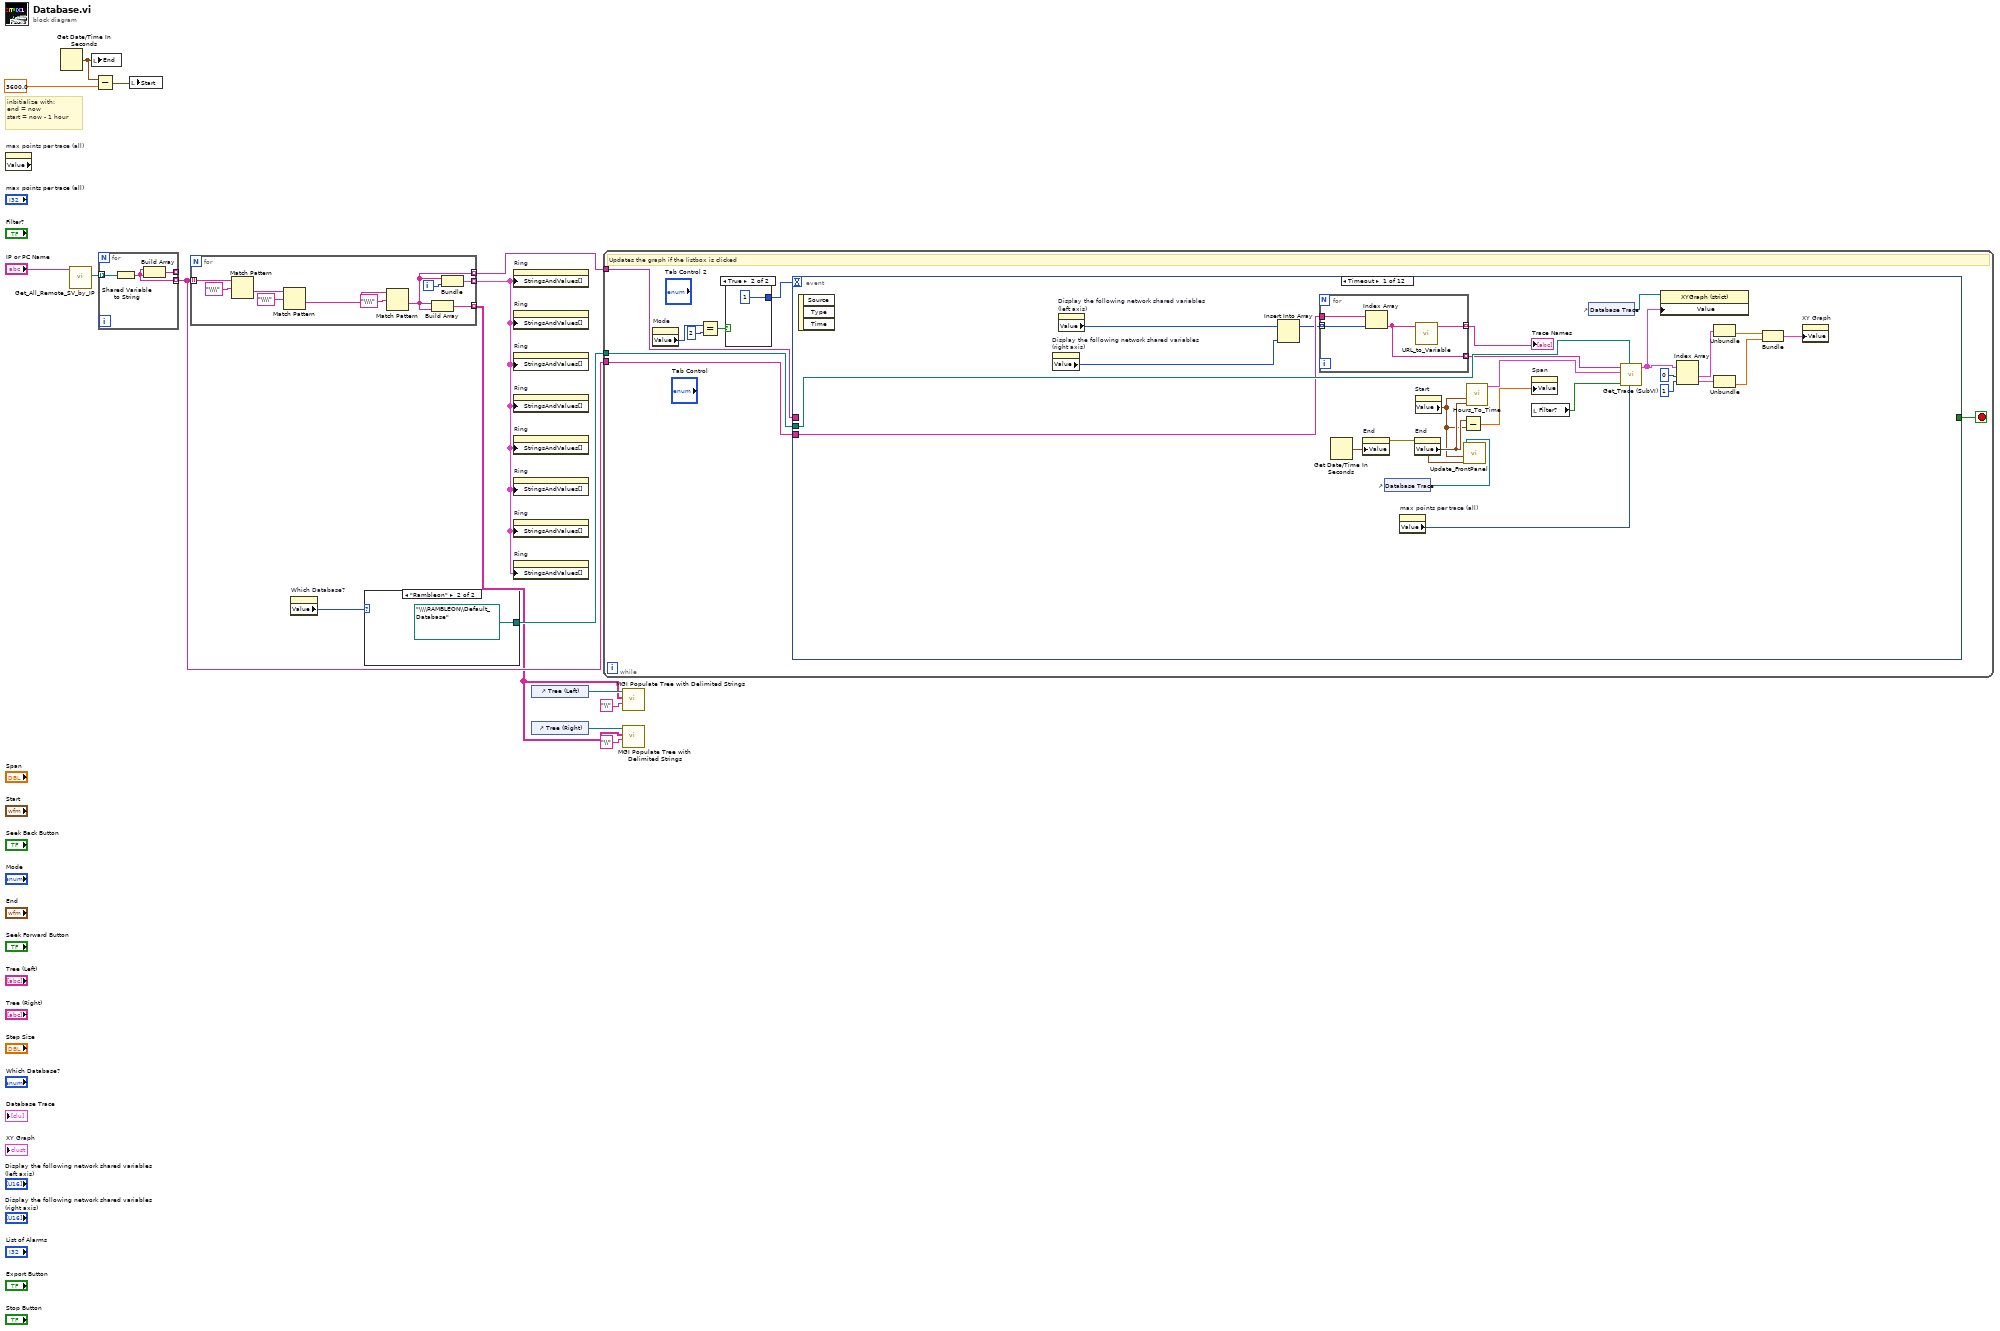
[diagram p0: block diagram]
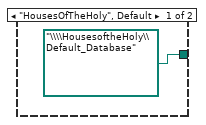
[diagram p2: hidden frame]
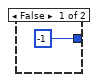
[diagram p3: hidden frame]
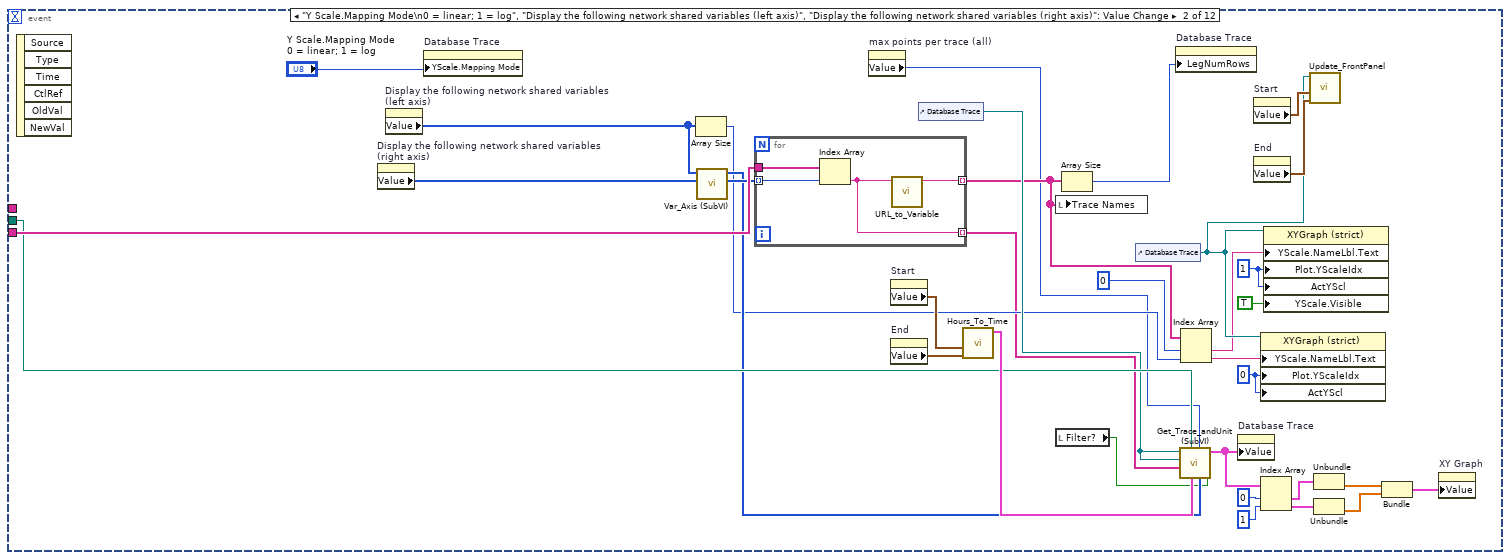
[diagram p4: hidden frame]
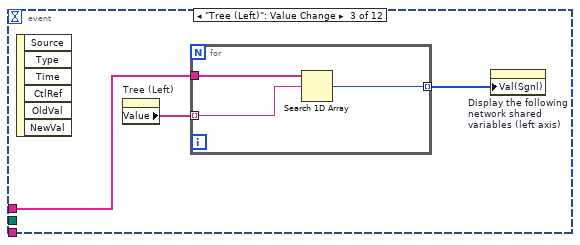
[diagram p5: hidden frame]
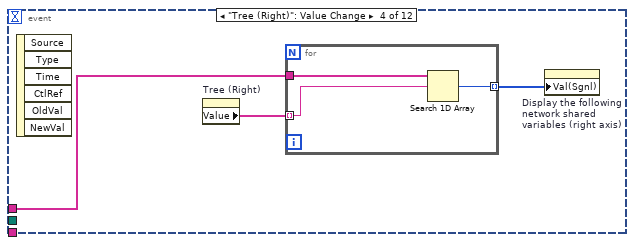
[diagram p6: hidden frame]
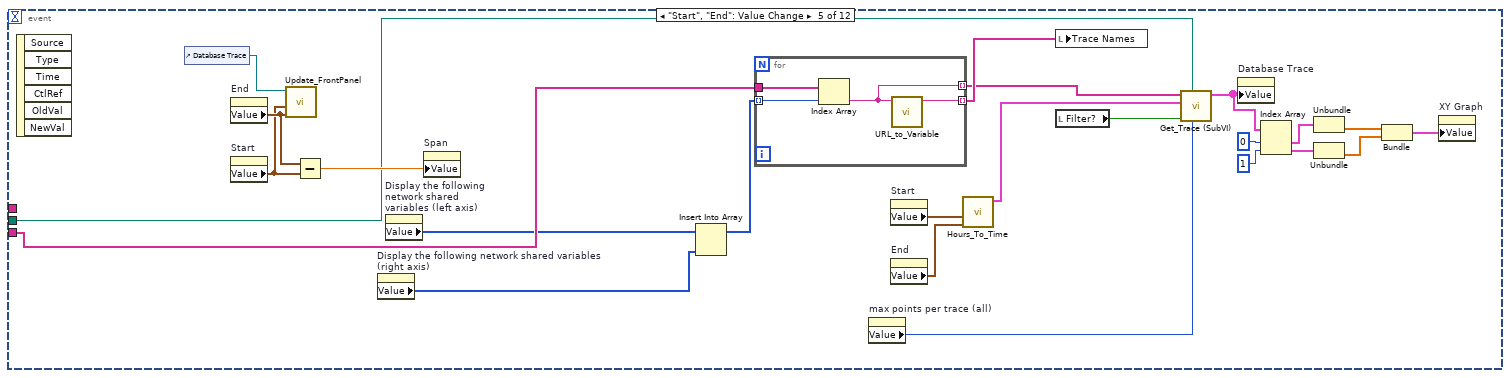
[diagram p7: hidden frame]
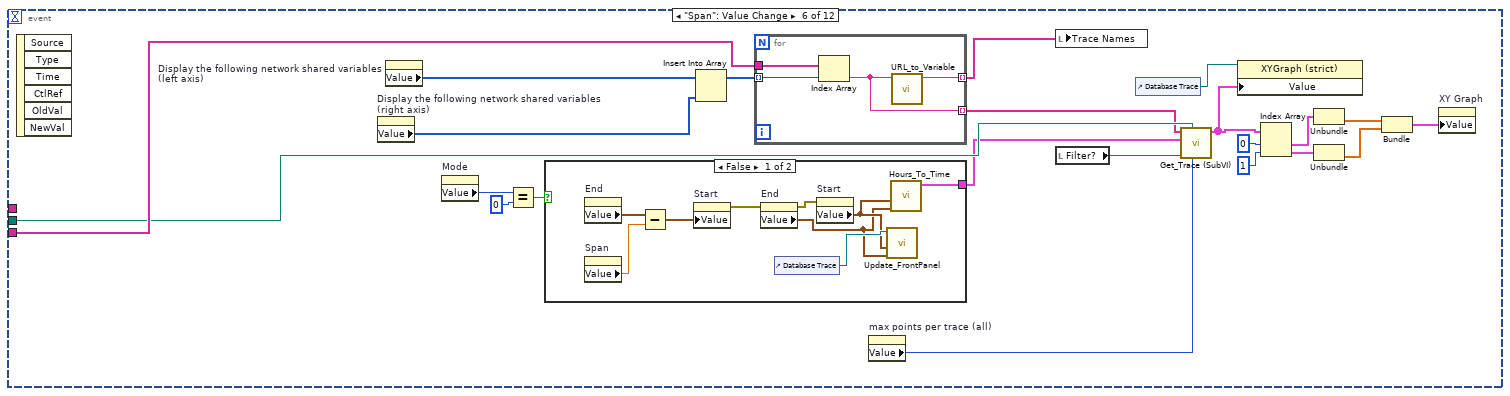
[diagram p8: hidden frame]
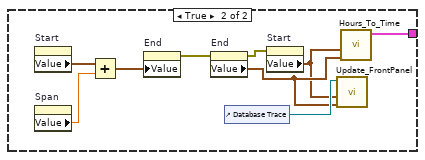
[diagram p9: hidden frame]
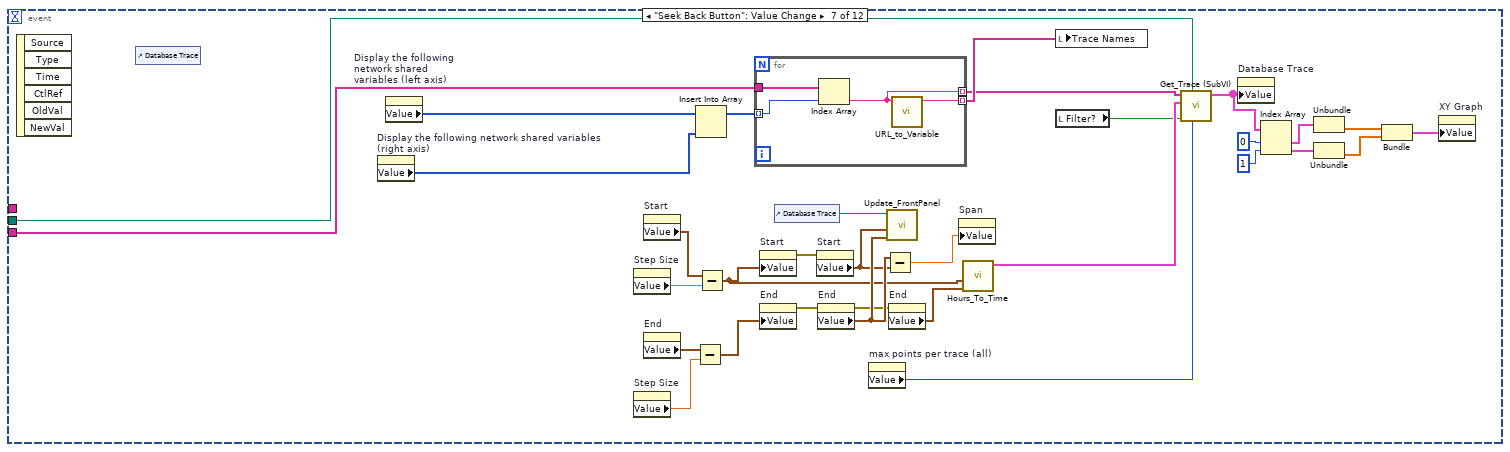
[diagram p10: hidden frame]
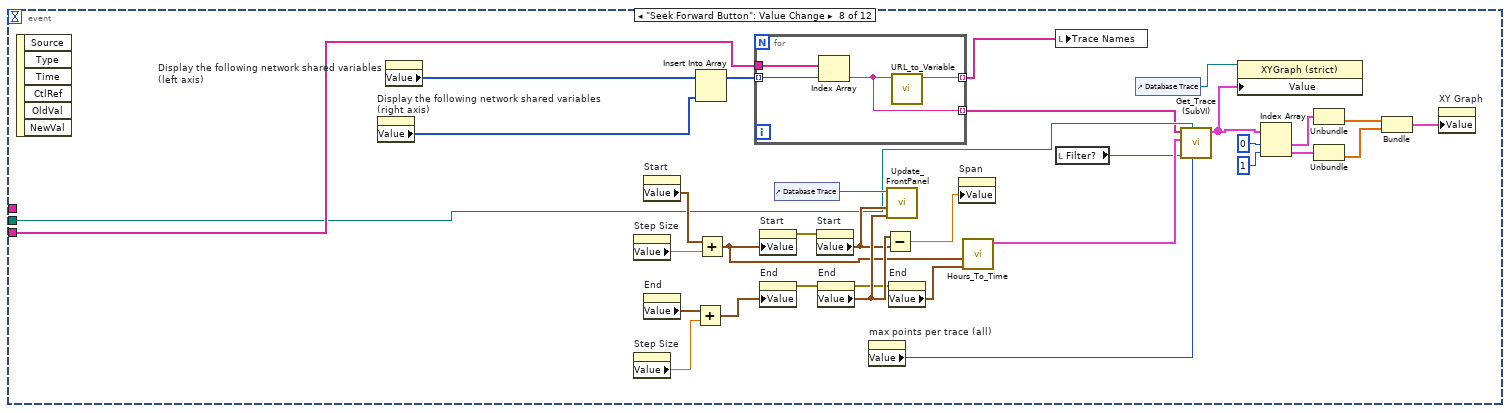
[diagram p11: hidden frame]
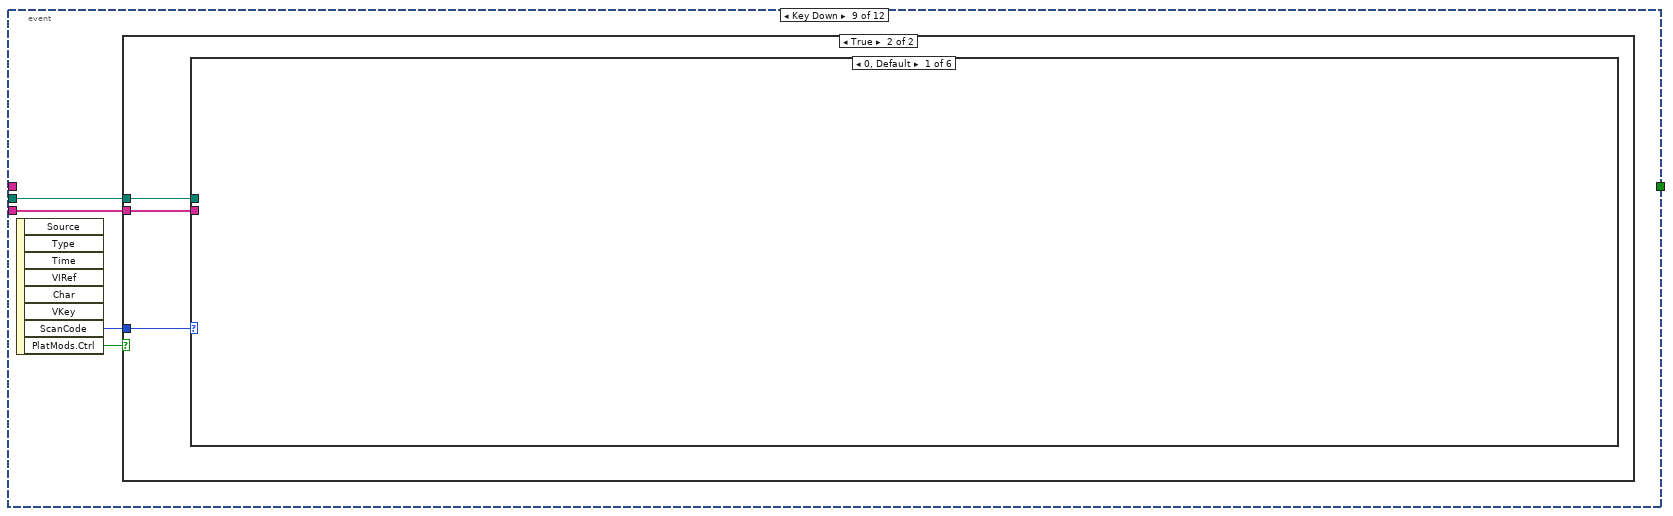
[diagram p12: hidden frame]
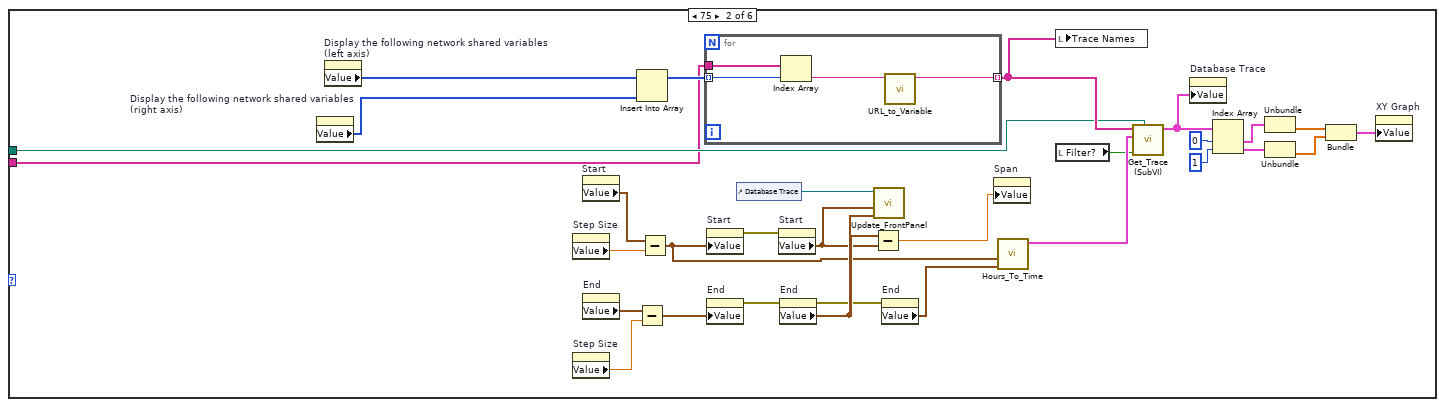
[diagram p14: hidden frame]
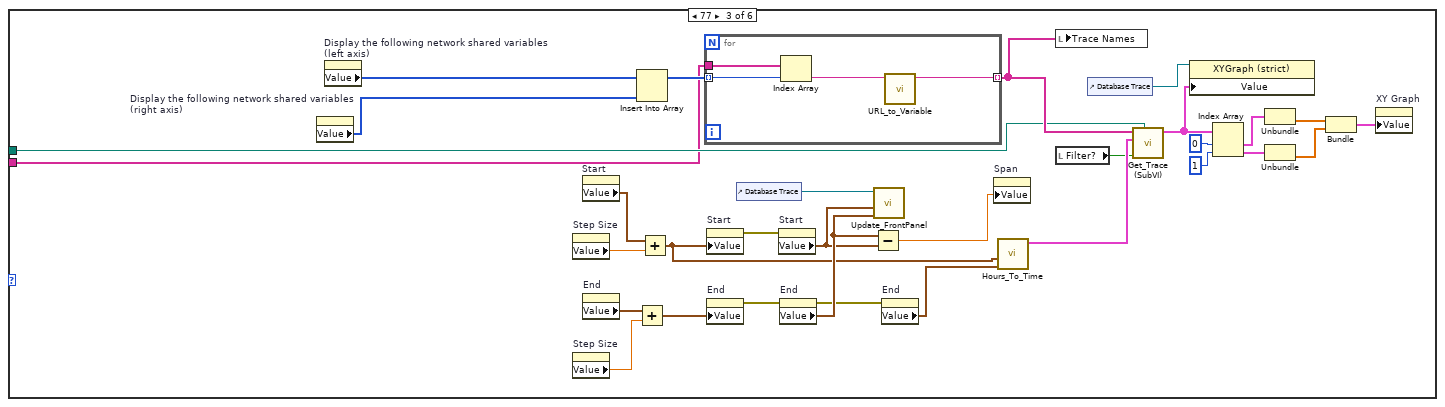
[diagram p15: hidden frame]
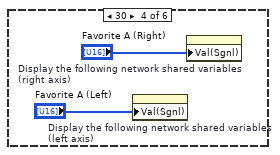
[diagram p16: hidden frame]
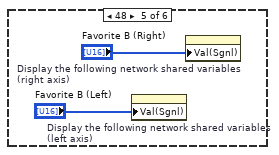
[diagram p17: hidden frame]
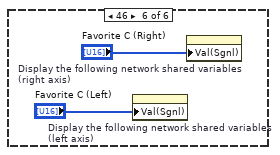
[diagram p18: hidden frame]
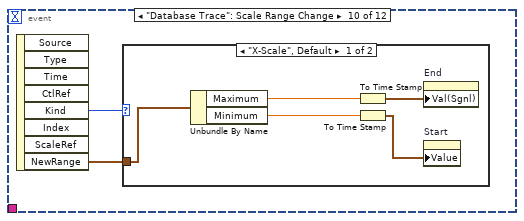
[diagram p19: hidden frame]
diagram:
  # "inbitialize with:\nend = now\nstart = now - 1 hour"
  n1 = property on="max points per trace (all)" class="DigNum (strict)" props=["Value"]() -> ()  [unwired: 2 in, 3 out]
  n2 = Get Date/Time In Seconds() -> (seconds since 1Jan1904=w8:timestamp)
  n3 = call "Get_All_Remote_SV_by_IP.vi"("IP Address"="IP or PC Name") -> ("Shared Variable List"=w15:refnum<k21>[])  [unwired: 8 in, 2 out]
  n4 = local write "End"(w8) -> ()
  n5 = Subtract(x=w8, y=3600.0) -> (x-y=w9:timestamp)
  n6 = for {
    tunnel: [w17] -> w13 mode=indexing
    tunnel: w15 -> [w18] mode=indexing
    tunnel: [w16] -> _ mode=indexing
    n7 = Shared Variable to String(1:w18) -> (0:w17:string)
    n8 = Build Array(w17, w17) -> (w16:string[])
  }
  n9 = local write "Start"(w9) -> ()
  n10 = for {
    tunnel: w13 -> [w27] mode=indexing
    tunnel: [w21] -> w7 mode=indexing
    tunnel: [w20] -> w1 mode=indexing
    tunnel: [w19] -> w4 mode=indexing
    i -> [w22]
    n11 = Match Pattern(string=w27, regular expression="\\\\") -> (after substring=w25:string)  [unwired: 1 in, 3 out]
    n12 = Match Pattern(string=w25, regular expression="\\\\") -> (after substring=w23:string)  [unwired: 1 in, 3 out]
    n13 = Match Pattern(string=w23, regular expression="\\\\") -> (after substring=w19:string)  [unwired: 1 in, 3 out]
    n14 = Build Array(w19, w19) -> (w20:string[])
    n15 = Bundle(w19, w22) -> (w21:cluster{string, i32})  [unwired: 1 in]
  }
  n16 = property on="Which Database?" class="Enum (strict)"() -> ("Value"=w12:enum16{"HousesOfTheHoly", "Rambleon"})  [unwired: 2 in, 2 out]
  n17 = case shown="\"Rambleon\"" w12 {
    tunnel: [path "\\\\HousesoftheHoly\\Default_Database" ("File Path Control") path "\\\\RAMBLEON\\Default_Database" ("File Path Control")] -> w11
    frame "HousesOfTheHoly", Default {
    }
    frame "Rambleon" {
    }
  }
  n18 = property on="Ring" class="Ring (strict)"("StringsAndValues[]"=w7) -> ()  [unwired: 2 in, 2 out]
  n19 = property on="Ring" class="Ring (strict)"("StringsAndValues[]"=w7) -> ()  [unwired: 2 in, 2 out]
  n20 = property on="Ring" class="Ring (strict)"("StringsAndValues[]"=w7) -> ()  [unwired: 2 in, 2 out]
  n21 = property on="Ring" class="Ring (strict)"("StringsAndValues[]"=w7) -> ()  [unwired: 2 in, 2 out]
  n22 = property on="Ring" class="Ring (strict)"("StringsAndValues[]"=w7) -> ()  [unwired: 2 in, 2 out]
  n23 = property on="Ring" class="Ring (strict)"("StringsAndValues[]"=w7) -> ()  [unwired: 2 in, 2 out]
  n24 = property on="Ring" class="Ring (strict)"("StringsAndValues[]"=w7) -> ()  [unwired: 2 in, 2 out]
  n25 = property on="Ring" class="Ring (strict)"("StringsAndValues[]"=w7) -> ()  [unwired: 2 in, 2 out]
  n26 = control-ref of="Tree (Left)"() -> (w6:refnum<vi>)
  n27 = control-ref of="Tree (Right)"() -> (w2:refnum<vi>)
  n28 = while {
    tunnel: w13 -> [w38]
    tunnel: w11 -> [w37]
    tunnel: w4 -> [w31]
    stop <- w32 stop-if-true
    # "Updates the graph if the listbox is clicked"
    n29 = property on="Mode" class="Enum (strict)"() -> ("Value"=w36:T3)  [unwired: 2 in, 2 out]
    n30 = Equal?(x=w36, y=u16 2) -> (x = y?=w34:bool)
    n31 = case shown="True" w34 {
      tunnel: [-1 1] -> w33
      frame False {
      }
      frame True {
      }
    }
    n32 = event shown="[0] Timeout" {
      selector: _ -> [_ _ _ _ _ _ _ _ _ _ _ _]
      dyn-events: _ -> [_ _ _ _ _ _ _ _ _ _ _ _]
      timeout: w33 -> [_ _ _ _ _ _ _ _ _ _ _ _]
      tunnel: w38 -> [w60 w103 _ _ w142 w169 w222 w259 w267 _ _ _]
      tunnel: w37 -> [w61 w97 _ _ w135 w167 w209 w245 w268 _ _ _]
      tunnel: [_ _ _ _ _ _ _ _ _ _ _ w376] -> w32
      tunnel: w31 -> [_ _ w108 w116 _ _ _ _ _ _ _ _]
      event Timeout {
        n33 = event-data() -> ()  [unwired: 1 in, 3 out]
        n34 = property on="Display the following network shared variables (right axis)" class="Arr (strict)"() -> ("Value"=w45:u16[])  [unwired: 2 in, 2 out]
        n35 = property on="Display the following network shared variables (left axis)" class="Arr (strict)"() -> ("Value"=w46:u16[])  [unwired: 2 in, 2 out]
        n36 = Insert Into Array(array=w46, new element=w45) -> (w44:u16[])  [unwired: 1 in]
        n37 = for {
          tunnel: [w68] -> w55 mode=indexing
          tunnel: w60 -> [w69]
          tunnel: w44 -> [w67] mode=indexing
          tunnel: [w66] -> w41 mode=indexing
          n38 = Index Array(array=w69, index=w67) -> (element=w66:string)
          n39 = call "URL_to_Variable.vi"("URL"=w66) -> ("Name"=w68:string)  [unwired: 10 in]
        }
        "Trace Names" <- w55
        n40 = Get Date/Time In Seconds() -> (seconds since 1Jan1904=w59:timestamp)
        n41 = property on="End" class="AbsTime (strict)"("Value"=w59) -> (error out=w58:errorcluster)  [unwired: 2 in, 1 out]
        n42 = control-ref of="Database Trace"() -> (w65:refnum<vi>)
        n43 = property on="max points per trace (all)" class="DigNum (strict)"() -> ("Value"=w43:i32)  [unwired: 2 in, 2 out]
        n44 = property on="End" class="AbsTime (strict)"(error in=w58) -> ("Value"=w57:timestamp)  [unwired: 1 in, 2 out]
        n45 = property on="Start" class="AbsTime (strict)"() -> ("Value"=w56:timestamp)  [unwired: 2 in, 2 out]
        n46 = Subtract(x=w57, y=w56) -> (x-y=w62:dbl)
        n47 = call "Update_FrontPanel.vi"("End"=w57, "Start"=w56, "XYGraph in"=w65) -> ()  [unwired: 9 in]
        n48 = call "Hours_To_Time.vi"("End"=w57, "Start"=w56) -> ("time interval"=w63:T4)  [unwired: 9 in]
        n49 = property on="Span" class="DigNum (strict)"("Value"=w62) -> ()  [unwired: 2 in, 2 out]
        n50 = local read "Filter?"() -> (w42:bool)
        n51 = control-ref of="Database Trace"() -> (w64:refnum<vi>)
        n52 = call "Get_Trace (SubVI).vi"("max points per trace (all)"=w43, "database URL"=w61, "Filter?"=w42, "time interval"=w63, "Array in"=w41) -> ("Array out"=w50:T1)  [unwired: 6 in]
        n53 = property on="Property Node" class="XYGraph (strict)"(reference=w64, "Value"=w50) -> ()  [unwired: 1 in, 2 out]
        n54 = Index Array(array=w50, index #1=0 ("index"), index #2=1 ("index")) -> (element #1=w49:cluster{"timestamps":timestamp[], "data":dbl[]}, element #2=w48:cluster{"timestamps":timestamp[], "data":dbl[]})
        n55 = Unbundle(w49) -> ("data"=w52:dbl[])  [unwired: 1 out]
        n56 = Unbundle(w48) -> ("data"=w51:dbl[])  [unwired: 1 out]
        n57 = Bundle("data"=w52, "data"=w51) -> (w47:cluster{"data":dbl[], "data":dbl[]})  [unwired: 1 in]
        n58 = property on="XY Graph" class="XYGraph (strict)"("Value"=w47) -> ()  [unwired: 2 in, 2 out]
      }
      event "Y Scale.Mapping Mode\n0 = linear; 1 = log", "Display the following network shared variables (left axis)", "Display the following network shared variables (right axis)": Value Change {
        w92 = u32 1 ("Plot.Y Scale Index")
        w89 = 0 ("Active Y Scale")
        n59 = event-data() -> ()  [unwired: 1 in, 6 out]
        n60 = property on="Display the following network shared variables (right axis)" class="Arr (strict)"() -> ("Value"=w79:u16[])  [unwired: 2 in, 2 out]
        n61 = property on="Display the following network shared variables (left axis)" class="Arr (strict)"() -> ("Value"=w72:u16[])  [unwired: 2 in, 2 out]
        n62 = property on="Database Trace" class="XYGraph (strict)"("YScale.Mapping Mode"="Y Scale.Mapping Mode\n0 = linear; 1 = log") -> ()  [unwired: 2 in, 2 out]
        n63 = Array Size(array=w72) -> (size(s)=w77:i32)
        n64 = call "Var_Axis (SubVI).vi"("Value"=w79, "Value 2"=w72) -> ("Value 3"=w80:u16[], "Array"=w78:i32[])  [unwired: 8 in]
        n65 = for {
          tunnel: w103 -> [w107]
          tunnel: w80 -> [w106] mode=indexing
          tunnel: [w105] -> w75 mode=indexing
          tunnel: [w104] -> w70 mode=indexing
          n66 = Index Array(array=w107, index=w106) -> (element=w104:string)
          n67 = call "URL_to_Variable.vi"("URL"=w104) -> ("Name"=w105:string)  [unwired: 10 in]
        }
        n68 = property on="max points per trace (all)" class="DigNum (strict)"() -> ("Value"=w74:i32)  [unwired: 2 in, 2 out]
        n69 = property on="Start" class="AbsTime (strict)"() -> ("Value"=w99:timestamp)  [unwired: 2 in, 2 out]
        n70 = property on="End" class="AbsTime (strict)"() -> ("Value"=w98:timestamp)  [unwired: 2 in, 2 out]
        n71 = control-ref of="Database Trace"() -> (w96:refnum<vi>)
        n72 = call "Hours_To_Time.vi"("End"=w98, "Start"=w99) -> ("time interval"=w102:T4)  [unwired: 9 in]
        n73 = local write "Trace Names"(w75) -> ()
        n74 = local read "Filter?"() -> (w71:bool)
        n75 = Array Size(array=w75) -> (size(s)=w76:i32)
        n76 = control-ref of="Database Trace"() -> (w95:refnum<vi>)
        n77 = property on="Database Trace" class="XYGraph (strict)"("LegNumRows"=w76) -> ()  [unwired: 2 in, 2 out]
        n78 = call "Get_Trace_andUnit (SubVI).vi"("Filter?"=w71, "Array"=w78, "max points per trace (all)"=w74, "time interval"=w102, "database URL"=w97, "Array in"=w70, "XYGraph Refnum"=w96, "XYGraph in"=w96) -> ("Array out"=w81:T1)  [unwired: 3 in]
        n79 = Index Array(array=w75, index #1=0 ("index"), index #2=w77) -> (element #1=w93:string, element #2=w90:string)
        n80 = property on="Database Trace" class="XYGraph (strict)"("Value"=w81) -> ()  [unwired: 2 in, 2 out]
        n81 = property on="Start" class="AbsTime (strict)"() -> ("Value"=w101:timestamp)  [unwired: 2 in, 2 out]
        n82 = property on="End" class="AbsTime (strict)"() -> ("Value"=w100:timestamp)  [unwired: 2 in, 2 out]
        n83 = property on="Property Node" class="XYGraph (strict)"(reference=w95, "YScale.NameLbl.Text"=w90, "Plot.YScaleIdx"=w89, "ActYScl"=w89) -> ()  [unwired: 1 in, 2 out]
        n84 = Index Array(array=w81, index #1=0 ("index"), index #2=1 ("index")) -> (element #1=w84:cluster{"timestamps":timestamp[], "data":dbl[]}, element #2=w83:cluster{"timestamps":timestamp[], "data":dbl[]})
        n85 = property on="Property Node" class="XYGraph (strict)"(reference=w95, "YScale.NameLbl.Text"=w93, "Plot.YScaleIdx"=w92, "ActYScl"=w92, "YScale.Visible"=TRUE ("Y Scale.Visible")) -> ()  [unwired: 1 in, 2 out]
        n86 = call "Update_FrontPanel.vi"("End"=w100, "Start"=w101, "XYGraph in"=w95) -> ()  [unwired: 9 in]
        n87 = Unbundle(w84) -> ("data"=w86:dbl[])  [unwired: 1 out]
        n88 = Unbundle(w83) -> ("data"=w85:dbl[])  [unwired: 1 out]
        n89 = Bundle("data"=w86, "data"=w85) -> (w82:cluster{"data":dbl[], "data":dbl[]})  [unwired: 1 in]
        n90 = property on="XY Graph" class="XYGraph (strict)"("Value"=w82) -> ()  [unwired: 2 in, 2 out]
      }
      event "Tree (Left)": Value Change {
        n91 = event-data() -> ()  [unwired: 1 in, 6 out]
        n92 = property on="Tree (Left)" class="Tree (strict)"() -> ("Value"=w110:string[])  [unwired: 2 in, 2 out]
        n93 = for {
          tunnel: w108 -> [w113]
          tunnel: w110 -> [w112] mode=indexing
          tunnel: [w111] -> w109 mode=indexing
          n94 = Search 1D Array(1D array=w113, element=w112) -> (index of element=w111:i32)  [unwired: 1 in]
        }
        n95 = property on="Display the following network shared variables (left axis)" class="Arr (strict)"("Val(Sgnl)"=w109) -> ()  [unwired: 2 in, 2 out]
      }
      event "Tree (Right)": Value Change {
        n96 = event-data() -> ()  [unwired: 1 in, 6 out]
        n97 = property on="Tree (Right)" class="Tree (strict)"() -> ("Value"=w114:string[])  [unwired: 2 in, 2 out]
        n98 = for {
          tunnel: w116 -> [w119]
          tunnel: w114 -> [w118] mode=indexing
          tunnel: [w117] -> w115 mode=indexing
          n99 = Search 1D Array(1D array=w119, element=w118) -> (index of element=w117:i32)  [unwired: 1 in]
        }
        n100 = property on="Display the following network shared variables (right axis)" class="Arr (strict)"("Val(Sgnl)"=w115) -> ()  [unwired: 2 in, 2 out]
      }
      event "Start", "End": Value Change {
        n101 = event-data() -> ()  [unwired: 1 in, 6 out]
        n102 = control-ref of="Database Trace"() -> (w143:refnum<vi>)
        n103 = property on="End" class="AbsTime (strict)"() -> ("Value"=w137:timestamp)  [unwired: 2 in, 2 out]
        n104 = property on="Start" class="AbsTime (strict)"() -> ("Value"=w136:timestamp)  [unwired: 2 in, 2 out]
        n105 = call "Update_FrontPanel.vi"("End"=w137, "Start"=w136, "XYGraph in"=w143) -> ()  [unwired: 9 in]
        n106 = Subtract(x=w137, y=w136) -> (x-y=w138:dbl)
        n107 = property on="Display the following network shared variables (right axis)" class="Arr (strict)"() -> ("Value"=w124:u16[])  [unwired: 2 in, 2 out]
        n108 = property on="Display the following network shared variables (left axis)" class="Arr (strict)"() -> ("Value"=w126:u16[])  [unwired: 2 in, 2 out]
        n109 = property on="Span" class="DigNum (strict)"("Value"=w138) -> ()  [unwired: 2 in, 2 out]
        n110 = Insert Into Array(array=w126, new element=w124) -> (w125:u16[])  [unwired: 1 in]
        n111 = for {
          tunnel: [w145] -> w134 mode=indexing
          tunnel: w142 -> [w147]
          tunnel: w125 -> [w146] mode=indexing
          tunnel: [w144] -> w120 mode=indexing
          n112 = Index Array(array=w147, index=w146) -> (element=w144:string)
          n113 = call "URL_to_Variable.vi"("URL"=w144) -> ("Name"=w145:string)  [unwired: 10 in]
        }
        n114 = property on="max points per trace (all)" class="DigNum (strict)"() -> ("Value"=w122:i32)  [unwired: 2 in, 2 out]
        n115 = property on="Start" class="AbsTime (strict)"() -> ("Value"=w139:timestamp)  [unwired: 2 in, 2 out]
        n116 = property on="End" class="AbsTime (strict)"() -> ("Value"=w140:timestamp)  [unwired: 2 in, 2 out]
        n117 = call "Hours_To_Time.vi"("End"=w140, "Start"=w139) -> ("time interval"=w141:T4)  [unwired: 9 in]
        n118 = local write "Trace Names"(w134) -> ()
        n119 = local read "Filter?"() -> (w121:bool)
        n120 = call "Get_Trace (SubVI).vi"("max points per trace (all)"=w122, "database URL"=w135, "Filter?"=w121, "time interval"=w141, "Array in"=w120) -> ("Array out"=w123:T1)  [unwired: 6 in]
        n121 = property on="Database Trace" class="XYGraph (strict)"("Value"=w123) -> ()  [unwired: 2 in, 2 out]
        n122 = Index Array(array=w123, index #1=0 ("index"), index #2=1 ("index")) -> (element #1=w129:cluster{"timestamps":timestamp[], "data":dbl[]}, element #2=w128:cluster{"timestamps":timestamp[], "data":dbl[]})
        n123 = Unbundle(w129) -> ("data"=w131:dbl[])  [unwired: 1 out]
        n124 = Unbundle(w128) -> ("data"=w130:dbl[])  [unwired: 1 out]
        n125 = Bundle("data"=w131, "data"=w130) -> (w127:cluster{"data":dbl[], "data":dbl[]})  [unwired: 1 in]
        n126 = property on="XY Graph" class="XYGraph (strict)"("Value"=w127) -> ()  [unwired: 2 in, 2 out]
      }
      event "Span": Value Change {
        n127 = event-data() -> ()  [unwired: 1 in, 6 out]
        n128 = property on="Display the following network shared variables (right axis)" class="Arr (strict)"() -> ("Value"=w151:u16[])  [unwired: 2 in, 2 out]
        n129 = property on="Display the following network shared variables (left axis)" class="Arr (strict)"() -> ("Value"=w153:u16[])  [unwired: 2 in, 2 out]
        n130 = property on="Mode" class="Enum (strict)"() -> ("Value"=w165:T3)  [unwired: 2 in, 2 out]
        n131 = Equal?(x=w165, y=u16 0) -> (x = y?=w163:bool)
        n132 = case shown="False" w163 {
          tunnel: [w171 w182] -> w166
          frame False {
            n133 = property on="End" class="AbsTime (strict)"() -> ("Value"=w176:timestamp)  [unwired: 2 in, 2 out]
            n134 = property on="Span" class="DigNum (strict)"() -> ("Value"=w178:dbl)  [unwired: 2 in, 2 out]
            n135 = Subtract(x=w176, y=w178) -> (x-y=w174:timestamp)
            n136 = property on="Start" class="AbsTime (strict)"("Value"=w174) -> (error out=w175:errorcluster)  [unwired: 2 in, 1 out]
            n137 = property on="End" class="AbsTime (strict)"(error in=w175) -> (error out=w170:errorcluster, "Value"=w172:timestamp)  [unwired: 1 in, 1 out]
            n138 = control-ref of="Database Trace"() -> (w177:refnum<vi>)
            n139 = property on="Start" class="AbsTime (strict)"(error in=w170) -> ("Value"=w173:timestamp)  [unwired: 1 in, 2 out]
            n140 = call "Update_FrontPanel.vi"("End"=w172, "Start"=w173, "XYGraph in"=w177) -> ()  [unwired: 9 in]
            n141 = call "Hours_To_Time.vi"("End"=w172, "Start"=w173) -> ("time interval"=w171:T4)  [unwired: 9 in]
          }
          frame True {
            n142 = property on="Start" class="AbsTime (strict)"() -> ("Value"=w184:timestamp)  [unwired: 2 in, 2 out]
            n143 = property on="Span" class="DigNum (strict)"() -> ("Value"=w185:dbl)  [unwired: 2 in, 2 out]
            n144 = Add(x=w184, y=w185) -> (x+y=w186:timestamp)
            n145 = property on="End" class="AbsTime (strict)"("Value"=w186) -> (error out=w187:errorcluster)  [unwired: 2 in, 1 out]
            n146 = property on="End" class="AbsTime (strict)"(error in=w187) -> (error out=w179:errorcluster, "Value"=w181:timestamp)  [unwired: 1 in, 1 out]
            n147 = control-ref of="Database Trace"() -> (w183:refnum<vi>)
            n148 = property on="Start" class="AbsTime (strict)"(error in=w179) -> ("Value"=w180:timestamp)  [unwired: 1 in, 2 out]
            n149 = call "Update_FrontPanel.vi"("End"=w181, "Start"=w180, "XYGraph in"=w183) -> ()  [unwired: 9 in]
            n150 = call "Hours_To_Time.vi"("End"=w181, "Start"=w180) -> ("time interval"=w182:T4)  [unwired: 9 in]
          }
        }
        n151 = Insert Into Array(array=w153, new element=w151) -> (w152:u16[])  [unwired: 1 in]
        n152 = for {
          tunnel: [w189] -> w162 mode=indexing
          tunnel: w169 -> [w191]
          tunnel: w152 -> [w190] mode=indexing
          tunnel: [w188] -> w148 mode=indexing
          n153 = Index Array(array=w191, index=w190) -> (element=w188:string)
          n154 = call "URL_to_Variable.vi"("URL"=w188) -> ("Name"=w189:string)  [unwired: 10 in]
        }
        n155 = property on="max points per trace (all)" class="DigNum (strict)"() -> ("Value"=w150:i32)  [unwired: 2 in, 2 out]
        n156 = local write "Trace Names"(w162) -> ()
        n157 = local read "Filter?"() -> (w149:bool)
        n158 = control-ref of="Database Trace"() -> (w168:refnum<vi>)
        n159 = call "Get_Trace (SubVI).vi"("max points per trace (all)"=w150, "database URL"=w167, "Filter?"=w149, "time interval"=w166, "Array in"=w148) -> ("Array out"=w154:T1)  [unwired: 6 in]
        n160 = property on="Property Node" class="XYGraph (strict)"(reference=w168, "Value"=w154) -> ()  [unwired: 1 in, 2 out]
        n161 = Index Array(array=w154, index #1=0 ("index"), index #2=1 ("index")) -> (element #1=w157:cluster{"timestamps":timestamp[], "data":dbl[]}, element #2=w156:cluster{"timestamps":timestamp[], "data":dbl[]})
        n162 = Unbundle(w157) -> ("data"=w159:dbl[])  [unwired: 1 out]
        n163 = Unbundle(w156) -> ("data"=w158:dbl[])  [unwired: 1 out]
        n164 = Bundle("data"=w159, "data"=w158) -> (w155:cluster{"data":dbl[], "data":dbl[]})  [unwired: 1 in]
        n165 = property on="XY Graph" class="XYGraph (strict)"("Value"=w155) -> ()  [unwired: 2 in, 2 out]
      }
      event "Seek Back Button": Value Change {
        n166 = event-data() -> ()  [unwired: 1 in, 6 out]
        n167 = control-ref of="Database Trace"() -> ()  [unwired: 1 out]
        n168 = property on="Display the following network shared variables (right axis)" class="Arr (strict)"() -> ("Value"=w198:u16[])  [unwired: 2 in, 2 out]
        n169 = property on="Display the following network shared variables (left axis)" class="Arr (strict)"() -> ("Value"=w199:u16[])  [unwired: 2 in, 2 out]
        n170 = property on="Step Size" class="DigNum (strict)"() -> ("Value"=w211:dbl)  [unwired: 2 in, 2 out]
        n171 = property on="Step Size" class="DigNum (strict)"() -> ("Value"=w210:dbl)  [unwired: 2 in, 2 out]
        n172 = property on="Start" class="AbsTime (strict)"() -> ("Value"=w216:timestamp)  [unwired: 2 in, 2 out]
        n173 = property on="End" class="AbsTime (strict)"() -> ("Value"=w215:timestamp)  [unwired: 2 in, 2 out]
        n174 = Subtract(x=w215, y=w210) -> (x-y=w214:timestamp)
        n175 = Insert Into Array(array=w199, new element=w198) -> (w197:u16[])  [unwired: 1 in]
        n176 = Subtract(x=w216, y=w211) -> (x-y=w207:timestamp)
        n177 = for {
          tunnel: [w225] -> w195 mode=indexing
          tunnel: w222 -> [w227]
          tunnel: w197 -> [w226] mode=indexing
          tunnel: [w224] -> w192 mode=indexing
          n178 = Index Array(array=w227, index=w226) -> (element=w224:string)
          n179 = call "URL_to_Variable.vi"("URL"=w224) -> ("Name"=w225:string)  [unwired: 10 in]
        }
        n180 = property on="Start" class="AbsTime (strict)"("Value"=w207) -> (error out=w213:errorcluster)  [unwired: 2 in, 1 out]
        n181 = property on="End" class="AbsTime (strict)"("Value"=w214) -> (error out=w212:errorcluster)  [unwired: 2 in, 1 out]
        n182 = control-ref of="Database Trace"() -> (w223:refnum<vi>)
        n183 = property on="Start" class="AbsTime (strict)"(error in=w213) -> ("Value"=w217:timestamp)  [unwired: 1 in, 2 out]
        n184 = property on="End" class="AbsTime (strict)"(error in=w212) -> (error out=w208:errorcluster, "Value"=w218:timestamp)  [unwired: 1 in, 1 out]
        n185 = property on="max points per trace (all)" class="DigNum (strict)"() -> ("Value"=w194:i32)  [unwired: 2 in, 2 out]
        n186 = Subtract(x=w218, y=w217) -> (x-y=w219:dbl)
        n187 = call "Update_FrontPanel.vi"("End"=w218, "Start"=w217, "XYGraph in"=w223) -> ()  [unwired: 9 in]
        n188 = property on="End" class="AbsTime (strict)"(error in=w208) -> ("Value"=w220:timestamp)  [unwired: 1 in, 2 out]
        n189 = property on="Span" class="DigNum (strict)"("Value"=w219) -> ()  [unwired: 2 in, 2 out]
        n190 = call "Hours_To_Time.vi"("End"=w220, "Start"=w207) -> ("time interval"=w221:T4)  [unwired: 9 in]
        n191 = local write "Trace Names"(w195) -> ()
        n192 = local read "Filter?"() -> (w193:bool)
        n193 = call "Get_Trace (SubVI).vi"("max points per trace (all)"=w194, "database URL"=w209, "Filter?"=w193, "time interval"=w221, "Array in"=w192) -> ("Array out"=w196:T1)  [unwired: 6 in]
        n194 = property on="Database Trace" class="XYGraph (strict)"("Value"=w196) -> ()  [unwired: 2 in, 2 out]
        n195 = Index Array(array=w196, index #1=0 ("index"), index #2=1 ("index")) -> (element #1=w202:cluster{"timestamps":timestamp[], "data":dbl[]}, element #2=w201:cluster{"timestamps":timestamp[], "data":dbl[]})
        n196 = Unbundle(w202) -> ("data"=w204:dbl[])  [unwired: 1 out]
        n197 = Unbundle(w201) -> ("data"=w203:dbl[])  [unwired: 1 out]
        n198 = Bundle("data"=w204, "data"=w203) -> (w200:cluster{"data":dbl[], "data":dbl[]})  [unwired: 1 in]
        n199 = property on="XY Graph" class="XYGraph (strict)"("Value"=w200) -> ()  [unwired: 2 in, 2 out]
      }
      event "Seek Forward Button": Value Change {
        n200 = event-data() -> ()  [unwired: 1 in, 6 out]
        n201 = property on="Display the following network shared variables (right axis)" class="Arr (strict)"() -> ("Value"=w231:u16[])  [unwired: 2 in, 2 out]
        n202 = property on="Display the following network shared variables (left axis)" class="Arr (strict)"() -> ("Value"=w233:u16[])  [unwired: 2 in, 2 out]
        n203 = property on="Step Size" class="DigNum (strict)"() -> ("Value"=w247:dbl)  [unwired: 2 in, 2 out]
        n204 = property on="Step Size" class="DigNum (strict)"() -> ("Value"=w246:dbl)  [unwired: 2 in, 2 out]
        n205 = property on="Start" class="AbsTime (strict)"() -> ("Value"=w252:timestamp)  [unwired: 2 in, 2 out]
        n206 = property on="End" class="AbsTime (strict)"() -> ("Value"=w251:timestamp)  [unwired: 2 in, 2 out]
        n207 = Add(x=w251, y=w246) -> (x+y=w250:timestamp)
        n208 = Insert Into Array(array=w233, new element=w231) -> (w232:u16[])  [unwired: 1 in]
        n209 = Add(x=w252, y=w247) -> (x+y=w243:timestamp)
        n210 = for {
          tunnel: [w262] -> w242 mode=indexing
          tunnel: w259 -> [w264]
          tunnel: w232 -> [w263] mode=indexing
          tunnel: [w261] -> w228 mode=indexing
          n211 = Index Array(array=w264, index=w263) -> (element=w261:string)
          n212 = call "URL_to_Variable.vi"("URL"=w261) -> ("Name"=w262:string)  [unwired: 10 in]
        }
        n213 = property on="Start" class="AbsTime (strict)"("Value"=w243) -> (error out=w249:errorcluster)  [unwired: 2 in, 1 out]
        n214 = property on="End" class="AbsTime (strict)"("Value"=w250) -> (error out=w248:errorcluster)  [unwired: 2 in, 1 out]
        n215 = control-ref of="Database Trace"() -> (w260:refnum<vi>)
        n216 = property on="Start" class="AbsTime (strict)"(error in=w249) -> ("Value"=w253:timestamp)  [unwired: 1 in, 2 out]
        n217 = property on="End" class="AbsTime (strict)"(error in=w248) -> (error out=w244:errorcluster, "Value"=w254:timestamp)  [unwired: 1 in, 1 out]
        n218 = property on="max points per trace (all)" class="DigNum (strict)"() -> ("Value"=w230:i32)  [unwired: 2 in, 2 out]
        n219 = Subtract(x=w254, y=w253) -> (x-y=w255:dbl)
        n220 = call "Update_FrontPanel.vi"("End"=w254, "Start"=w253, "XYGraph in"=w260) -> ()  [unwired: 9 in]
        n221 = property on="End" class="AbsTime (strict)"(error in=w244) -> ("Value"=w256:timestamp)  [unwired: 1 in, 2 out]
        n222 = property on="Span" class="DigNum (strict)"("Value"=w255) -> ()  [unwired: 2 in, 2 out]
        n223 = call "Hours_To_Time.vi"("End"=w256, "Start"=w243) -> ("time interval"=w257:T4)  [unwired: 9 in]
        n224 = local write "Trace Names"(w242) -> ()
        n225 = local read "Filter?"() -> (w229:bool)
        n226 = control-ref of="Database Trace"() -> (w258:refnum<vi>)
        n227 = call "Get_Trace (SubVI).vi"("max points per trace (all)"=w230, "database URL"=w245, "Filter?"=w229, "time interval"=w257, "Array in"=w228) -> ("Array out"=w234:T1)  [unwired: 6 in]
        n228 = property on="Property Node" class="XYGraph (strict)"(reference=w258, "Value"=w234) -> ()  [unwired: 1 in, 2 out]
        n229 = Index Array(array=w234, index #1=0 ("index"), index #2=1 ("index")) -> (element #1=w237:cluster{"timestamps":timestamp[], "data":dbl[]}, element #2=w236:cluster{"timestamps":timestamp[], "data":dbl[]})
        n230 = Unbundle(w237) -> ("data"=w239:dbl[])  [unwired: 1 out]
        n231 = Unbundle(w236) -> ("data"=w238:dbl[])  [unwired: 1 out]
        n232 = Bundle("data"=w239, "data"=w238) -> (w235:cluster{"data":dbl[], "data":dbl[]})  [unwired: 1 in]
        n233 = property on="XY Graph" class="XYGraph (strict)"("Value"=w235) -> ()  [unwired: 2 in, 2 out]
      }
      event Key Down {
        n234 = event-data() -> ("ScanCode"=w266:i16, "PlatMods.Ctrl"=w265:bool)  [unwired: 1 in, 6 out]
        n235 = case shown="True" w265 {
          tunnel: w268 -> [_ w271]
          tunnel: w267 -> [_ w270]
          tunnel: w266 -> [_ w269]
          frame False {
          }
          frame True {
            n236 = case shown="0, Default" w269 {
              tunnel: w271 -> [_ w274 w308 _ _ _]
              tunnel: w270 -> [_ w273 w307 _ _ _]
              frame 0, Default {
              }
              frame 75 {
                n237 = property on="Display the following network shared variables (right axis)" class="Arr (strict)"() -> ("Value"=w278:u16[])  [unwired: 2 in, 2 out]
                n238 = property on="Display the following network shared variables (left axis)" class="Arr (strict)"() -> ("Value"=w279:u16[])  [unwired: 2 in, 2 out]
                n239 = property on="Step Size" class="DigNum (strict)"() -> ("Value"=w290:dbl)  [unwired: 2 in, 2 out]
                n240 = property on="Step Size" class="DigNum (strict)"() -> ("Value"=w289:dbl)  [unwired: 2 in, 2 out]
                n241 = property on="Start" class="AbsTime (strict)"() -> ("Value"=w295:timestamp)  [unwired: 2 in, 2 out]
                n242 = property on="End" class="AbsTime (strict)"() -> ("Value"=w294:timestamp)  [unwired: 2 in, 2 out]
                n243 = Insert Into Array(array=w279, new element=w278) -> (w277:u16[])  [unwired: 1 in]
                n244 = Subtract(x=w294, y=w289) -> (x-y=w293:timestamp)
                n245 = Subtract(x=w295, y=w290) -> (x-y=w287:timestamp)
                n246 = for {
                  tunnel: [w302] -> w275 mode=indexing
                  tunnel: w273 -> [w305]
                  tunnel: w277 -> [w304] mode=indexing
                  n247 = Index Array(array=w305, index=w304) -> (element=w303:string)
                  n248 = call "URL_to_Variable.vi"("URL"=w303) -> ("Name"=w302:string)  [unwired: 10 in]
                }
                n249 = property on="Start" class="AbsTime (strict)"("Value"=w287) -> (error out=w292:errorcluster)  [unwired: 2 in, 1 out]
                n250 = property on="End" class="AbsTime (strict)"("Value"=w293) -> (error out=w291:errorcluster)  [unwired: 2 in, 1 out]
                n251 = control-ref of="Database Trace"() -> (w301:refnum<vi>)
                n252 = property on="Start" class="AbsTime (strict)"(error in=w292) -> ("Value"=w296:timestamp)  [unwired: 1 in, 2 out]
                n253 = property on="End" class="AbsTime (strict)"(error in=w291) -> (error out=w288:errorcluster, "Value"=w297:timestamp)  [unwired: 1 in, 1 out]
                n254 = Subtract(x=w297, y=w296) -> (x-y=w298:dbl)
                n255 = call "Update_FrontPanel.vi"("End"=w297, "Start"=w296, "XYGraph in"=w301) -> ()  [unwired: 9 in]
                n256 = property on="End" class="AbsTime (strict)"(error in=w288) -> ("Value"=w299:timestamp)  [unwired: 1 in, 2 out]
                n257 = property on="Span" class="DigNum (strict)"("Value"=w298) -> ()  [unwired: 2 in, 2 out]
                n258 = call "Hours_To_Time.vi"("End"=w299, "Start"=w287) -> ("time interval"=w300:T4)  [unwired: 9 in]
                n259 = local write "Trace Names"(w275) -> ()
                n260 = local read "Filter?"() -> (w272:bool)
                n261 = call "Get_Trace (SubVI).vi"("database URL"=w274, "Filter?"=w272, "time interval"=w300, "Array in"=w275) -> ("Array out"=w276:T1)  [unwired: 7 in]
                n262 = property on="Database Trace" class="XYGraph (strict)"("Value"=w276) -> ()  [unwired: 2 in, 2 out]
                n263 = Index Array(array=w276, index #1=0 ("index"), index #2=1 ("index")) -> (element #1=w282:cluster{"timestamps":timestamp[], "data":dbl[]}, element #2=w281:cluster{"timestamps":timestamp[], "data":dbl[]})
                n264 = Unbundle(w282) -> ("data"=w284:dbl[])  [unwired: 1 out]
                n265 = Unbundle(w281) -> ("data"=w283:dbl[])  [unwired: 1 out]
                n266 = Bundle("data"=w284, "data"=w283) -> (w280:cluster{"data":dbl[], "data":dbl[]})  [unwired: 1 in]
                n267 = property on="XY Graph" class="XYGraph (strict)"("Value"=w280) -> ()  [unwired: 2 in, 2 out]
              }
              frame 77 {
                n268 = property on="Display the following network shared variables (right axis)" class="Arr (strict)"() -> ("Value"=w309:u16[])  [unwired: 2 in, 2 out]
                n269 = property on="Display the following network shared variables (left axis)" class="Arr (strict)"() -> ("Value"=w311:u16[])  [unwired: 2 in, 2 out]
                n270 = property on="Step Size" class="DigNum (strict)"() -> ("Value"=w324:dbl)  [unwired: 2 in, 2 out]
                n271 = property on="Step Size" class="DigNum (strict)"() -> ("Value"=w323:dbl)  [unwired: 2 in, 2 out]
                n272 = property on="Start" class="AbsTime (strict)"() -> ("Value"=w329:timestamp)  [unwired: 2 in, 2 out]
                n273 = property on="End" class="AbsTime (strict)"() -> ("Value"=w328:timestamp)  [unwired: 2 in, 2 out]
                n274 = Insert Into Array(array=w311, new element=w309) -> (w310:u16[])  [unwired: 1 in]
                n275 = Add(x=w328, y=w323) -> (x+y=w327:timestamp)
                n276 = Add(x=w329, y=w324) -> (x+y=w321:timestamp)
                n277 = for {
                  tunnel: [w337] -> w320 mode=indexing
                  tunnel: w307 -> [w340]
                  tunnel: w310 -> [w339] mode=indexing
                  n278 = Index Array(array=w340, index=w339) -> (element=w338:string)
                  n279 = call "URL_to_Variable.vi"("URL"=w338) -> ("Name"=w337:string)  [unwired: 10 in]
                }
                n280 = property on="Start" class="AbsTime (strict)"("Value"=w321) -> (error out=w326:errorcluster)  [unwired: 2 in, 1 out]
                n281 = property on="End" class="AbsTime (strict)"("Value"=w327) -> (error out=w325:errorcluster)  [unwired: 2 in, 1 out]
                n282 = control-ref of="Database Trace"() -> (w336:refnum<vi>)
                n283 = property on="Start" class="AbsTime (strict)"(error in=w326) -> ("Value"=w330:timestamp)  [unwired: 1 in, 2 out]
                n284 = property on="End" class="AbsTime (strict)"(error in=w325) -> (error out=w322:errorcluster, "Value"=w331:timestamp)  [unwired: 1 in, 1 out]
                n285 = Subtract(x=w331, y=w330) -> (x-y=w332:dbl)
                n286 = call "Update_FrontPanel.vi"("End"=w331, "Start"=w330, "XYGraph in"=w336) -> ()  [unwired: 9 in]
                n287 = property on="End" class="AbsTime (strict)"(error in=w322) -> ("Value"=w333:timestamp)  [unwired: 1 in, 2 out]
                n288 = property on="Span" class="DigNum (strict)"("Value"=w332) -> ()  [unwired: 2 in, 2 out]
                n289 = call "Hours_To_Time.vi"("End"=w333, "Start"=w321) -> ("time interval"=w334:T4)  [unwired: 9 in]
                n290 = local write "Trace Names"(w320) -> ()
                n291 = local read "Filter?"() -> (w306:bool)
                n292 = control-ref of="Database Trace"() -> (w335:refnum<vi>)
                n293 = call "Get_Trace (SubVI).vi"("database URL"=w308, "Filter?"=w306, "time interval"=w334, "Array in"=w320) -> ("Array out"=w312:T1)  [unwired: 7 in]
                n294 = property on="Property Node" class="XYGraph (strict)"(reference=w335, "Value"=w312) -> ()  [unwired: 1 in, 2 out]
                n295 = Index Array(array=w312, index #1=0 ("index"), index #2=1 ("index")) -> (element #1=w315:cluster{"timestamps":timestamp[], "data":dbl[]}, element #2=w314:cluster{"timestamps":timestamp[], "data":dbl[]})
                n296 = Unbundle(w315) -> ("data"=w317:dbl[])  [unwired: 1 out]
                n297 = Unbundle(w314) -> ("data"=w316:dbl[])  [unwired: 1 out]
                n298 = Bundle("data"=w317, "data"=w316) -> (w313:cluster{"data":dbl[], "data":dbl[]})  [unwired: 1 in]
                n299 = property on="XY Graph" class="XYGraph (strict)"("Value"=w313) -> ()  [unwired: 2 in, 2 out]
              }
              frame 30 {
                n300 = property on="Display the following network shared variables (left axis)" class="Arr (strict)"("Val(Sgnl)"="Favorite A (Left)") -> ()  [unwired: 2 in, 2 out]
                n301 = property on="Display the following network shared variables (right axis)" class="Arr (strict)"("Val(Sgnl)"="Favorite A (Right)") -> ()  [unwired: 2 in, 2 out]
              }
              frame 48 {
                n302 = property on="Display the following network shared variables (left axis)" class="Arr (strict)"("Val(Sgnl)"="Favorite B (Left)") -> ()  [unwired: 2 in, 2 out]
                n303 = property on="Display the following network shared variables (right axis)" class="Arr (strict)"("Val(Sgnl)"="Favorite B (Right)") -> ()  [unwired: 2 in, 2 out]
              }
              frame 46 {
                n304 = property on="Display the following network shared variables (left axis)" class="Arr (strict)"("Val(Sgnl)"="Favorite C (Left)") -> ()  [unwired: 2 in, 2 out]
                n305 = property on="Display the following network shared variables (right axis)" class="Arr (strict)"("Val(Sgnl)"="Favorite C (Right)") -> ()  [unwired: 2 in, 2 out]
              }
            }
          }
        }
      }
      event "Database Trace": Scale Range Change {
        n306 = event-data() -> ("Kind"=w347:enum16{"X-Scale", "Y-Scale", "Z-Scale"}, "NewRange"=w348:T5)  [unwired: 1 in, 6 out]
        n307 = case shown="\"X-Scale\", Default" w347 {
          tunnel: w348 -> [w349 _]
          frame "X-Scale", Default {
            n308 = Unbundle By Name(w349) -> ("Maximum"=w353:dbl, "Minimum"=w351:dbl)
            n309 = To Time Stamp(1:w353) -> (0:w352:timestamp)
            n310 = To Time Stamp(1:w351) -> (0:w350:timestamp)
            n311 = property on="End" class="AbsTime (strict)"("Val(Sgnl)"=w352) -> ()  [unwired: 2 in, 2 out]
            n312 = property on="Start" class="AbsTime (strict)"("Value"=w350) -> ()  [unwired: 2 in, 2 out]
          }
          frame "Y-Scale" {
          }
        }
      }
      event "Export Button": Value Change {
        n313 = event-data() -> ("OldVal"=w354:bool)  [unwired: 1 in, 5 out]
        n314 = local write "Export Button"(w354) -> ()
        n315 = control-ref of="Database Trace"() -> (w359:refnum<vi>)
        n316 = property on="Property Node" class="XYGraph (strict)"(reference=w359) -> ("Value"=w360:T1)  [unwired: 1 in, 2 out]
        n317 = for {
          tunnel: w360 -> [w370] mode=indexing
          tunnel: [w367] -> w358 mode=indexing
          n318 = case shown="True" "Igor" {
            tunnel: [0.0 w372] -> w361
            frame False {
            }
            frame True {
              n319 = case shown="True" "DST" {
                tunnel: [-5.0 -4.0] -> w372
                frame False {
                }
                frame True {
                }
              }
            }
          }
          "Shift Hours" <- w361
          n320 = Unbundle(w370) -> ("timestamps"=w369:timestamp[], "data"=w368:dbl[])
          n321 = Multiply(x=w361, y=3600.0) -> (x*y=w364:dbl)
          n322 = To Double Precision Float(number=w369) -> (double precision float=w366:dbl[])
          n323 = Add(x=w364, y=w366) -> (x+y=w365:dbl[])
          n324 = Bundle(w365, "data"=w368) -> (w367:cluster{dbl[], "data":dbl[]})  [unwired: 1 in]
        }
        n325 = local read "Trace Names"() -> (w357:string[])
        n326 = call <userlib>:"LV to ITX XY AutoPlot.vi"("filename"="export", "path"="path", "XY Array"=w358, "wavenames (.Vx, etc)"=w357) -> ()  [unwired: 11 in, 1 out]
      }
      event "Stop Button": Value Change {
        n327 = event-data() -> ("OldVal"=w377:bool, "NewVal"=w376:bool)  [unwired: 1 in, 4 out]
        n328 = local write "Stop Button"(w377) -> ()
      }
    }
  }
  n329 = call <userlib>:"MGI Populate Tree with Delimited Strings.vi"("Delimiter"="\\", "Items (Delimited)"=w1, "Tree Control"=w6) -> ()  [unwired: 6 in, 3 out]
  n330 = call <userlib>:"MGI Populate Tree with Delimited Strings.vi"("Delimiter"="\\", "Items (Delimited)"=w1, "Tree Control"=w2) -> ()  [unwired: 6 in, 3 out]
